vi "MC_8_27_12a_JW.vi"() -> ()   [LabVIEW 2011]
uses:
  <vilib>/Utility/file.llb/Read From Spreadsheet File (string).vi
  <vilib>/Utility/inputDevices.llb/keyboardAcquire.vi
  <vilib>/Utility/file.llb/Write To Spreadsheet File (DBL).vi
  <vilib>/Utility/file.llb/Write To Spreadsheet File (string).vi
  <vilib>/regexp/Match Regular Expression.xnode
panel:
  in  "Treatment Concentration (mM):":dbl=nan
  in  "Surface Treatment:":string="NaN"
  in  "# Drops*:":dbl=inf
  in  "Solution Temp (C):":dbl=nan
  in  "Relative Humidity (%):":dbl=nan
  in  "Room Temp (F):":dbl=nan
  in  "Time (s):":dbl=nan
  in  "RPM:":dbl=nan
  in  "Wait Time (s):":dbl=nan
  in  "Sample #:":dbl=1.0
  in  "Fabricator:":string="NaN"
  in  "Ramp (s):":dbl=3.0
  out "X Axis Display Type":string
  out "Opj X Axis":string
  in  "Room Temp":dbl=294.0
  out "No Image 2":path=path "\\\\acad1\\physics/Jurchescu-group/JW-PD/Image Not Found.png"
  out "Save1 Array":string[][](array[string])
  out "Lin Vd":dbl
  out "Lin-Vg Array-Used":dbl[](array[numeric])
  out "Lin Id-Used":dbl[](array[numeric])
  out "Rec: Comments":string
  out "Folder Index":dbl caption="Length"
  out "Current \nRecord":string[](array[string])
  out "Transformer \nHeaders":string[](array[string])
  out "Current Device ID":string
  out "Column":string
  out "Row":string
  out "Rec: Concentration":dbl
  out "Rec: Solvent":string
  out "Rec: Method":string
  in  "?":T1(tab)
  in  "Transport File":path
  out "Transport Folder":path
  out "Rec: Material":string
  out "Accel (RPM/s):":dbl
  in  "Transfer File":path
  out "Transfer Folder":path
  in  "Image Folder":path
  out "Image File":path=path "D:/UserData/Desktop/Jeremy/WFU/Research/Programs/VI mods/Image Not Found.png"
  in  "Manual Comments":bool
  in  "Comments:":string
  out "Calc: On/Off":dbl caption="On/Off-Sat" format="%#.2e"
  out "Calc: Off I-Sat":dbl caption="Off I-Sat" format="%#.2e"
  in  "Manuel-Dielectric":bool
  in  "Manuel-Length":bool
  out "Calc: VT-Lin":dbl
  out "New: VT-Lin":dbl
  out "Rec: VT-Lin":dbl caption="VT-Lin" format="%#_3g"
  out "Calc: Trap Density-STS":dbl format="%#.2e"
  out "New: Trap Density-STS":dbl format="%#.2e"
  out "Rec: Trap Density-STS":dbl caption="N-Sat (STS)" format="%#.2e"
  out "Calc: Trap Density-VT":dbl format="%#.2e"
  out "New: Trap Density-VT":dbl format="%#.2e"
  out "Rec: Trap Density-VT":dbl caption="N-Sat (VT)" format="%#.2e"
  out "Calc: Mobility-Lin":dbl format="%#.2e"
  out "New: Mobility-Lin":dbl format="%#_4e"
  out "Rec: Mobility-Lin":dbl caption="Mobility-Lin" format="%#_3e"
  out "Calc: Mobility-Sat":dbl format="%#.2e"
  out "Rec: Length":dbl caption="Length" format="%#_3g"
  out "Rec: Width":dbl caption="Width" format="%#_4g"
  out "Rec: Dielectric (d)":dbl caption="Dielectric (d)" format="%#_3g"
  in  "Cancel Button":bool
  in  "Up Button":bool
  in  "Down Button":bool
  out "Data Name:":string
  in  "Save Changes?":bool
  in  "New: Dielectric":dbl
  in  "New: Length":dbl
  in  "New: Width":dbl
  out "New: Mobility-Sat":dbl format="%#.2e"
  in  "Blank Button":bool
  in  "Zoom":i16(slide)=-3 scale=-5.0..5.0
  out "Image Out 2":T2(plugin-control)
  out "Image Out":T2(plugin-control)
  in  "Magnification":u16(ring) items=["5x", "10x", "20x", "50x", "80x"]
  out "Total Width":dbl
  out "Distances":dbl[](array[numeric])
  in  "Undo Button":bool
  in  "Remove Button":bool
  out "Rec: Mobility-Sat":dbl caption="Mobility-Sat" format="%#.2e"
  in  "Export":bool
  out "Calc: VT-Sat":dbl format="%#.2g"
  out "New: VT-Sat":dbl format="%#.2g"
  in  "Manual-Width":bool caption="Manual"
  out "Calc: STS":dbl format="%#.2g"
  out "New: STS":dbl format="%#.2g"
  out "Rec: VT-Sat":dbl caption="VT-Sat" format="%#.2g"
  out "Rec: STS":dbl caption="STS-Sat" format="%#.2g"
  out "Rec: On/Off":dbl caption="On/Off-Sat" format="%#.2e"
  in  "Save Changes? 2":bool
  in  "Save Changes? 3":bool
  out "Rec: Temp":dbl caption="Sample Temp" format="%.1f"
  in  "New: Temp":dbl format="%.1f"
  out "Rec: Off I-Sat":dbl caption="Off I-Sat" format="%#.2e"
  in  "Independant Variable":string(combo)="Length (um):"
  in  "Transfer Plots":enum32{"Linear", "Saturation", "Raw"}(tab)=enum."Saturation"
  in  "Lin-Trans Slider":dbl(slide) step=1.0 scale=-22.0..89.0 scale format="%#_1p"
  out "Sqrt-Lin":cluster{dbl[], dbl[]}[](graph)
  in  "Next Sqrt Lin":bool
  in  "Previous Sqrt Lin":bool
  in  "Sat-Trans Slider":dbl(slide) step=1.0 scale=-22.0..89.0 scale format="%#_1p"
  out "Sqrt-Sat":cluster{dbl[], dbl[]}[](graph)
  in  "Previous Sqrt Sat":bool
  in  "Next Sqrt Sat":bool
  out "Sqrt-Raw":cluster{dbl[], dbl[]}[](graph)
  in  "Log Plots":enum32{"Linear", "Saturation", "Raw"}(tab)=enum."Saturation"
  in  "Lin-Log Slider":dbl(slide) step=1.0 scale=-1.0..82.0 scale format="%#_1p"
  in  "Previous Log Lin":bool
  in  "Next Log Lin":bool
  out "Log-Lin":cluster{dbl[], dbl[]}[](graph)
  in  "Sat-Log Slider":dbl(slide) step=1.0 scale=-1.0..82.0 scale format="%#_1p"
  out "Log-Sat":cluster{dbl[], dbl[]}[](graph)
  in  "Previous Log Sat":bool
  in  "Next Log Sat":bool
  out "Raw-Log":cluster{dbl[], dbl[]}[](graph)
  in  "Manual-Temp":bool caption="Manual"
  out "Date Created":string caption="Fabricated"
  out "Date Recorded":string="Date Recorded" caption="Measured"
  out "Image Name":string
  out "Index":string
  in  "Num Pts":dbl=5.0
  in  "NumPoints Log":dbl=5.0 caption="Num Pts"
  in  "Origin Project File":path=path "\\\\acad1\\physics/Jurchescu-group/JW-PD/Group Library/Origin Project Files/DeviceData_8_10_12a_JW.opj"
  in  "No Image File":path=path "\\\\acad1\\physics/Jurchescu-group/JW-PD/Mega Awesome/Image Not Found.png"
  out "String":string
  out "Index 2":dbl
  out "Sat Id-Log-Used":dbl[](array[numeric])
  out "Vg Array-Log-Used":dbl[](array[numeric])
  out "ROI Descriptor out":T3 {"Contours"."Type" items=["No Selection", "Point", "Line", "Rectangle", "Oval", "Polygon", "Freehand Region", "Annulus", "Unused2", "Unused3", "Broken Line", "Freehand Line", "Rotated Rectangle"]}
  out "ROI Descriptor":T3 {"Contours"."Type" items=["No Selection", "Point", "Line", "Rectangle", "Oval", "Polygon", "Freehand Region", "Annulus", "Unused2", "Unused3", "Broken Line", "Freehand Line", "Rotated Rectangle"]}
  out "Numeric 3":dbl
  out "Array 6":dbl[][](array[numeric])
  out "Cluster":T4
  out "Array 5":dbl[](array[numeric])
  out "Array 4":dbl[](array[numeric])
  out "Array 3":dbl[](array[numeric])
  out "Numeric 2":dbl
  out "Numeric":dbl
  out "Sat Id-Used":dbl[](array[numeric])
  out "Sat Vg Array-Used":dbl[](array[numeric])
  out "MobVi Index":dbl
  in  "Row Start":dbl=20.0
  # "Sample Properties"
  # "*     Inf = Full coverage\n   NaN = Unknown or Not Applicable"
  # "Data Locations"
  # "Transport Location"
  # "Transfer Location"
  # "Image Location"
  # "Recorded"
  # "Calculated"
  # "Re-Calculated"
  # "Manual"
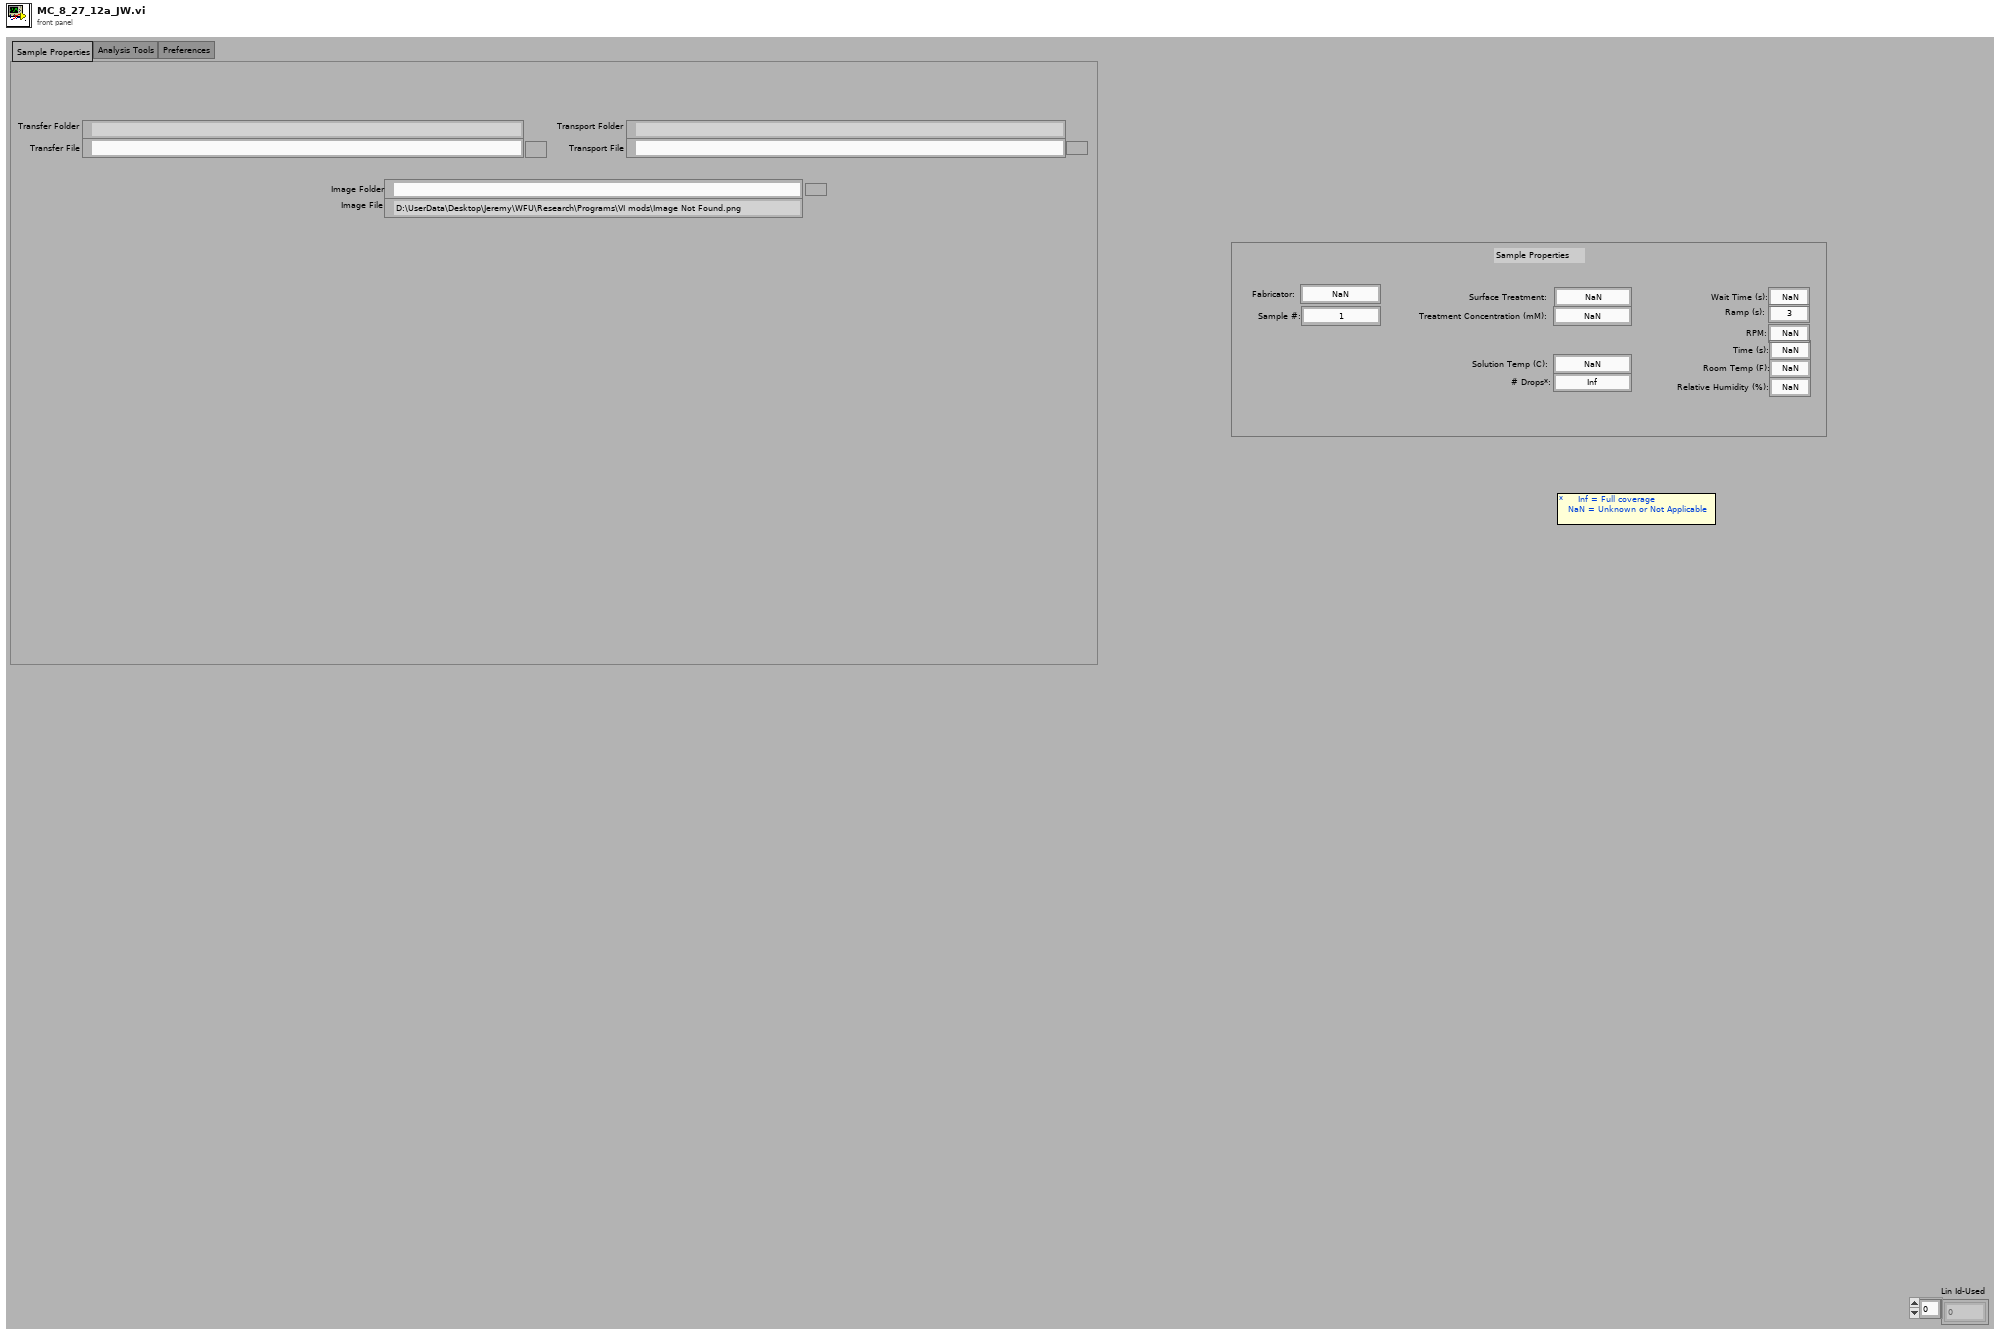
[diagram p1: front panel]
types:
  T1 = enum32{"Sample Properties", "Analysis Tools", "Preferences", "Current Database"}
  T2 = typedef "IMAQ Image.ctl" = refnum<image>
  T3 = typedef "ROI Descriptor" = cluster{"Global Rectangle":i32[], "Contours":cluster{"ID":enum32{"External", "Internal"}, "Type":u32, "Coordinates":i32[]}[]}
  T4 = cluster{"Numeric":dbl, "Numeric 2":dbl, "Numeric 3":dbl, "Numeric 4":dbl}
  T5 = cluster{"Mobility-Sat":dbl, "Moblitity-Lin":dbl, "On/Off":dbl, "Off Current":dbl, "Vt-Sat":dbl, "STS":dbl, "Trap Density-VT":dbl, "Trap Density-STS":dbl}
  T6 = cluster{"Date Recorded":string, "Index":string, "Length":dbl, "Width":dbl, "Sample Temp":dbl}
  T7 = cluster{"Date Created":string, "Material":string, "Solvent":string, "Concentration":dbl, "Method":string, "Dielectric (nm)":dbl, "Treatment":string, "Comments":string}
  T8 = cluster{"Raw Sat":cluster{dbl[], dbl[]}[], "Sqrt Sat":cluster{dbl[], dbl[]}[], "Log Sat":cluster{dbl[], dbl[]}, "Raw Lin":cluster{dbl[], dbl[]}[], "Sqrt Lin":cluster{dbl[], dbl[]}[], "Log Lin":cluster{dbl[], dbl[]}[]}
  T9 = cluster{"Mobility-Sat":dbl, "Vt-Sat":dbl, "Mobility-Lin":dbl, "Vt-Lin":dbl, "Off I-Sat":dbl, "On/Off I-Sat":dbl}
  T10 = cluster{"[0]":cluster{dbl[], dbl[]}, "[1]":cluster{dbl[], dbl[]}, "[2]":cluster{dbl[], dbl[]}, "[3]":cluster{dbl[], dbl[]}, "[4]":cluster{dbl[], dbl[]}, "[5]":cluster{dbl[], dbl[]}, "[6]":cluster{dbl[], dbl[]}, "[7]":cluster{dbl[], dbl[]}, "[8]":cluster{dbl[], dbl[]}}
  T11 = cluster{"Global Rectangle":i32[], "Contours":cluster{"Contour Type":u32, "ROI Type":u32, "Points":i32[]}[]}
  T12 = typedef "LVBoundsTypeDef.ctl" = cluster{"Width":u32, "Height":u32}
  T13 = enum16{"0", "1", "2", "3", "4", "5", "6", "7", "8", "9", "A", "B", "C", "D", "E", "F", "G", "H", "I", "J", "K", "L", "M", "N", "O", "P", "Q", "R", "S", "T", "U", "V", "W", "X", "Y", "Z", "F1", "F2", "F3", "F4", "F5", "F6", "F7", "F8", "F9", "F10", "F11", "F12", "F13", "F14", "F15", "ADD", "BACK", "BACKSLASH", "CAPITAL", "COMMA", "DECIMAL", "DELETE", "DIVIDE", "DOWN", "END", "EQUALS", "ESCAPE", "GRAVE (`)", "HOME", "INSERT", "LBRACKET", "LCONTROL", "LEFT", "L ALT", "LSHIFT", "LWIN", "MINUS", "MULTIPLY", "NEXT", "NUMLOCK", "NUMPAD_0", "NUMPAD_1", "NUMPAD_2", "NUMPAD_3", "NUMPAD_4", "NUMPAD_5", "NUMPAD_6", "NUMPAD_7", "NUMPAD_8", "NUMPAD_9", "PAUSE", "PERIOD", "PRIOR (PG UP)", "RBRACKET", "RCONTROL", "RETURN", "RIGHT", "R ALT", "RSHIFT", "RWIN", "SCROLL", "SEMICOLON", "SLASH", "SPACE", "SUBTRACT", "TAB", "UP", "ENTER (num pad)", "' (quote)"}[]
  T14 = enum16{"0", "1", "2", "3", "4", "5", "6", "7", "8", "9", "A", "B", "C", "D", "E", "F", "G", "H", "I", "J", "K", "L", "M", "N", "O", "P", "Q", "R", "S", "T", "U", "V", "W", "X", "Y", "Z", "F1", "F2", "F3", "F4", "F5", "F6", "F7", "F8", "F9", "F10", "F11", "F12", "F13", "F14", "F15", "ADD", "BACK", "BACKSLASH", "CAPITAL", "COMMA", "DECIMAL", "DELETE", "DIVIDE", "DOWN", "END", "EQUALS", "ESCAPE", "GRAVE (`)", "HOME", "INSERT", "LBRACKET", "LCONTROL", "LEFT", "L ALT", "LSHIFT", "LWIN", "MINUS", "MULTIPLY", "NEXT", "NUMLOCK", "NUMPAD_0", "NUMPAD_1", "NUMPAD_2", "NUMPAD_3", "NUMPAD_4", "NUMPAD_5", "NUMPAD_6", "NUMPAD_7", "NUMPAD_8", "NUMPAD_9", "PAUSE", "PERIOD", "PRIOR (PG UP)", "RBRACKET", "RCONTROL", "RETURN", "RIGHT", "R ALT", "RSHIFT", "RWIN", "SCROLL", "SEMICOLON", "SLASH", "SPACE", "SUBTRACT", "TAB", "UP", "ENTER (num pad)", "' (quote)"}
  T15 = cluster{"Contour Type":u32, "ROI Type":u32, "Points":i32[]}[]
  T16 = cluster{i32[], cluster{"Contour Type":u32, "ROI Type":u32, "Points":i32[]}[]}
  T17 = cluster{"Independant  Variable Indicator":string, "Parameter String Indicator":string}
  T18 = cluster{string, sgl, bool, bool, bool, bool, bool, bool, i32}
  T19 = cluster{i32, cluster{string, sgl, bool, bool, bool, bool, bool, bool, i32}, i32, i32}
  T20 = cluster{"Contour Type":u32, "ROI Type":u32, "Points":i32[]}
  T21 = cluster{"Points[0]":i32, "Points[1]":i32, "Points[2]":i32, "Points[3]":i32, "Points[4]":i32, "Points[5]":i32, "Points[6]":i32, "Points[7]":i32, "Points[8]":i32}
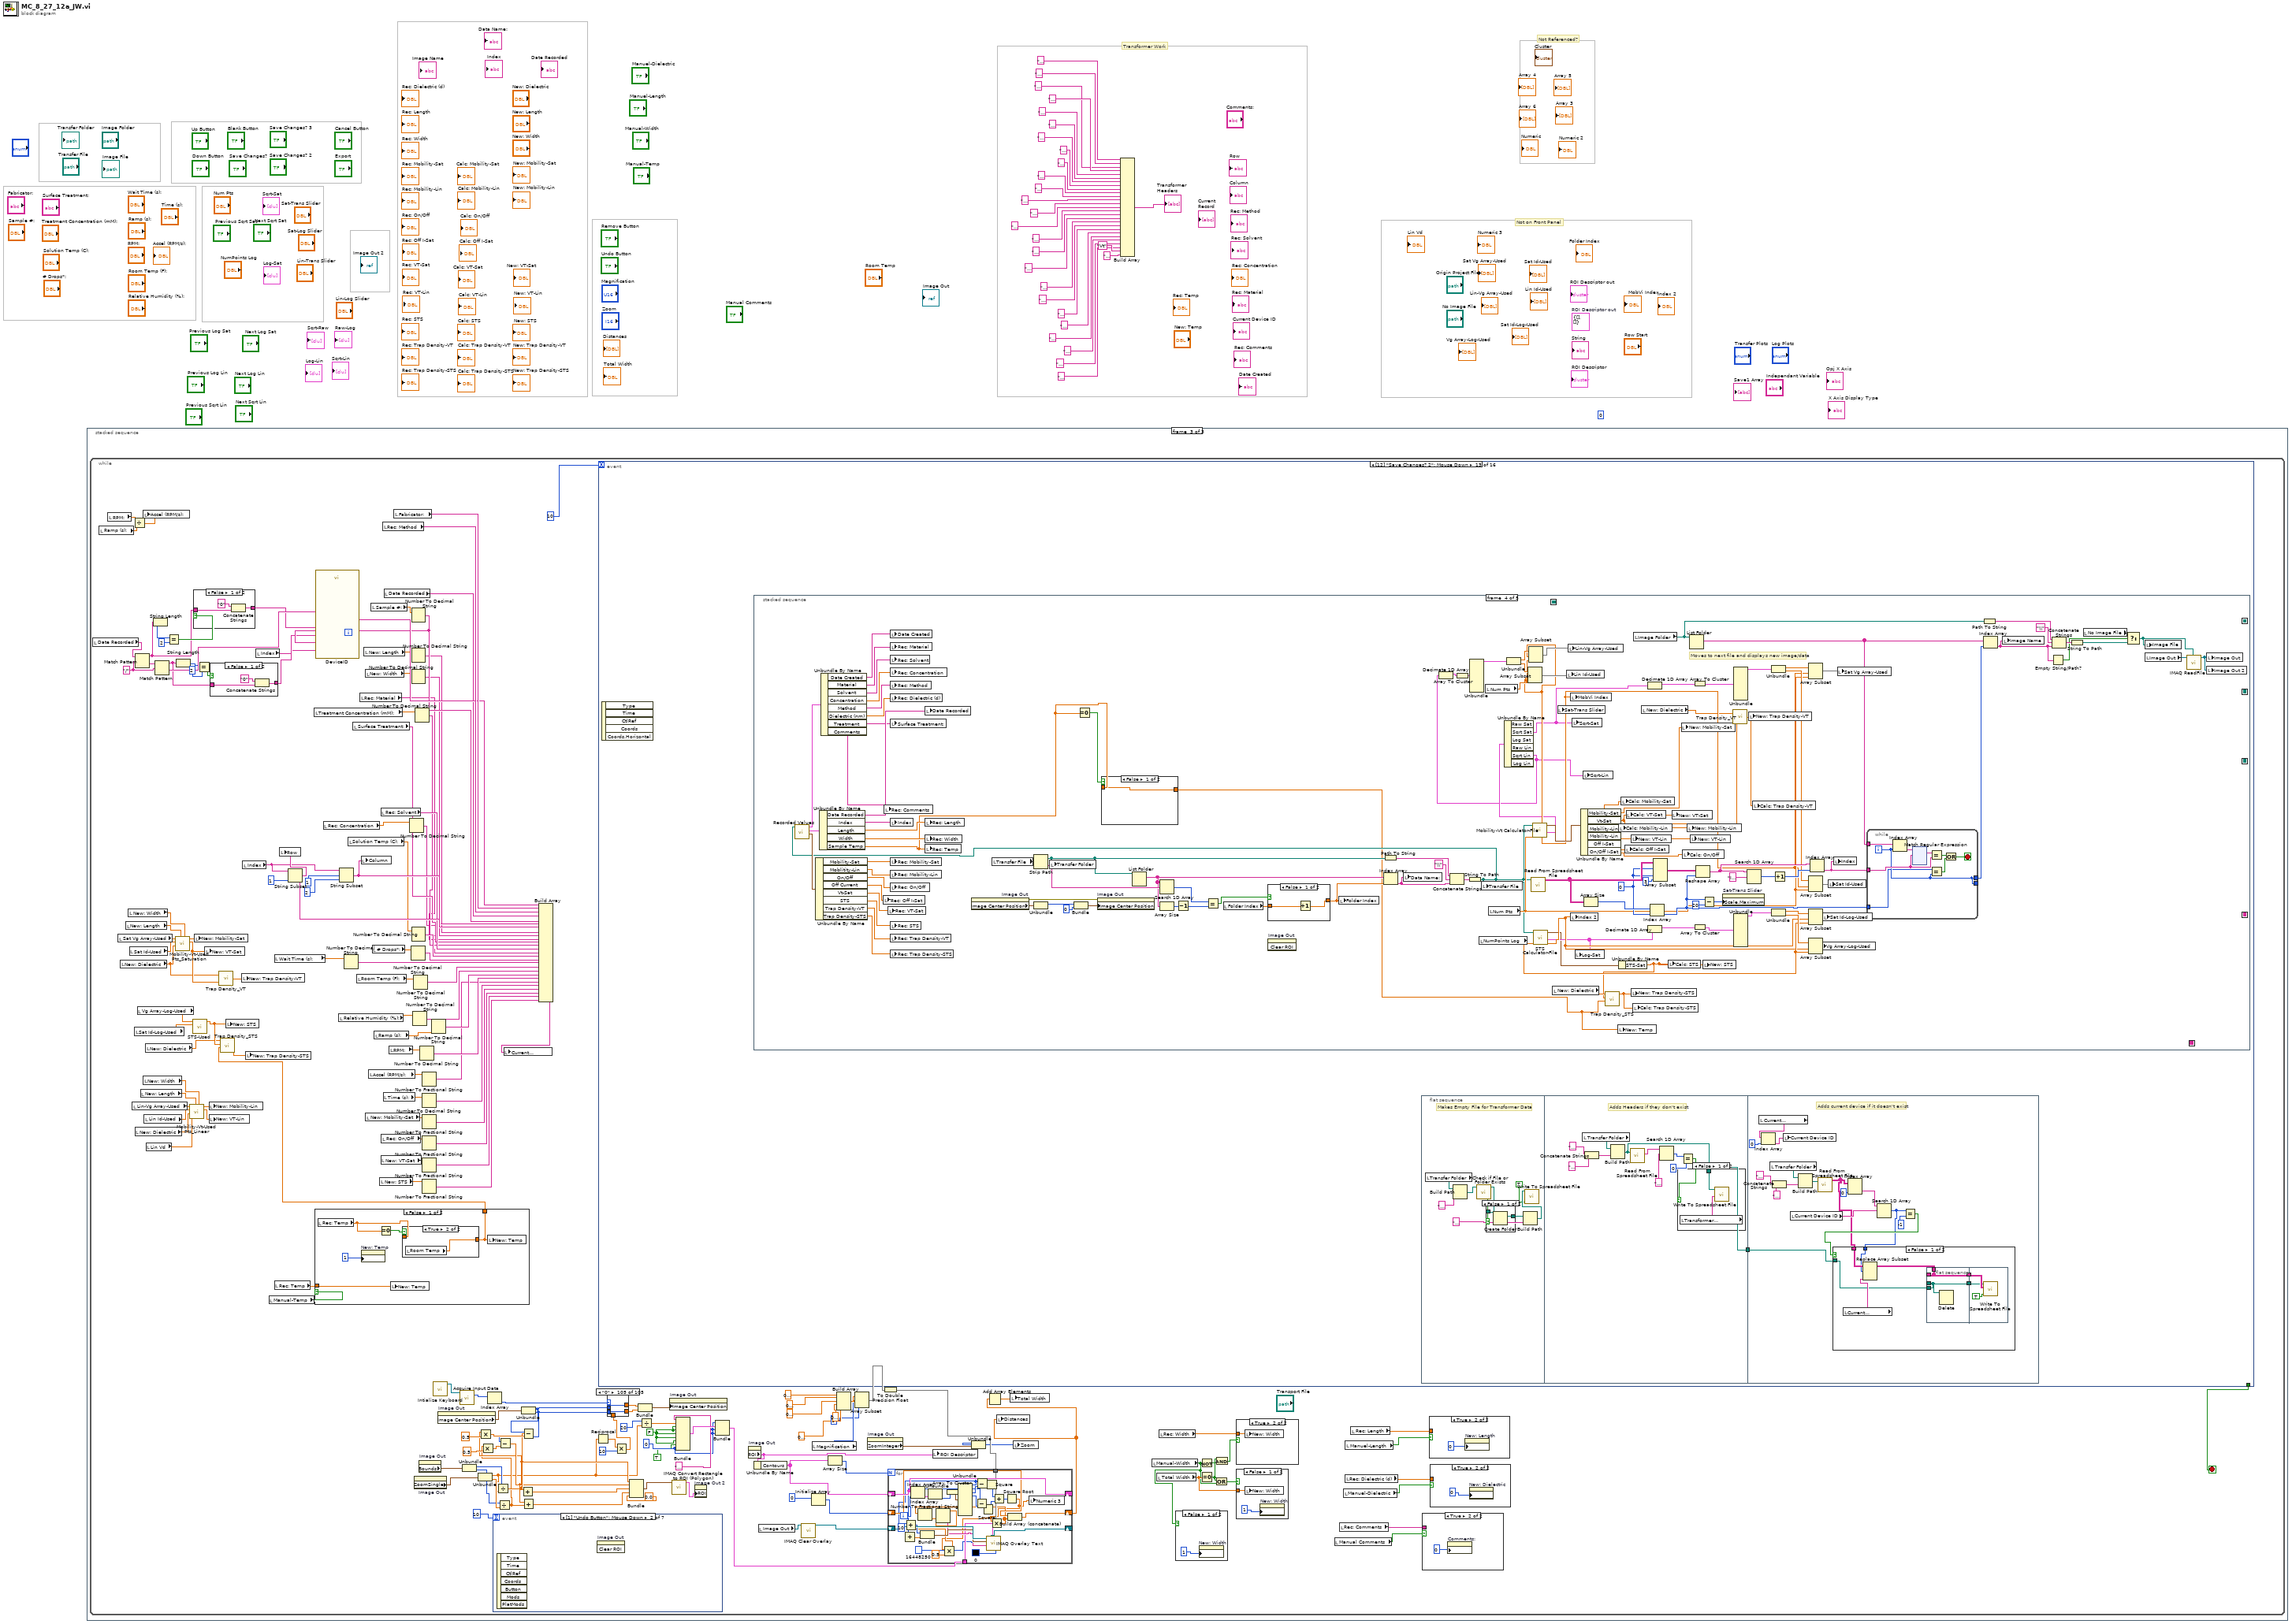
[diagram p0: block diagram]
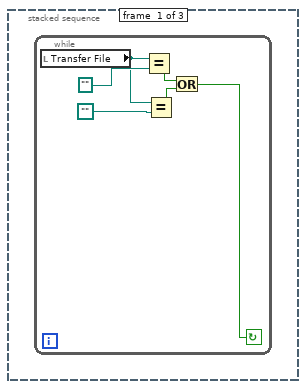
[diagram p2: hidden frame]
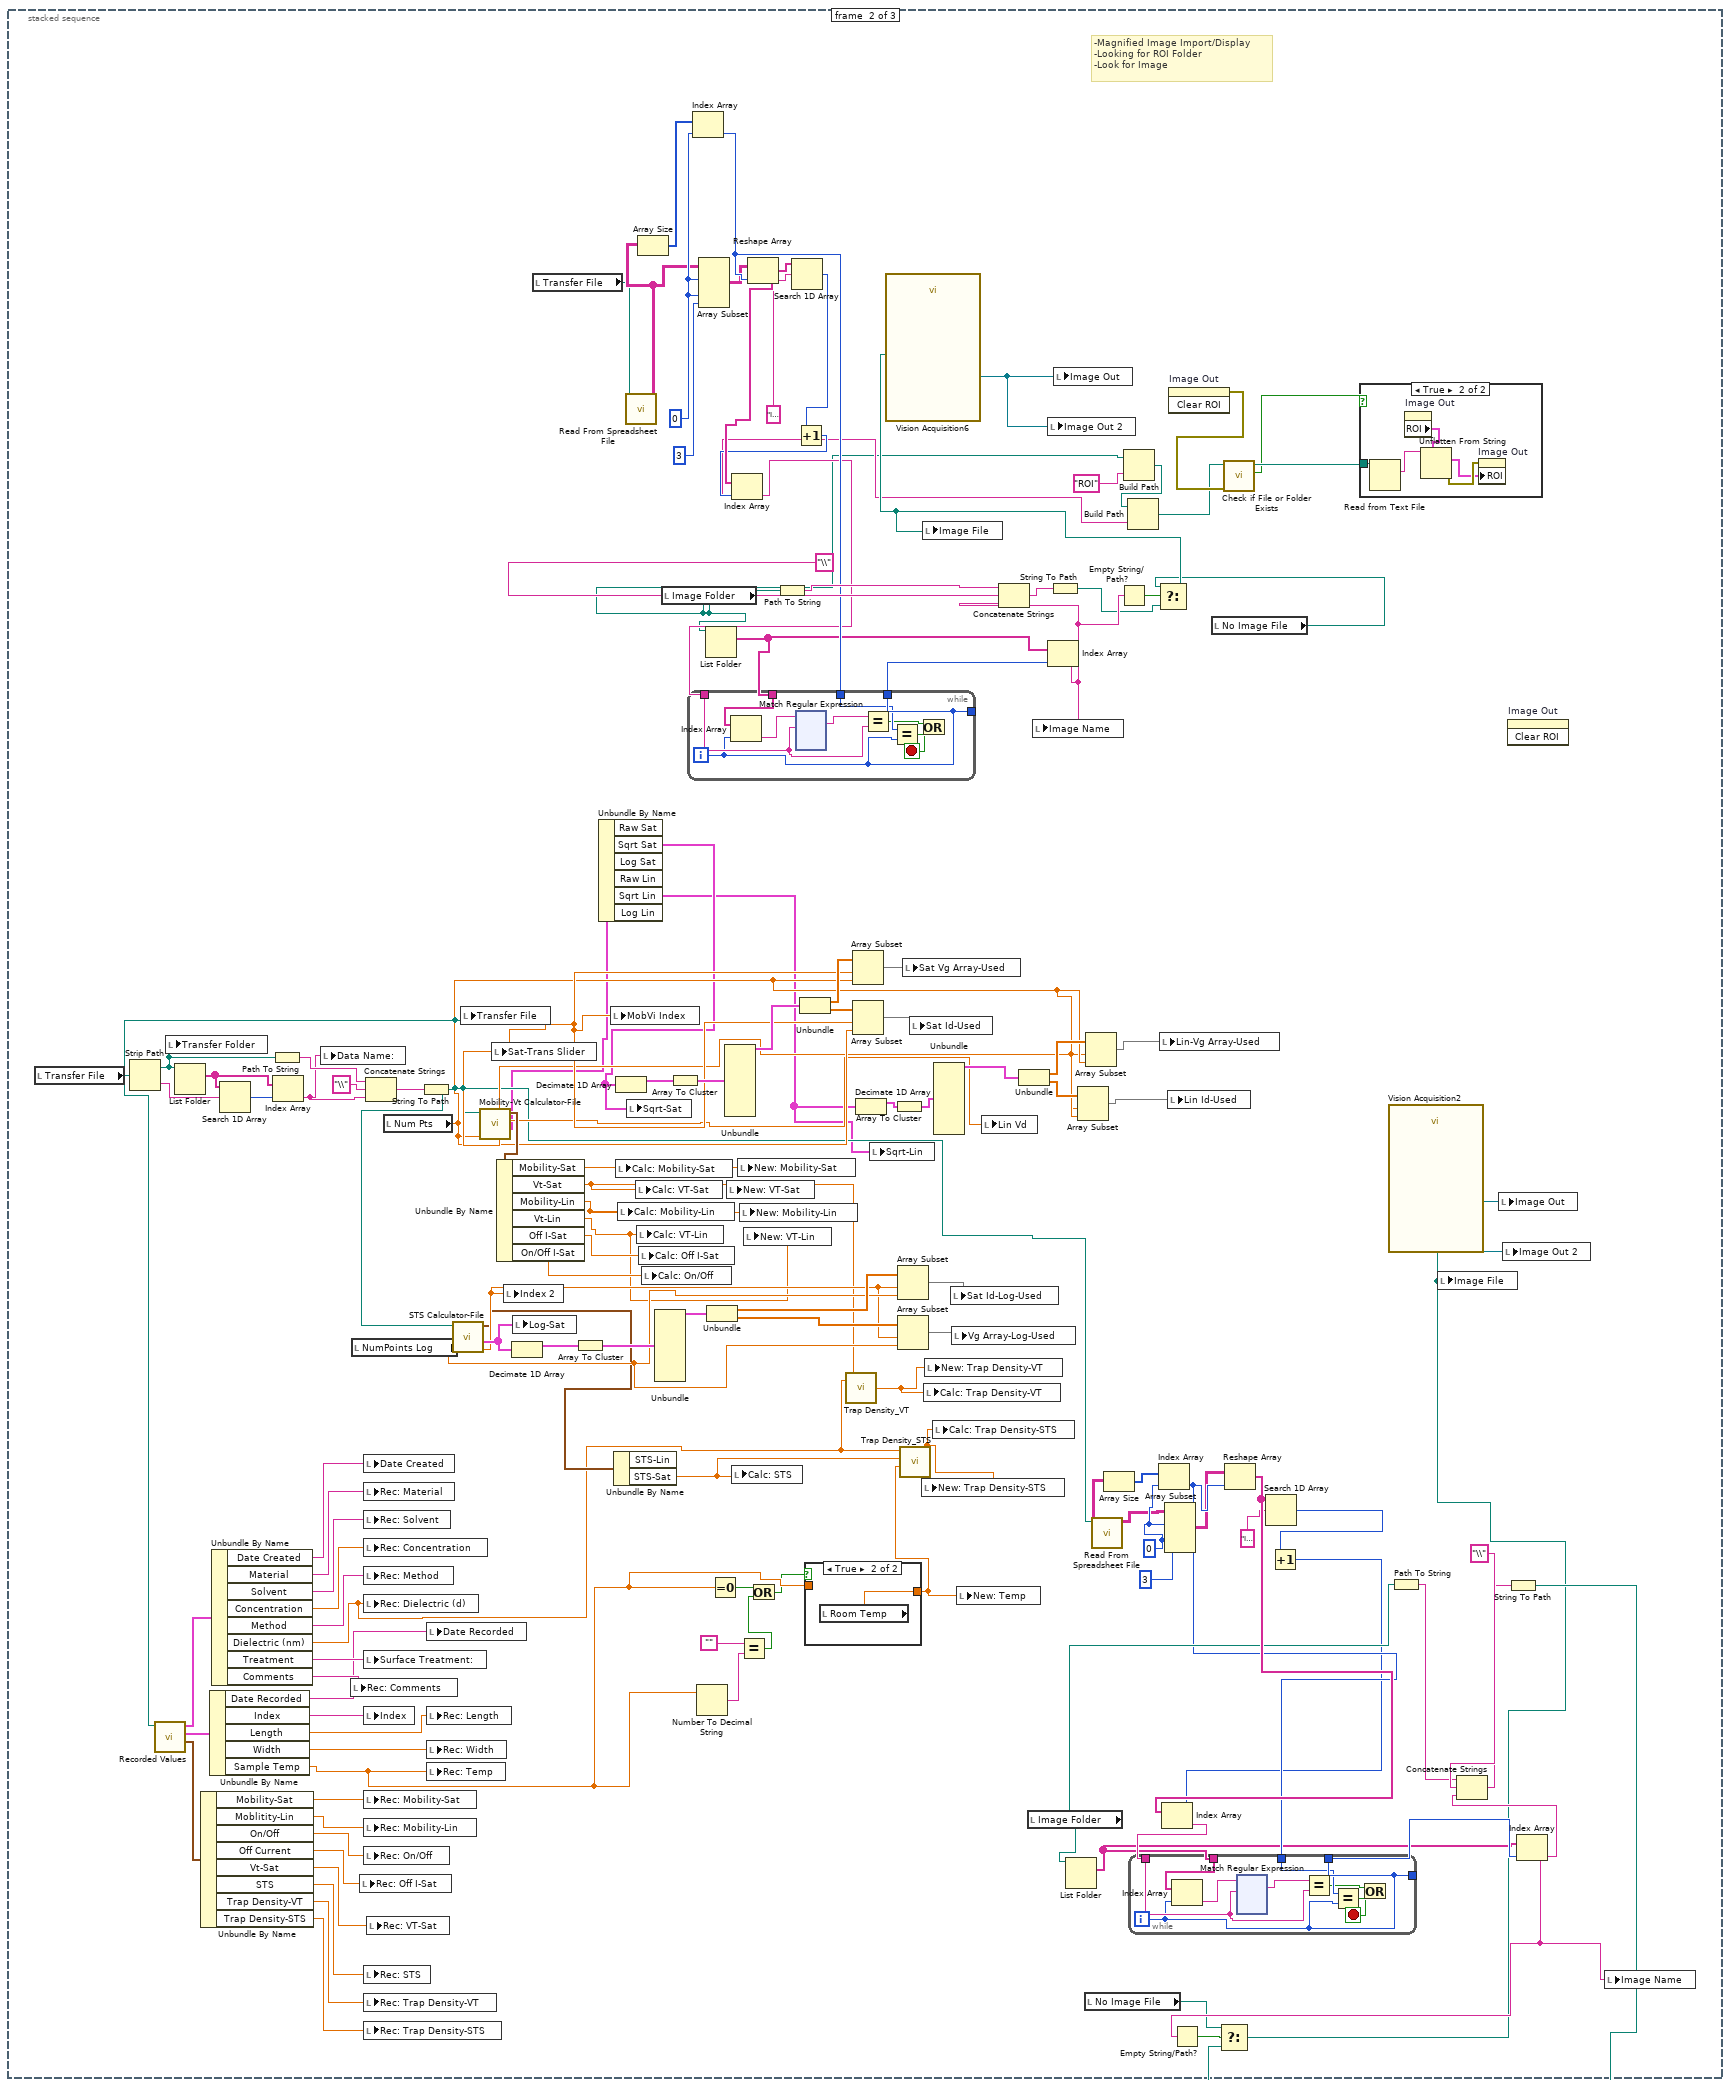
[diagram p3: hidden frame]
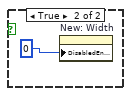
[diagram p6: hidden frame]
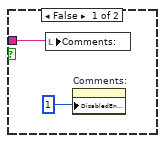
[diagram p7: hidden frame]
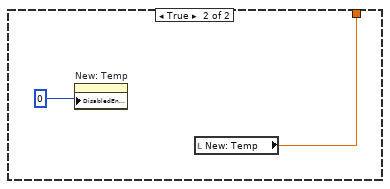
[diagram p9: hidden frame]
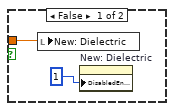
[diagram p10: hidden frame]
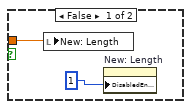
[diagram p11: hidden frame]
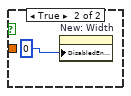
[diagram p15: hidden frame]
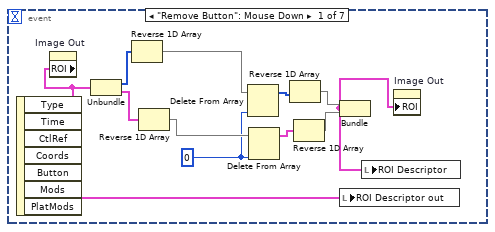
[diagram p16: hidden frame]
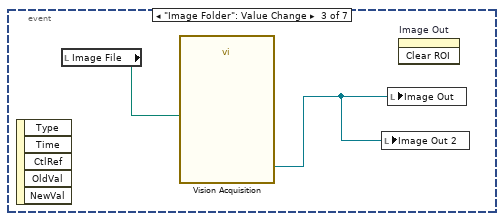
[diagram p17: hidden frame]
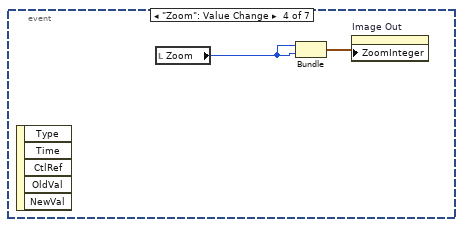
[diagram p18: hidden frame]
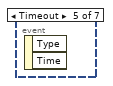
[diagram p19: hidden frame]
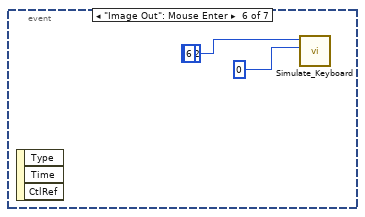
[diagram p20: hidden frame]
diagram:
  (unwired) 0
  (unwired) T3 {"Global Rectangle"=[], "Contours"=[]}  # ROI Descriptor out
  # "Not Referenced?"
  # "Transformer Work"
  # "Not on Front Panel"
  n1 = stacked-sequence {
    frame #0 {
      n2 = while {
        stop <- w29 continue-if-true
        n3 = local read "Transfer File"() -> (w31:path)
        n4 = Equal?(x=w31, y=path "") -> (x = y?=w33:bool)
        n5 = Equal?(x=w31, y=path "") -> (x = y?=w32:bool)
        n6 = Or(x=w33, y=w32) -> (x .or. y?=w29:bool)
      }
    }
    frame #1 {
      w134 = 0
      w158 = 0
      # "-Magnified Image Import/Display\n-Looking for ROI Folder\n-Look for Image"
      n7 = local read "Transfer File"() -> (w138:path)
      n8 = Strip Path(path=w138) -> (stripped path=w139:path, name=w125:string)
      n9 = local write "Transfer Folder"(w139) -> ()
      n10 = List Folder(path=w139) -> (filenames=w129:string[])  [unwired: 3 in, 3 out]
      n11 = Search 1D Array(1D array=w129, element=w125) -> (index of element=w128:i32)  [unwired: 1 in]
      n12 = Path To String(path=w139) -> (string=w124:string)
      n13 = Index Array(array=w129, index=w128) -> (element=w94:string)
      n14 = local write "Data Name:"(w94) -> ()
      n15 = local read "NumPoints Log"() -> (w70:dbl)
      n16 = Concatenate Strings(w124, "\\", w94) -> (w126:string)
      n17 = local read "Num Pts"() -> (w61:dbl)
      n18 = String To Path(string=w126) -> (path=w55:path)
      n19 = call "Recorded Values.vi"("Path"=w55) -> ("Recorded Char"=w92:T5, "Recorded Prop"=w91:T6, "Fabrication Prop"=w93:T7)  [unwired: 8 in]
      n20 = Unbundle By Name(w92) -> ("Mobility-Sat"=w80:dbl, "Moblitity-Lin"=w79:dbl, "On/Off"=w78:dbl, "Off Current"=w77:dbl, "Vt-Sat"=w41:dbl, "STS"=w76:dbl, "Trap Density-VT"=w75:dbl, "Trap Density-STS"=w74:dbl)
      n21 = Unbundle By Name(w91) -> ("Date Recorded"=w84:string, "Index"=w83:string, "Length"=w82:dbl, "Width"=w81:dbl, "Sample Temp"=w47:dbl)
      n22 = Unbundle By Name(w93) -> ("Date Created"=w73:string, "Material"=w90:string, "Solvent"=w89:string, "Concentration"=w88:dbl, "Method"=w87:string, "Dielectric (nm)"=w51:dbl, "Treatment"=w86:string, "Comments"=w85:string)
      n23 = local write "Rec: Comments"(w85) -> ()
      n24 = local write "Rec: Off I-Sat"(w77) -> ()
      n25 = local write "Date Created"(w73) -> ()
      n26 = local write "Rec: Material"(w90) -> ()
      n27 = local write "Rec: Solvent"(w89) -> ()
      n28 = local write "Rec: Concentration"(w88) -> ()
      n29 = local write "Rec: Method"(w87) -> ()
      n30 = local write "Rec: Dielectric (d)"(w51) -> ()
      n31 = local write "Surface Treatment:"(w86) -> ()
      n32 = local write "Index"(w83) -> ()
      n33 = local write "Rec: Mobility-Sat"(w80) -> ()
      n34 = local write "Rec: Mobility-Lin"(w79) -> ()
      n35 = local write "Rec: On/Off"(w78) -> ()
      n36 = local write "Rec: STS"(w76) -> ()
      n37 = local write "Rec: Trap Density-VT"(w75) -> ()
      n38 = local write "Rec: Trap Density-STS"(w74) -> ()
      n39 = local write "Rec: VT-Sat"(w41) -> ()
      n40 = local write "Date Recorded"(w84) -> ()
      n41 = local write "Rec: Length"(w82) -> ()
      n42 = local write "Rec: Width"(w81) -> ()
      n43 = local write "Rec: Temp"(w47) -> ()
      n44 = call "STS Calculator-File.vi"("NumPts"=w70, "Path"=w55) -> ("STS Index-Sat"=w68:dbl, "XY Graph-Sat"=w69:cluster{dbl[], dbl[]}[], "Ouput"=w67:cluster{"STS-Sat":dbl, "STS-Lin":dbl})  [unwired: 5 in, 2 out]
      n45 = local write "Transfer File"(w55) -> ()
      n46 = call "Mobility-Vt Calculator-File.vi"("NumPts"=w61, "Path"=w55) -> ("Graph Cluster"=w37:T8, "Lin Vd"=w57:dbl, "Output"=w72:T9, "Index-Sat"=w71:dbl, "Index-Lin"=w60:dbl)  [unwired: 5 in]
      n47 = local write "Sat-Trans Slider"(w71) -> ()
      n48 = Unbundle By Name(w72) -> ("Mobility-Sat"=w50:dbl, "Vt-Sat"=w49:dbl, "Mobility-Lin"=w40:dbl, "Vt-Lin"=w38:dbl, "Off I-Sat"=w56:dbl, "On/Off I-Sat"=w39:dbl)
      n49 = local write "Index 2"(w68) -> ()
      n50 = Decimate 1D Array(w69) -> (w116:cluster{dbl[], dbl[]}[])  [unwired: 1 out]
      n51 = local write "Log-Sat"(w69) -> ()
      n52 = local read "Transfer File"() -> (w153:path)
      n53 = Array To Cluster(array=w116) -> (cluster=w118:T10)
      n54 = Unbundle By Name(w37) -> ("Sqrt Sat"=w36:cluster{dbl[], dbl[]}[], "Sqrt Lin"=w35:cluster{dbl[], dbl[]}[])  [unwired: 4 out]
      n55 = local write "MobVi Index"(w71) -> ()
      n56 = Unbundle By Name(w67) -> ("STS-Sat"=w54:dbl)  [unwired: 1 out]
      n57 = Decimate 1D Array(w36) -> (w152:cluster{dbl[], dbl[]}[])  [unwired: 1 out]
      n58 = local write "Calc: Mobility-Sat"(w50) -> ()
      n59 = local write "Calc: Mobility-Lin"(w40) -> ()
      n60 = call-poly <vilib>:"Read From Spreadsheet File.vi"("file path (dialog if empty)"=w153) -> ("all rows"=w156:string[][])  [unwired: 6 in, 4 out]
      n61 = local write "Sqrt-Sat"(w36) -> ()
      n62 = local write "Calc: VT-Sat"(w49) -> ()
      n63 = local write "Calc: VT-Lin"(w38) -> ()
      n64 = Array Size(array=w156) -> (size(s)=w157:i32[])
      n65 = local write "Calc: Off I-Sat"(w56) -> ()
      n66 = local write "Calc: On/Off"(w39) -> ()
      n67 = Unbundle(w118) -> ("[0]"=w117:cluster{dbl[], dbl[]})  [unwired: 8 out]
      n68 = local read "Image Folder"() -> (w95:path)
      n69 = Array To Cluster(array=w152) -> (cluster=w150:T10)
      n70 = Index Array(array=w157, index=w158) -> (element=w164:i32)
      n71 = Number To Decimal String(number=w47) -> (decimal integer string=w45:string)  [unwired: 1 in]
      n72 = Array Subset(array=w156, index (row)=w158, index (col)=w158, length (col)=3) -> (w155:string[][])  [unwired: 1 in]
      n73 = List Folder(path=w95) -> (filenames=w162:string[])  [unwired: 3 in, 3 out]
      n74 = Unbundle(w117) -> (w114:dbl[], w113:dbl[])
      n75 = Equal To 0?(x=w47) -> (x = 0?=w46:bool)
      n76 = Unbundle(w150) -> ("[0]"=w151:cluster{dbl[], dbl[]})  [unwired: 8 out]
      n77 = local write "New: VT-Sat"(w49) -> ()
      n78 = local write "Calc: STS"(w54) -> ()
      n79 = local write "New: Mobility-Sat"(w50) -> ()
      n80 = Equal?(x="", y=w45) -> (x = y?=w43:bool)
      n81 = local write "New: Mobility-Lin"(w40) -> ()
      n82 = local write "New: VT-Lin"(w38) -> ()
      n83 = Reshape Array(w155, w164) -> (w169:string[])
      n84 = Or(x=w46, y=w43) -> (x .or. y?=w42:bool)
      n85 = Path To String(path=w95) -> (string=w166:string)
      n86 = Search 1D Array(1D array=w169, element="Index:") -> (index of element=w161:i32)  [unwired: 1 in]
      n87 = Increment(x=w161) -> (x+1=w160:i32)
      n88 = Index Array(array=w169, index=w160) -> (element=w96:string)
      n89 = while {
        tunnel: w162 -> [w304]
        tunnel: w96 -> [w302]
        tunnel: [w301] -> _
        tunnel: [w301] -> w163
        tunnel: w164 -> [w300]
        i -> [w301]
        stop <- w297 stop-if-true
        n90 = Index Array(array=w304, index=w301) -> (element=w305:string)
        n91 = xnode "Match Regular Expression"("input string"=w305, "regular expression"=w302) -> ("whole match"=w303:string)  [unwired: 4 in, 4 out]
        n92 = Equal?(x=w303, y=w302) -> (x = y?=w299:bool)
        n93 = Equal?(x=w300, y=w301) -> (x = y?=w298:bool)
        n94 = Or(x=w299, y=w298) -> (x .or. y?=w297:bool)
      }
      n95 = Unbundle(w151) -> (w115:dbl[], w119:dbl[])
      n96 = case shown="True" w42 {
        tunnel: [w170 w171] -> w53
        tunnel: w47 -> [w170 _]
        frame False {
        }
        frame True {
          n97 = local read "Room Temp"() -> (w171:dbl)
        }
      }
      n98 = call "Trap Density_VT.vi"("VT"=w49, "Dielectric"=w51) -> ("Trap Density-VT"=w48:dbl)
      n99 = Array Subset(array=w115, index=w71, length=w61) -> (w122:dbl[])
      n100 = Array Subset(array=w119, index=w71, length=w61) -> (w123:dbl[])
      n101 = Decimate 1D Array(w35) -> (w66:cluster{dbl[], dbl[]}[])  [unwired: 1 out]
      n102 = local write "Sqrt-Lin"(w35) -> ()
      n103 = Array To Cluster(array=w66) -> (cluster=w65:T10)
      n104 = Array Subset(array=w114, index=w68, length=w70) -> (w121:dbl[])
      n105 = Array Subset(array=w113, index=w68, length=w70) -> (w120:dbl[])
      n106 = call "Trap Density_STS.vi"("Temp (T) [K]"=w53, "S.T.S. (S)"=w54, "Dielectric"=w51) -> ("Trap Density (N)"=w52:dbl)  [unwired: 8 in]
      n107 = local write "Sat Vg Array-Used"(w122) -> ()
      n108 = local write "Sat Id-Used"(w123) -> ()
      n109 = local write "New: Trap Density-STS"(w52) -> ()
      n110 = local write "Calc: Trap Density-VT"(w48) -> ()
      n111 = local write "New: Trap Density-VT"(w48) -> ()
      n112 = local write "Calc: Trap Density-STS"(w52) -> ()
      n113 = Unbundle(w65) -> ("[0]"=w64:cluster{dbl[], dbl[]})  [unwired: 8 out]
      n114 = local write "Sat Id-Log-Used"(w121) -> ()
      n115 = local write "Vg Array-Log-Used"(w120) -> ()
      n116 = local write "New: Temp"(w53) -> ()
      n117 = local write "Lin Vd"(w57) -> ()
      n118 = Unbundle(w64) -> (w63:dbl[], w62:dbl[])
      n119 = local read "Image Folder"() -> (w145:path)
      n120 = Index Array(array=w162, index=w163) -> (element=w112:string)
      n121 = Concatenate Strings(w166, "\\", w112) -> (w167:string)
      n122 = local write "Image Name"(w112) -> ()
      n123 = String To Path(string=w167) -> (path=w110:path)
      n124 = List Folder(path=w145) -> (filenames=w141:string[])  [unwired: 3 in, 3 out]
      n125 = Array Subset(array=w62, index=w60, length=w61) -> (w58:dbl[])
      n126 = local read "No Image File"() -> (w104:path)
      n127 = Array Subset(array=w63, index=w60, length=w61) -> (w59:dbl[])
      n128 = call-poly <vilib>:"Read From Spreadsheet File.vi"("file path (dialog if empty)"=w55) -> ("all rows"=w132:string[][])  [unwired: 6 in, 4 out]
      n129 = Array Size(array=w132) -> (size(s)=w133:i32[])
      n130 = Empty String/Path?(string/path=w112) -> (empty?=w111:bool)
      n131 = Build Path(base path=w95, name or relative path="ROI") -> (appended path=w98:path)
      n132 = Build Path(base path=w98, name or relative path=w96) -> (appended path=w97:path)
      n133 = Index Array(array=w133, index=w134) -> (element=w144:i32)
      n134 = local write "Lin-Vg Array-Used"(w59) -> ()
      n135 = Array Subset(array=w132, index (row)=w134, index (col)=w134, length (col)=3) -> (w131:string[][])  [unwired: 1 in]
      n136 = local write "Lin Id-Used"(w58) -> ()
      n137 = invoke on="Image Out" class="ImageControl" method="Clear ROI"() -> (error out=w102:errorcluster)  [unwired: 3 in, 2 out]
      n138 = local read "No Image File"() -> (w103:path)
      n139 = Select(t=w103, s=w111, f=w110) -> (s? t:f=w109:path)
      n140 = call "Vision Acquisition6"("Image Path"=w109) -> ("Image Out"=w165:T2)  [unwired: 25 in, 1 out]
      n141 = local write "Image File"(w109) -> ()
      n142 = local write "Image Out 2"(w165) -> ()
      n143 = local write "Image Out"(w165) -> ()
      n144 = call <vilib>:"Check if File or Folder Exists.vi"("error in (no error)"=w102, "path"=w97) -> ("file or folder exists?"=w100:bool, "dup path"=w101:path)  [unwired: 7 in, 1 out]
      n145 = Reshape Array(w131, w144) -> (w149:string[])
      n146 = Search 1D Array(1D array=w149, element="Index:") -> (index of element=w137:i32)  [unwired: 1 in]
      n147 = Increment(x=w137) -> (x+1=w136:i32)
      n148 = Index Array(array=w149, index=w136) -> (element=w142:string)
      n149 = while {
        tunnel: w141 -> [w184]
        tunnel: w142 -> [w182]
        tunnel: [w181] -> _
        tunnel: [w181] -> w143
        tunnel: w144 -> [w180]
        i -> [w181]
        stop <- w177 stop-if-true
        n150 = Index Array(array=w184, index=w181) -> (element=w185:string)
        n151 = xnode "Match Regular Expression"("input string"=w185, "regular expression"=w182) -> ("whole match"=w183:string)  [unwired: 4 in, 4 out]
        n152 = Equal?(x=w183, y=w182) -> (x = y?=w179:bool)
        n153 = Equal?(x=w180, y=w181) -> (x = y?=w178:bool)
        n154 = Or(x=w179, y=w178) -> (x .or. y?=w177:bool)
      }
      n155 = case shown="True" w100 {
        tunnel: w101 -> [_ w172]
        frame False {
        }
        frame True {
          n156 = Read from Text File(file (use dialog)=w172) -> (text=w176:string)  [unwired: 3 in, 3 out]
          n157 = property on="Image Out" class="ImageControl"() -> ("ROI"=w173:T11)  [unwired: 2 in, 2 out]
          n158 = Unflatten From String(type=w173, binary string=w176) -> (value=w174:T11, error out=w175:errorcluster)  [unwired: 3 in, 1 out]
          n159 = property on="Image Out" class="ImageControl"(error in=w175, "ROI"=w174) -> ()  [unwired: 1 in, 2 out]
        }
      }
      n160 = Path To String(path=w145) -> (string=w146:string)
      n161 = invoke on="Image Out" class="ImageControl" method="Clear ROI"() -> ()  [unwired: 3 in, 3 out]
      n162 = Index Array(array=w141, index=w143) -> (element=w107:string)
      n163 = Empty String/Path?(string/path=w107) -> (empty?=w108:bool)
      n164 = Concatenate Strings(w146, "\\", w107) -> (w147:string)
      n165 = String To Path(string=w147) -> (path=w106:path)
      n166 = Select(t=w104, s=w108, f=w106) -> (s? t:f=w105:path)
      n167 = call "Vision Acquisition2"("Image Path"=w105) -> ("Image Out"=w140:T2)  [unwired: 25 in, 1 out]
      n168 = local write "Image File"(w105) -> ()
      n169 = local write "Image Out"(w140) -> ()
      n170 = local write "Image Out 2"(w140) -> ()
      n171 = local write "Image Name"(w107) -> ()
    }
    frame #2 {
      n172 = while {
        stop <- w584 stop-if-true
        w481 = "/"
        w534 = FALSE
        w532 = 0
        n173 = local read "Date Recorded"() -> (w484:string)
        n174 = local read "Ramp (s):"() -> (w451:dbl)
        n175 = local read "RPM:"() -> (w452:dbl)
        n176 = local read "Sat Vg Array-Used"() -> (w440:dbl[])
        n177 = local read "New: Dielectric"() -> (w425:dbl)
        n178 = local read "New: Length"() -> (w441:dbl)
        n179 = local read "New: Width"() -> (w443:dbl)
        n180 = local read "Sat Id-Used"() -> (w439:dbl[])
        n181 = local read "Lin-Vg Array-Used"() -> (w434:dbl[])
        n182 = Divide(x=w452, y=w451) -> (x/y=w450:dbl)
        n183 = local read "Sat Id-Log-Used"() -> (w438:dbl[])
        n184 = local read "New: Dielectric"() -> (w431:dbl)
        n185 = Match Pattern(string=w484, regular expression=w481) -> (before substring=w475:string, after substring=w482:string)  [unwired: 1 in, 2 out]
        n186 = local read "Vg Array-Log-Used"() -> (w437:dbl[])
        n187 = local read "New: Length"() -> (w433:dbl)
        n188 = local write "Accel (RPM/s):"(w450) -> ()
        n189 = local read "New: Width"() -> (w430:dbl)
        n190 = local read "Lin Id-Used"() -> (w435:dbl[])
        n191 = local read "New: Dielectric"() -> (w427:dbl)
        n192 = local read "Lin Vd"() -> (w429:dbl)
        n193 = String Length(string=w475) -> (length=w478:i32)
        n194 = Match Pattern(string=w482, regular expression=w481) -> (before substring=w469:string, after substring=w480:string)  [unwired: 1 in, 2 out]
        n195 = Equal?(x=w478, y=2) -> (x = y?=w476:bool)
        n196 = call "Mobility-Vt-Used Pts_Saturation.vi"("Width"=w443, "Length"=w441, "Dielectric (d)"=w425, "Sat Id Used"=w439, "Vg Used"=w440) -> ("Vt"=w426:dbl, "Mobility"=w442:dbl)  [unwired: 4 in, 1 out]
        n197 = String Length(string=w469) -> (length=w471:i32)
        n198 = call "Mobility-Vt-Used Pts_Linear.vi"("Width"=w430, "Length"=w433, "Vd"=w429, "Dielectric (d)"=w431, "Sat Id Used"=w435, "Vg Used"=w434) -> ("Vt"=w436:dbl, "Mobility"=w432:dbl)  [unwired: 3 in, 1 out]
        n199 = call "STS-Used.vi"("Id Used"=w438, "Vg-Used"=w437) -> ("STS"=w428:dbl)  [unwired: 9 in]
        n200 = case shown="False" w476 {
          tunnel: w475 -> [w610 w612]
          tunnel: [w609 w612] -> w474
          frame False {
            n201 = Concatenate Strings("0", w610) -> (w609:string)
          }
          frame True {
          }
        }
        n202 = local write "New: Mobility-Sat"(w442) -> ()
        n203 = Equal?(x=w471, y=2) -> (x = y?=w473:bool)
        n204 = local write "New: VT-Sat"(w426) -> ()
        n205 = local write "New: Mobility-Lin"(w432) -> ()
        n206 = local write "New: VT-Lin"(w436) -> ()
        n207 = case shown="False" w473 {
          tunnel: w469 -> [w606 w608]
          tunnel: [w605 w608] -> w470
          frame False {
            n208 = Concatenate Strings("0", w606) -> (w605:string)
          }
          frame True {
          }
        }
        n209 = call "Trap Density_VT.vi"("VT"=w426, "Dielectric"=w425) -> ("Trap Density-VT"=w424:dbl)
        n210 = local write "New: STS"(w428) -> ()
        n211 = local write "New: Trap Density-VT"(w424) -> ()
        n212 = local read "Index"() -> (w454:string)
        n213 = local read "Index"() -> (w468:string)
        n214 = local read "Manual-Temp"() -> (w421:bool)
        n215 = local read "Wait Time (s):"() -> (w514:dbl)
        n216 = local read "Rec: Temp"() -> (w422:dbl)
        n217 = String Subset(string=w454, length (rest)=1) -> (substring=w509:string)  [unwired: 1 in]
        n218 = local write "Row"(w509) -> ()
        n219 = local read "Treatment Concentration (mM):"() -> (w462:dbl)
        n220 = case shown="False" w421 {
          tunnel: w422 -> [w594 _]
          tunnel: [w591 w598] -> w420
          frame False {
            n221 = local read "Rec: Temp"() -> (w592:dbl)
            n222 = property on="New: Temp" class="DigNum (strict)"("DisabledEnum"=1) -> ()  [unwired: 2 in, 2 out]
            n223 = Equal To 0?(x=w592) -> (x = 0?=w593:bool)
            n224 = local write "New: Temp"(w594) -> ()
            n225 = case shown="True" w593 {
              tunnel: [w595 w596] -> w591
              tunnel: w592 -> [w595 _]
              frame False {
              }
              frame True {
                n226 = local read "Room Temp"() -> (w596:dbl)
              }
            }
            n227 = local write "New: Temp"(w591) -> ()
          }
          frame True {
            n228 = property on="New: Temp" class="DigNum (strict)"("DisabledEnum"=0) -> ()  [unwired: 2 in, 2 out]
            n229 = local read "New: Temp"() -> (w598:dbl)
          }
        }
        n230 = call "Trap Density_STS.vi"("Temp (T) [K]"=w420, "S.T.S. (S)"=w428, "Dielectric"=w427) -> ("Trap Density (N)"=w423:dbl)  [unwired: 8 in]
        n231 = local write "New: Trap Density-STS"(w423) -> ()
        n232 = local read "Rec: Concentration"() -> (w449:dbl)
        n233 = local read "Relative Humidity (%):"() -> (w459:dbl)
        n234 = String Subset(string=w454, offset (0)=1, length (rest)=2) -> (substring=w510:string)
        n235 = Number To Decimal String(number=w514) -> (decimal integer string=w515:string)  [unwired: 1 in]
        n236 = local read "Solution Temp (C):"() -> (w503:dbl)
        n237 = local read "Surface Treatment:"() -> (w461:string)
        n238 = local read "Room Temp (F):"() -> (w507:dbl)
        n239 = local read "Rec: Material"() -> (w457:string)
        n240 = local write "Column"(w510) -> ()
        n241 = local read "New: Length"() -> (w467:dbl)
        n242 = local read "New: Width"() -> (w466:dbl)
        n243 = local read "New: Mobility-Sat"() -> (w496:dbl)
        n244 = local read "Accel (RPM/s):"() -> (w494:dbl)
        n245 = local read "Sample #:"() -> (w486:dbl)
        n246 = local read "# Drops*:"() -> (w504:dbl)
        n247 = local read "Ramp (s):"() -> (w512:dbl)
        n248 = local read "New: STS"() -> (w488:dbl)
        n249 = local read "Rec: Solvent"() -> (w463:string)
        n250 = local read "New: VT-Sat"() -> (w490:dbl)
        n251 = local read "Rec: On/Off"() -> (w492:dbl)
        n252 = local read "Rec: Method"() -> (w487:string)
        n253 = local read "Time (s):"() -> (w499:dbl)
        n254 = local read "Date Recorded"() -> (w483:string)
        n255 = local read "RPM:"() -> (w500:dbl)
        n256 = local read "Fabricator:"() -> (w508:string)
        n257 = Number To Decimal String(number=w449) -> (decimal integer string=w448:string)  [unwired: 1 in]
        n258 = Number To Decimal String(number=w504) -> (decimal integer string=w505:string)  [unwired: 1 in]
        n259 = Number To Decimal String(number=w486) -> (decimal integer string=w479:string)  [unwired: 1 in]
        n260 = call "DeviceID"("Sample"=w479, "Year"=w480, "Month"=w474, "Day"=w470, "Index"=w468) -> ("Result"=w485:string)  [unwired: 9 in, 1 out]
        n261 = Number To Decimal String(number=w467) -> (decimal integer string=w465:string)  [unwired: 1 in]
        n262 = Number To Decimal String(number=w466) -> (decimal integer string=w464:string)  [unwired: 1 in]
        n263 = Number To Decimal String(number=w503) -> (decimal integer string=w502:string)  [unwired: 1 in]
        n264 = Number To Decimal String(number=w459) -> (decimal integer string=w458:string)  [unwired: 1 in]
        n265 = Number To Decimal String(number=w507) -> (decimal integer string=w506:string)  [unwired: 1 in]
        n266 = property on="Image Out" class="ImageControl"() -> ("ZoomSingle"=w552:cluster{"X":sgl, "Y":sgl})  [unwired: 2 in, 2 out]
        n267 = Number To Decimal String(number=w462) -> (decimal integer string=w460:string)  [unwired: 1 in]
        n268 = property on="Image Out" class="ImageControl"() -> ("Bounds"=w553:T12)  [unwired: 2 in, 2 out]
        n269 = Number To Decimal String(number=w500) -> (decimal integer string=w501:string)  [unwired: 1 in]
        n270 = Number To Fractional String(number=w494) -> (F-format string=w495:string)  [unwired: 3 in]
        n271 = Number To Decimal String(number=w499) -> (decimal integer string=w498:string)  [unwired: 1 in]
        n272 = Number To Fractional String(number=w496) -> (F-format string=w497:string)  [unwired: 3 in]
        n273 = Number To Fractional String(number=w492) -> (F-format string=w493:string)  [unwired: 3 in]
        n274 = Number To Fractional String(number=w490) -> (F-format string=w491:string)  [unwired: 3 in]
        n275 = Number To Fractional String(number=w488) -> (F-format string=w489:string)  [unwired: 3 in]
        n276 = Number To Decimal String(number=w512) -> (decimal integer string=w513:string)  [unwired: 1 in]
        n277 = call <vilib>:"Intialize Keyboard.vi"() -> ("device ID"=w564:refnum<k1>)  [unwired: 10 in, 1 out]
        n278 = property on="Image Out" class="ImageControl"() -> ("Image Center Position"=w559:cluster{"X":u32, "Y":u32})  [unwired: 2 in, 2 out]
        n279 = call-poly <vilib>:"Acquire Input Data.vi"("device ID"=w564) -> ("keys pressed"=w563:T13)  [unwired: 16 in, 2 out]
        n280 = Unbundle(w553) -> ("Width"=w550:u32, "Height"=w549:u32)
        n281 = Unbundle(w552) -> ("X"=w527:sgl, "Y"=w551:sgl)
        n282 = Index Array(array=w563) -> (element=w567:T14)  [unwired: 1 in]
        n283 = event shown="[1] \"Undo Button\": Mouse Down" {
          selector: _ -> [_ _ _ _ _ _ _]
          dyn-events: _ -> [_ _ _ _ _ _ _]
          timeout: 10 -> [_ _ _ _ _ _ _]
          event "Remove Button": Mouse Down {
            w619 = 0
            n284 = event-data() -> ()  [unwired: 1 in, 7 out]
            n285 = property on="Image Out" class="ImageControl"() -> ("ROI"=w617:T11)  [unwired: 2 in, 2 out]
            n286 = Unbundle(w617) -> ("Global Rectangle"=w620:i32[], "Contours"=w622:T15)
            n287 = Reverse 1D Array(array=w620) -> (reversed array=w621:i32[])
            n288 = Reverse 1D Array(array=w622) -> (reversed array=w623:T15)
            n289 = Delete From Array(array=w621, index=w619) -> (array with subset deleted=w624:i32[])  [unwired: 1 in, 1 out]
            n290 = Delete From Array(array=w623, index=w619) -> (array with subset deleted=w625:T15)  [unwired: 1 in, 1 out]
            n291 = Reverse 1D Array(array=w624) -> (reversed array=w626:i32[])
            n292 = Reverse 1D Array(array=w625) -> (reversed array=w627:T15)
            n293 = Bundle(w626, w627) -> (w618:T16)  [unwired: 1 in]
            n294 = local write "ROI Descriptor out"(w617) -> ()
            n295 = local write "ROI Descriptor"(w618) -> ()
            n296 = property on="Image Out" class="ImageControl"("ROI"=w618) -> ()  [unwired: 2 in, 2 out]
          }
          event "Undo Button": Mouse Down {
            n297 = event-data() -> ()  [unwired: 1 in, 7 out]
            n298 = invoke on="Image Out" class="ImageControl" method="Clear ROI"() -> ()  [unwired: 3 in, 3 out]
          }
          event "Image Folder": Value Change {
            n299 = event-data() -> ()  [unwired: 1 in, 5 out]
            n300 = local read "Image File"() -> (w629:path)
            n301 = call "Vision Acquisition"("Image Path"=w629) -> ("Image Out"=w628:T2)  [unwired: 25 in, 1 out]
            n302 = local write "Image Out 2"(w628) -> ()
            n303 = local write "Image Out"(w628) -> ()
            n304 = invoke on="Image Out" class="ImageControl" method="Clear ROI"() -> ()  [unwired: 3 in, 3 out]
          }
          event "Zoom": Value Change {
            n305 = event-data() -> ()  [unwired: 1 in, 5 out]
            n306 = local read "Zoom"() -> (w630:i16)
            n307 = Bundle("Zoom"=w630, "Zoom"=w630) -> (w631:cluster{"Zoom":i16, "Zoom":i16})  [unwired: 1 in]
            n308 = property on="Image Out" class="ImageControl"("ZoomInteger"=w631) -> ()  [unwired: 2 in, 2 out]
          }
          event Timeout {
            n309 = event-data() -> ()  [unwired: 1 in, 2 out]
          }
          event "Image Out": Mouse Enter {
            (unwired) 6
            n310 = event-data() -> ()  [unwired: 1 in, 3 out]
            n311 = call "Simulate_Keyboard.vi"("Action"=0, "Virtual Key"=162) -> ()  [unwired: 7 in, 1 out]
          }
          event "Image Out": Mouse Leave {
            n312 = event-data() -> ()  [unwired: 1 in, 3 out]
            n313 = flat-sequence {
              frame #0 {
                n314 = Wait (ms)(milliseconds to wait=10) -> ()  [unwired: 1 out]
              }
              frame #1 {
                (unwired) 6
                n315 = call "Simulate_Keyboard.vi"("Action"=2, "Virtual Key"=162) -> ()  [unwired: 7 in, 1 out]
              }
            }
          }
        }
        n316 = Divide(x=w550, y=w527) -> (x/y=w540:sgl)
        n317 = Multiply(x=w540, y=0.5) -> (x*y=w546:dbl)
        n318 = Divide(x=w549, y=w551) -> (x/y=w539:sgl)
        n319 = Multiply(x=w539, y=0.5) -> (x*y=w545:dbl)
        n320 = Unbundle(w559) -> ("X"=w541:u32, "Y"=w542:u32)
        n321 = Subtract(x=w542, y=w545) -> (x-y=w543:dbl)
        n322 = Subtract(x=w541, y=w546) -> (x-y=w544:dbl)
        n323 = Add(x=w544, y=w540) -> (x+y=w558:dbl)
        n324 = Add(x=w543, y=w539) -> (x+y=w557:dbl)
        n325 = Build Array(w485, w508, w487, w483, w479, w509, w510, w465, w464, w457, w461, w460, w463, w448, w502, w505, w515, w506, w458, w513, w501, w495, w498, w497, w493, w491, w489) -> (w511:string[])
        n326 = local write "Current \nRecord"(w511) -> ()
        n327 = Reciprocal(x=w527) -> (1/x=w526:sgl)
        n328 = event shown="[12] \"Save Changes? 2\": Mouse Down" {
          selector: _ -> [_ _ _ _ _ _ _ _ _ _ _ _ _ _ _ _]
          dyn-events: _ -> [_ _ _ _ _ _ _ _ _ _ _ _ _ _ _ _]
          timeout: 10 -> [_ _ _ _ _ _ _ _ _ _ _ _ _ _ _ _]
          tunnel: [_ _ _ _ _ _ _ _ _ _ _ _ _ TRUE _ TRUE] -> w584
          event Timeout {
            n329 = event-data() -> ()  [unwired: 1 in, 2 out]
          }
          event "Down Button": Mouse Down {
            w972 = 0
            n330 = event-data() -> ()  [unwired: 1 in, 7 out]
            n331 = local read "Transfer File"() -> (w977:path)
            n332 = Strip Path(path=w977) -> (stripped path=w968:path, name=w986:string)
            n333 = local write "Transfer Folder"(w968) -> ()
            n334 = List Folder(path=w968) -> (filenames=w982:string[], error out=w922:errorcluster)  [unwired: 3 in, 2 out]
            n335 = local read "Folder Index"() -> (w924:dbl)
            n336 = Array Size(array=w982) -> (size(s)=w978:i32)
            n337 = Search 1D Array(1D array=w982, element=w986) -> (index of element=w979:i32)  [unwired: 1 in]
            n338 = property on="Image Out" class="ImageControl"() -> (error out=w925:errorcluster, "Image Center Position"=w929:cluster{"X":u32, "Y":u32})  [unwired: 2 in, 1 out]
            n339 = Decrement(x=w978) -> (x-1=w980:i32)
            n340 = Equal?(x=w979, y=w980) -> (x = y?=w981:bool)
            n341 = invoke on="Image Out" class="ImageControl" method="Clear ROI"() -> ()  [unwired: 3 in, 3 out]
            n342 = case shown="False" w981 {
              tunnel: w924 -> [w1139 _]
              tunnel: [w1138 0] -> w923
              tunnel: w922 -> [w1137 w1140]
              tunnel: [w1137 w1140] -> w921
              frame False {
                n343 = Increment(x=w1139) -> (x+1=w1138:dbl)
              }
              frame True {
              }
            }
            n344 = Unbundle(w929) -> ("X"=w927:u32)  [unwired: 1 out]
            n345 = local write "Folder Index"(w923) -> ()
            n346 = Bundle("X"=w927, 0) -> (w928:cluster{"X":u32, i32})  [unwired: 1 in]
            n347 = property on="Image Out" class="ImageControl"(error in=w925, "Image Center Position"=w928) -> ()  [unwired: 1 in, 2 out]
            n348 = Path To String(path=w968) -> (string=w987:string)
            n349 = Index Array(array=w982, index=w923) -> (element=w983:string)
            n350 = local write "Data Name:"(w983) -> ()
            n351 = Concatenate Strings(w987, "\\", w983) -> (w985:string)
            n352 = String To Path(string=w985) -> (path=w896:path)
            n353 = call "Recorded Values.vi"("Path"=w896) -> ("Recorded Char"=w989:T5, "Recorded Prop"=w990:T6, "Fabrication Prop"=w988:T7)  [unwired: 8 in]
            n354 = Unbundle By Name(w989) -> ("Mobility-Sat"=w1002:dbl, "Moblitity-Lin"=w1003:dbl, "On/Off"=w1004:dbl, "Off Current"=w1005:dbl, "Vt-Sat"=w891:dbl, "STS"=w1006:dbl, "Trap Density-VT"=w1007:dbl, "Trap Density-STS"=w1008:dbl)
            n355 = Unbundle By Name(w988) -> ("Date Created"=w1009:string, "Material"=w991:string, "Solvent"=w992:string, "Concentration"=w993:dbl, "Method"=w994:string, "Dielectric (nm)"=w995:dbl, "Treatment"=w996:string, "Comments"=w997:string)
            n356 = Unbundle By Name(w990) -> ("Date Recorded"=w998:string, "Index"=w999:string, "Length"=w1000:dbl, "Width"=w1001:dbl, "Sample Temp"=w893:dbl)
            n357 = local write "Date Created"(w1009) -> ()
            n358 = local write "Rec: Off I-Sat"(w1005) -> ()
            n359 = local write "Rec: Comments"(w997) -> ()
            n360 = local write "Rec: Material"(w991) -> ()
            n361 = local write "Rec: VT-Sat"(w891) -> ()
            n362 = local write "Rec: Concentration"(w993) -> ()
            n363 = local write "Rec: Method"(w994) -> ()
            n364 = local write "Rec: Dielectric (d)"(w995) -> ()
            n365 = local write "Surface Treatment:"(w996) -> ()
            n366 = local write "Index"(w999) -> ()
            n367 = local write "Rec: Mobility-Sat"(w1002) -> ()
            n368 = local write "Rec: Mobility-Lin"(w1003) -> ()
            n369 = local write "Rec: On/Off"(w1004) -> ()
            n370 = local write "Rec: STS"(w1006) -> ()
            n371 = local write "Rec: Trap Density-VT"(w1007) -> ()
            n372 = local write "Rec: Trap Density-STS"(w1008) -> ()
            n373 = local write "Rec: Solvent"(w992) -> ()
            n374 = local write "Date Recorded"(w998) -> ()
            n375 = local write "Rec: Length"(w1000) -> ()
            n376 = local write "Rec: Width"(w1001) -> ()
            n377 = local write "Rec: Temp"(w893) -> ()
            n378 = Equal To 0?(x=w893) -> (x = 0?=w894:bool)
            n379 = case shown="True" w894 {
              tunnel: [w1010 w1011] -> w892
              tunnel: w893 -> [w1010 _]
              frame False {
              }
              frame True {
                n380 = local read "Room Temp"() -> (w1011:dbl)
              }
            }
            n381 = local read "NumPoints Log"() -> (w917:dbl)
            n382 = local write "Transfer File"(w896) -> ()
            n383 = local read "Num Pts"() -> (w920:dbl)
            n384 = call-poly <vilib>:"Read From Spreadsheet File.vi"("file path (dialog if empty)"=w896) -> ("all rows"=w974:string[][])  [unwired: 6 in, 4 out]
            n385 = call "Mobility-Vt Calculator-File.vi"("NumPts"=w920, "Path"=w896) -> ("Graph Cluster"=w889:T8, "Output"=w919:T9, "Index-Sat"=w918:dbl, "Index-Lin"=w904:dbl)  [unwired: 5 in, 1 out]
            n386 = local read "New: Dielectric"() -> (w901:dbl)
            n387 = call "STS Calculator-File.vi"("NumPts"=w917, "Path"=w896) -> ("STS Index-Sat"=w916:dbl, "XY Graph-Sat"=w915:cluster{dbl[], dbl[]}[], "Ouput"=w914:cluster{"STS-Sat":dbl, "STS-Lin":dbl})  [unwired: 5 in, 2 out]
            n388 = local write "Sat-Trans Slider"(w918) -> ()
            n389 = Unbundle By Name(w919) -> ("Mobility-Sat"=w913:dbl, "Vt-Sat"=w900:dbl, "Mobility-Lin"=w912:dbl, "Vt-Lin"=w911:dbl, "Off I-Sat"=w897:dbl, "On/Off I-Sat"=w890:dbl)
            n390 = Unbundle By Name(w914) -> ("STS-Sat"=w895:dbl)  [unwired: 1 out]
            n391 = local write "Index 2"(w916) -> ()
            n392 = local write "MobVi Index"(w918) -> ()
            n393 = local write "Log-Sat"(w915) -> ()
            n394 = Array Size(array=w974) -> (size(s)=w973:i32[])
            n395 = Unbundle By Name(w889) -> ("Sqrt Sat"=w888:cluster{dbl[], dbl[]}[], "Sqrt Lin"=w887:cluster{dbl[], dbl[]}[])  [unwired: 4 out]
            n396 = local write "Sqrt-Sat"(w888) -> ()
            n397 = call "Trap Density_VT.vi"("VT"=w900, "Dielectric"=w901) -> ("Trap Density-VT"=w899:dbl)
            n398 = call "Trap Density_STS.vi"("Temp (T) [K]"=w892, "S.T.S. (S)"=w895, "Dielectric"=w901) -> ("Trap Density (N)"=w898:dbl)  [unwired: 8 in]
            n399 = local write "New: STS"(w895) -> ()
            n400 = local write "Calc: STS"(w895) -> ()
            n401 = local write "Calc: Mobility-Sat"(w913) -> ()
            n402 = local write "Calc: Off I-Sat"(w911) -> ()
            n403 = local write "Calc: Mobility-Lin"(w912) -> ()
            n404 = Index Array(array=w973, index=w972) -> (element=w954:i32)
            n405 = Decimate 1D Array(w915) -> (w948:cluster{dbl[], dbl[]}[])  [unwired: 1 out]
            n406 = Decimate 1D Array(w888) -> (w958:cluster{dbl[], dbl[]}[])  [unwired: 1 out]
            n407 = local write "Calc: Off I-Sat"(w897) -> ()
            n408 = local write "Calc: On/Off"(w890) -> ()
            n409 = Decimate 1D Array(w887) -> (w910:cluster{dbl[], dbl[]}[])  [unwired: 1 out]
            n410 = local write "Calc: VT-Sat"(w900) -> ()
            n411 = Array Subset(array=w974, index (row)=w972, index (col)=w972, length (col)=3) -> (w975:string[][])  [unwired: 1 in]
            n412 = local write "Calc: Trap Density-VT"(w899) -> ()
            n413 = local write "Calc: Trap Density-STS"(w898) -> ()
            n414 = local write "New: Trap Density-STS"(w898) -> ()
            n415 = local write "New: Trap Density-VT"(w899) -> ()
            n416 = Array To Cluster(array=w948) -> (cluster=w946:T10)
            n417 = Array To Cluster(array=w958) -> (cluster=w960:T10)
            n418 = local write "Sqrt-Lin"(w887) -> ()
            n419 = local write "New: VT-Lin"(w911) -> ()
            n420 = local write "New: VT-Sat"(w900) -> ()
            n421 = local write "New: Mobility-Sat"(w913) -> ()
            n422 = local write "New: Mobility-Lin"(w912) -> ()
            n423 = Reshape Array(w975, w954) -> (w961:string[])
            n424 = Array To Cluster(array=w910) -> (cluster=w909:T10)
            n425 = Subtract(x=w954, y=20) -> (x-y=w953:i32)
            n426 = property on="Sat-Trans Slider" class="Slide (strict)"("Scale.Maximum"=w953) -> ()  [unwired: 2 in, 2 out]
            n427 = Unbundle(w946) -> ("[0]"=w947:cluster{dbl[], dbl[]})  [unwired: 8 out]
            n428 = Unbundle(w960) -> ("[0]"=w959:cluster{dbl[], dbl[]})  [unwired: 8 out]
            n429 = Unbundle(w909) -> ("[0]"=w906:cluster{dbl[], dbl[]})  [unwired: 8 out]
            n430 = Search 1D Array(1D array=w961, element="Index:") -> (index of element=w969:i32)  [unwired: 1 in]
            n431 = local read "Num Pts"() -> (w905:dbl)
            n432 = Unbundle(w906) -> (w908:dbl[], w907:dbl[])
            n433 = Increment(x=w969) -> (x+1=w970:i32)
            n434 = Unbundle(w947) -> (w945:dbl[], w944:dbl[])
            n435 = Unbundle(w959) -> (w950:dbl[], w949:dbl[])
            n436 = Array Subset(array=w908, index=w904, length=w905) -> (w903:dbl[])
            n437 = Array Subset(array=w907, index=w904, length=w905) -> (w902:dbl[])
            n438 = Array Subset(array=w945, index=w916, length=w917) -> (w952:dbl[])
            n439 = Array Subset(array=w944, index=w916, length=w917) -> (w951:dbl[])
            n440 = Array Subset(array=w950, index=w918, length=w920) -> (w957:dbl[])
            n441 = Array Subset(array=w949, index=w918, length=w920) -> (w956:dbl[])
            n442 = Index Array(array=w961, index=w970) -> (element=w933:string)
            n443 = local write "Lin-Vg Array-Used"(w903) -> ()
            n444 = local write "Sat Vg Array-Used"(w957) -> ()
            n445 = local write "Vg Array-Log-Used"(w951) -> ()
            n446 = local write "Lin Id-Used"(w902) -> ()
            n447 = local read "Image Folder"() -> (w931:path)
            n448 = local write "Sat Id-Used"(w956) -> ()
            n449 = local write "Sat Id-Log-Used"(w952) -> ()
            n450 = List Folder(path=w931, error in=w921) -> (filenames=w967:string[], error out=w934:errorcluster)  [unwired: 2 in, 2 out]
            n451 = while {
              tunnel: w967 -> [w1024]
              tunnel: w933 -> [w1022]
              tunnel: [w1021] -> _
              tunnel: [w1021] -> w966
              tunnel: w954 -> [w1020]
              i -> [w1021]
              stop <- w1017 stop-if-true
              n452 = Index Array(array=w1024, index=w1021) -> (element=w1025:string)
              n453 = xnode "Match Regular Expression"("input string"=w1025, "regular expression"=w1022) -> ("whole match"=w1023:string)  [unwired: 4 in, 4 out]
              n454 = Equal?(x=w1023, y=w1022) -> (x = y?=w1019:bool)
              n455 = Equal?(x=w1020, y=w1021) -> (x = y?=w1018:bool)
              n456 = Or(x=w1019, y=w1018) -> (x .or. y?=w1017:bool)
            }
            n457 = Build Path(base path=w931, name or relative path="ROI") -> (appended path=w930:path)
            n458 = Path To String(path=w931) -> (string=w964:string)
            n459 = Index Array(array=w967, index=w966) -> (element=w942:string)
            n460 = invoke on="Image Out" class="ImageControl" method="Clear ROI"(error in=w934) -> (error out=w937:errorcluster)  [unwired: 2 in, 2 out]
            n461 = local write "Image Name"(w942) -> ()
            n462 = Build Path(base path=w930, name or relative path=w933) -> (appended path=w938:path)
            n463 = call <vilib>:"Check if File or Folder Exists.vi"("error in (no error)"=w937, "path"=w938) -> ("file or folder exists?"=w935:bool, "dup path"=w936:path)  [unwired: 7 in, 1 out]
            n464 = Concatenate Strings(w964, "\\", w942) -> (w963:string)
            n465 = case shown="False" w935 {
              tunnel: w936 -> [_ w1012]
              frame False {
              }
              frame True {
                n466 = Read from Text File(file (use dialog)=w1012) -> (text=w1016:string)  [unwired: 3 in, 3 out]
                n467 = property on="Image Out" class="ImageControl"() -> ("ROI"=w1013:T11)  [unwired: 2 in, 2 out]
                n468 = Unflatten From String(type=w1013, binary string=w1016) -> (value=w1014:T11, error out=w1015:errorcluster)  [unwired: 3 in, 1 out]
                n469 = property on="Image Out" class="ImageControl"(error in=w1015, "ROI"=w1014) -> ()  [unwired: 1 in, 2 out]
              }
            }
            n470 = String To Path(string=w963) -> (path=w941:path)
            n471 = Empty String/Path?(string/path=w942) -> (empty?=w943:bool)
            n472 = local read "No Image File"() -> (w939:path)
            n473 = Select(t=w939, s=w943, f=w941) -> (s? t:f=w940:path)
            n474 = local write "Image File"(w940) -> ()
            n475 = call "Vision Acquisition4"("Image Path"=w940) -> ("Image Out"=w965:T2)  [unwired: 25 in, 1 out]
            n476 = local write "Image Out"(w965) -> ()
            n477 = local write "Image Out 2"(w965) -> ()
          }
          event "Transfer File": Value Change {
            w1249 = 0
            n478 = event-data() -> ()  [unwired: 1 in, 5 out]
            n479 = local read "Transfer File"() -> (w1245:path)
            n480 = Strip Path(path=w1245) -> (stripped path=w1244:path, name=w1258:string)
            n481 = local write "Transfer Folder"(w1244) -> ()
            n482 = property on="Image Out" class="ImageControl"() -> (error out=w1200:errorcluster, "Image Center Position"=w1204:cluster{"X":u32, "Y":u32})  [unwired: 2 in, 1 out]
            n483 = List Folder(path=w1244) -> (filenames=w1254:string[], error out=w1210:errorcluster)  [unwired: 3 in, 2 out]
            n484 = Search 1D Array(1D array=w1254, element=w1258) -> (index of element=w1199:i32)  [unwired: 1 in]
            n485 = local write "Folder Index"(w1199) -> ()
            n486 = Unbundle(w1204) -> ("X"=w1202:u32)  [unwired: 1 out]
            n487 = Path To String(path=w1244) -> (string=w1259:string)
            n488 = Index Array(array=w1254, index=w1199) -> (element=w1255:string)
            n489 = Bundle("X"=w1202, 0) -> (w1203:cluster{"X":u32, i32})  [unwired: 1 in]
            n490 = local write "Data Name:"(w1255) -> ()
            n491 = property on="Image Out" class="ImageControl"(error in=w1200, "Image Center Position"=w1203) -> ()  [unwired: 1 in, 2 out]
            n492 = Concatenate Strings(w1259, "\\", w1255) -> (w1257:string)
            n493 = String To Path(string=w1257) -> (path=w1151:path)
            n494 = call "Recorded Values.vi"("Path"=w1151) -> ("Recorded Char"=w1197:T5, "Recorded Prop"=w1196:T6, "Fabrication Prop"=w1198:T7)  [unwired: 8 in]
            n495 = Unbundle By Name(w1197) -> ("Mobility-Sat"=w1184:dbl, "Moblitity-Lin"=w1183:dbl, "On/Off"=w1182:dbl, "Off Current"=w1181:dbl, "Vt-Sat"=w1147:dbl, "STS"=w1180:dbl, "Trap Density-VT"=w1179:dbl, "Trap Density-STS"=w1178:dbl)
            n496 = Unbundle By Name(w1198) -> ("Date Created"=w1177:string, "Material"=w1195:string, "Solvent"=w1194:string, "Concentration"=w1193:dbl, "Method"=w1192:string, "Dielectric (nm)"=w1191:dbl, "Treatment"=w1190:string, "Comments"=w1189:string)
            n497 = Unbundle By Name(w1196) -> ("Date Recorded"=w1188:string, "Index"=w1187:string, "Length"=w1186:dbl, "Width"=w1185:dbl, "Sample Temp"=w1149:dbl)
            n498 = local write "Date Created"(w1177) -> ()
            n499 = local write "Rec: Material"(w1195) -> ()
            n500 = local write "Rec: Off I-Sat"(w1181) -> ()
            n501 = local write "Rec: Comments"(w1189) -> ()
            n502 = local write "Rec: VT-Sat"(w1147) -> ()
            n503 = local write "Rec: Concentration"(w1193) -> ()
            n504 = local write "Rec: Method"(w1192) -> ()
            n505 = local write "Rec: Dielectric (d)"(w1191) -> ()
            n506 = local write "Surface Treatment:"(w1190) -> ()
            n507 = local write "Index"(w1187) -> ()
            n508 = local write "Rec: Mobility-Sat"(w1184) -> ()
            n509 = local write "Rec: Mobility-Lin"(w1183) -> ()
            n510 = local write "Rec: On/Off"(w1182) -> ()
            n511 = local write "Rec: STS"(w1180) -> ()
            n512 = local write "Rec: Trap Density-VT"(w1179) -> ()
            n513 = local write "Rec: Trap Density-STS"(w1178) -> ()
            n514 = local write "Rec: Solvent"(w1194) -> ()
            n515 = local write "Date Recorded"(w1188) -> ()
            n516 = local write "Rec: Length"(w1186) -> ()
            n517 = local write "Rec: Width"(w1185) -> ()
            n518 = local write "Rec: Temp"(w1149) -> ()
            n519 = Equal To 0?(x=w1149) -> (x = 0?=w1150:bool)
            n520 = case shown="False" w1150 {
              tunnel: [w1260 w1261] -> w1148
              tunnel: w1149 -> [w1260 _]
              frame False {
              }
              frame True {
                n521 = local read "Room Temp"() -> (w1261:dbl)
              }
            }
            n522 = local read "NumPoints Log"() -> (w1173:dbl)
            n523 = local write "Transfer File"(w1151) -> ()
            n524 = local read "Num Pts"() -> (w1174:dbl)
            n525 = call-poly <vilib>:"Read From Spreadsheet File.vi"("file path (dialog if empty)"=w1151) -> ("all rows"=w1251:string[][])  [unwired: 6 in, 4 out]
            n526 = local read "New: Dielectric"() -> (w1157:dbl)
            n527 = call "STS Calculator-File.vi"("NumPts"=w1173, "Path"=w1151) -> ("STS Index-Sat"=w1171:dbl, "XY Graph-Sat"=w1172:cluster{dbl[], dbl[]}[], "Ouput"=w1170:cluster{"STS-Sat":dbl, "STS-Lin":dbl})  [unwired: 5 in, 2 out]
            n528 = call "Mobility-Vt Calculator-File.vi"("NumPts"=w1174, "Path"=w1151) -> ("Graph Cluster"=w1144:T8, "Output"=w1175:T9, "Index-Sat"=w1176:dbl, "Index-Lin"=w1163:dbl)  [unwired: 5 in, 1 out]
            n529 = Unbundle By Name(w1175) -> ("Mobility-Sat"=w1159:dbl, "Vt-Sat"=w1153:dbl, "Mobility-Lin"=w1158:dbl, "Vt-Lin"=w1145:dbl, "Off I-Sat"=w1152:dbl, "On/Off I-Sat"=w1146:dbl)
            n530 = local write "Index 2"(w1171) -> ()
            n531 = Unbundle By Name(w1170) -> ("STS-Sat"=w1154:dbl)  [unwired: 1 out]
            n532 = local write "MobVi Index"(w1176) -> ()
            n533 = local write "Log-Sat"(w1172) -> ()
            n534 = local write "Sat-Trans Slider"(w1176) -> ()
            n535 = Array Size(array=w1251) -> (size(s)=w1250:i32[])
            n536 = call "Trap Density_VT.vi"("VT"=w1153, "Dielectric"=w1157) -> ("Trap Density-VT"=w1156:dbl)
            n537 = call "Trap Density_STS.vi"("Temp (T) [K]"=w1148, "S.T.S. (S)"=w1154, "Dielectric"=w1157) -> ("Trap Density (N)"=w1155:dbl)  [unwired: 8 in]
            n538 = local write "Calc: Mobility-Lin"(w1158) -> ()
            n539 = local write "Calc: Mobility-Sat"(w1159) -> ()
            n540 = local write "Calc: VT-Sat"(w1153) -> ()
            n541 = local write "Calc: Off I-Sat"(w1152) -> ()
            n542 = local write "Calc: VT-Lin"(w1145) -> ()
            n543 = local write "Calc: On/Off"(w1146) -> ()
            n544 = local write "Calc: STS"(w1154) -> ()
            n545 = Unbundle By Name(w1144) -> ("Sqrt Sat"=w1142:cluster{dbl[], dbl[]}[], "Sqrt Lin"=w1143:cluster{dbl[], dbl[]}[])  [unwired: 4 out]
            n546 = Decimate 1D Array(w1143) -> (w1169:cluster{dbl[], dbl[]}[])  [unwired: 1 out]
            n547 = local write "Calc: Trap Density-VT"(w1156) -> ()
            n548 = local write "Calc: Trap Density-STS"(w1155) -> ()
            n549 = local write "New: Trap Density-STS"(w1155) -> ()
            n550 = local write "New: Trap Density-VT"(w1156) -> ()
            n551 = local write "Sqrt-Lin"(w1143) -> ()
            n552 = local write "New: VT-Sat"(w1153) -> ()
            n553 = Decimate 1D Array(w1172) -> (w1225:cluster{dbl[], dbl[]}[])  [unwired: 1 out]
            n554 = Index Array(array=w1250, index=w1249) -> (element=w1231:i32)
            n555 = Decimate 1D Array(w1142) -> (w1234:cluster{dbl[], dbl[]}[])  [unwired: 1 out]
            n556 = local write "Sqrt-Sat"(w1142) -> ()
            n557 = local write "New: Mobility-Lin"(w1158) -> ()
            n558 = Array Subset(array=w1251, index (row)=w1249, index (col)=w1249, length (col)=3) -> (w1252:string[][])  [unwired: 1 in]
            n559 = local write "New: VT-Lin"(w1145) -> ()
            n560 = Array To Cluster(array=w1169) -> (cluster=w1168:T10)
            n561 = local write "New: STS"(w1154) -> ()
            n562 = local write "New: Mobility-Sat"(w1159) -> ()
            n563 = Array To Cluster(array=w1225) -> (cluster=w1223:T10)
            n564 = Array To Cluster(array=w1234) -> (cluster=w1236:T10)
            n565 = Reshape Array(w1252, w1231) -> (w1237:string[])
            n566 = Subtract(x=w1231, y=20) -> (x-y=w1229:i32)
            n567 = Unbundle(w1168) -> ("[0]"=w1167:cluster{dbl[], dbl[]})  [unwired: 8 out]
            n568 = local read "Num Pts"() -> (w1164:dbl)
            n569 = property on="Sat-Trans Slider" class="Slide (strict)"("Scale.Maximum"=w1229) -> ()  [unwired: 2 in, 2 out]
            n570 = Unbundle(w1167) -> (w1166:dbl[], w1165:dbl[])
            n571 = Unbundle(w1223) -> ("[0]"=w1224:cluster{dbl[], dbl[]})  [unwired: 8 out]
            n572 = Unbundle(w1236) -> ("[0]"=w1235:cluster{dbl[], dbl[]})  [unwired: 8 out]
            n573 = Search 1D Array(1D array=w1237, element="Index:") -> (index of element=w1246:i32)  [unwired: 1 in]
            n574 = local read "Num Pts"() -> (w1160:dbl)
            n575 = Array Subset(array=w1166, index=w1163, length=w1164) -> (w1162:dbl[])
            n576 = Array Subset(array=w1165, index=w1163, length=w1164) -> (w1161:dbl[])
            n577 = Increment(x=w1246) -> (x+1=w1247:i32)
            n578 = Unbundle(w1224) -> (w1221:dbl[], w1220:dbl[])
            n579 = Unbundle(w1235) -> (w1222:dbl[], w1226:dbl[])
            n580 = local read "Image Folder"() -> (w1206:path)
            n581 = local write "Lin-Vg Array-Used"(w1162) -> ()
            n582 = Array Subset(array=w1221, index=w1171, length=w1173) -> (w1228:dbl[])
            n583 = Array Subset(array=w1220, index=w1171, length=w1173) -> (w1227:dbl[])
            n584 = Array Subset(array=w1222, index=w1176, length=w1160) -> (w1233:dbl[])
            n585 = Array Subset(array=w1226, index=w1176, length=w1160) -> (w1232:dbl[])
            n586 = Index Array(array=w1237, index=w1247) -> (element=w1208:string)
            n587 = local write "Lin Id-Used"(w1161) -> ()
            n588 = local write "Sat Vg Array-Used"(w1233) -> ()
            n589 = local write "Vg Array-Log-Used"(w1227) -> ()
            n590 = local write "Sat Id-Log-Used"(w1228) -> ()
            n591 = local write "Sat Id-Used"(w1232) -> ()
            n592 = local write "Index"(w1208) -> ()
            n593 = List Folder(path=w1206, error in=w1210) -> (filenames=w1242:string[], error out=w1209:errorcluster)  [unwired: 2 in, 2 out]
            n594 = Build Path(base path=w1206, name or relative path="ROI") -> (appended path=w1205:path)
            n595 = invoke on="Image Out" class="ImageControl" method="Clear ROI"(error in=w1209) -> (error out=w1213:errorcluster)  [unwired: 2 in, 2 out]
            n596 = Build Path(base path=w1205, name or relative path=w1208) -> (appended path=w1214:path)
            n597 = while {
              tunnel: w1242 -> [w1274]
              tunnel: w1208 -> [w1272]
              tunnel: [w1271] -> _
              tunnel: [w1271] -> w1241
              tunnel: w1231 -> [w1270]
              i -> [w1271]
              stop <- w1267 stop-if-true
              n598 = Index Array(array=w1274, index=w1271) -> (element=w1275:string)
              n599 = xnode "Match Regular Expression"("input string"=w1275, "regular expression"=w1272) -> ("whole match"=w1273:string)  [unwired: 4 in, 4 out]
              n600 = Equal?(x=w1273, y=w1272) -> (x = y?=w1269:bool)
              n601 = Equal?(x=w1270, y=w1271) -> (x = y?=w1268:bool)
              n602 = Or(x=w1269, y=w1268) -> (x .or. y?=w1267:bool)
            }
            n603 = call <vilib>:"Check if File or Folder Exists.vi"("error in (no error)"=w1213, "path"=w1214) -> ("file or folder exists?"=w1211:bool, "dup path"=w1212:path)  [unwired: 7 in, 1 out]
            n604 = case shown="True" w1211 {
              tunnel: w1212 -> [_ w1262]
              frame False {
              }
              frame True {
                n605 = Read from Text File(file (use dialog)=w1262) -> (text=w1266:string)  [unwired: 3 in, 3 out]
                n606 = property on="Image Out" class="ImageControl"() -> ("ROI"=w1263:T11)  [unwired: 2 in, 2 out]
                n607 = Unflatten From String(type=w1263, binary string=w1266) -> (value=w1264:T11, error out=w1265:errorcluster)  [unwired: 3 in, 1 out]
                n608 = property on="Image Out" class="ImageControl"(error in=w1265, "ROI"=w1264) -> ()  [unwired: 1 in, 2 out]
              }
            }
            n609 = invoke on="Image Out" class="ImageControl" method="Clear ROI"() -> ()  [unwired: 3 in, 3 out]
            n610 = Path To String(path=w1206) -> (string=w1240:string)
            n611 = Index Array(array=w1242, index=w1241) -> (element=w1218:string)
            n612 = Concatenate Strings(w1240, "\\", w1218) -> (w1239:string)
            n613 = local write "Image Name"(w1218) -> ()
            n614 = String To Path(string=w1239) -> (path=w1217:path)
            n615 = Empty String/Path?(string/path=w1218) -> (empty?=w1219:bool)
            n616 = local read "No Image File"() -> (w1215:path)
            n617 = Select(t=w1215, s=w1219, f=w1217) -> (s? t:f=w1216:path)
            n618 = local write "Image File"(w1216) -> ()
            n619 = call "Vision Acquisition3"("Image Path"=w1216) -> ("Image Out"=w1243:T2)  [unwired: 25 in, 1 out]
            n620 = local write "Image Out"(w1243) -> ()
            n621 = local write "Image Out 2"(w1243) -> ()
          }
          event "Up Button": Mouse Down {
            w1495 = 0
            n622 = event-data() -> ()  [unwired: 1 in, 5 out]
            n623 = local read "Transfer File"() -> (w1491:path)
            n624 = Strip Path(path=w1491) -> (stripped path=w1490:path, name=w1506:string)
            n625 = local write "Transfer Folder"(w1490) -> ()
            n626 = List Folder(path=w1490) -> (filenames=w1500:string[], error out=w1457:errorcluster)  [unwired: 3 in, 2 out]
            n627 = Array Size(array=w1500) -> (size(s)=w1445:i32)
            n628 = Search 1D Array(1D array=w1500, element=w1506) -> (index of element=w1501:i32)  [unwired: 1 in]
            n629 = Equal To 0?(x=w1501) -> (x = 0?=w1502:bool)
            n630 = local read "Folder Index"() -> (w1444:dbl)
            n631 = property on="Image Out" class="ImageControl"() -> (error out=w1447:errorcluster, "Image Center Position"=w1451:cluster{"X":u32, "Y":u32})  [unwired: 2 in, 1 out]
            n632 = case shown="True" w1502 {
              tunnel: w1444 -> [w1636 _]
              tunnel: [w1635 w1637] -> w1443
              tunnel: w1445 -> [_ w1638]
              frame False {
                n633 = Decrement(x=w1636) -> (x-1=w1635:dbl)
              }
              frame True {
                n634 = Decrement(x=w1638) -> (x-1=w1637:i32)
              }
            }
            n635 = Unbundle(w1451) -> ("X"=w1449:u32)  [unwired: 1 out]
            n636 = local write "Folder Index"(w1443) -> ()
            n637 = Bundle("X"=w1449, 0) -> (w1450:cluster{"X":u32, i32})  [unwired: 1 in]
            n638 = Path To String(path=w1490) -> (string=w1507:string)
            n639 = Index Array(array=w1500, index=w1443) -> (element=w1503:string)
            n640 = local write "Data Name:"(w1503) -> ()
            n641 = property on="Image Out" class="ImageControl"(error in=w1447, "Image Center Position"=w1450) -> ()  [unwired: 1 in, 2 out]
            n642 = Concatenate Strings(w1507, "\\", w1503) -> (w1505:string)
            n643 = String To Path(string=w1505) -> (path=w1395:path)
            n644 = call "Recorded Values.vi"("Path"=w1395) -> ("Recorded Char"=w1441:T5, "Recorded Prop"=w1440:T6, "Fabrication Prop"=w1442:T7)  [unwired: 8 in]
            n645 = Unbundle By Name(w1441) -> ("Mobility-Sat"=w1428:dbl, "Moblitity-Lin"=w1427:dbl, "On/Off"=w1426:dbl, "Off Current"=w1425:dbl, "Vt-Sat"=w1391:dbl, "STS"=w1424:dbl, "Trap Density-VT"=w1423:dbl, "Trap Density-STS"=w1422:dbl)
            n646 = Unbundle By Name(w1442) -> ("Date Created"=w1421:string, "Material"=w1439:string, "Solvent"=w1438:string, "Concentration"=w1437:dbl, "Method"=w1436:string, "Dielectric (nm)"=w1435:dbl, "Treatment"=w1434:string, "Comments"=w1433:string)
            n647 = Unbundle By Name(w1440) -> ("Date Recorded"=w1432:string, "Index"=w1431:string, "Length"=w1430:dbl, "Width"=w1429:dbl, "Sample Temp"=w1392:dbl)
            n648 = local write "Date Created"(w1421) -> ()
            n649 = local write "Rec: Material"(w1439) -> ()
            n650 = local write "Rec: Off I-Sat"(w1425) -> ()
            n651 = local write "Rec: Comments"(w1433) -> ()
            n652 = local write "Rec: VT-Sat"(w1391) -> ()
            n653 = local write "Rec: Solvent"(w1438) -> ()
            n654 = local write "Rec: Concentration"(w1437) -> ()
            n655 = local write "Rec: Method"(w1436) -> ()
            n656 = local write "Rec: Dielectric (d)"(w1435) -> ()
            n657 = local write "Surface Treatment:"(w1434) -> ()
            n658 = local write "Index"(w1431) -> ()
            n659 = local write "Rec: Mobility-Sat"(w1428) -> ()
            n660 = local write "Rec: Mobility-Lin"(w1427) -> ()
            n661 = local write "Rec: On/Off"(w1426) -> ()
            n662 = local write "Rec: STS"(w1424) -> ()
            n663 = local write "Rec: Trap Density-VT"(w1423) -> ()
            n664 = local write "Rec: Trap Density-STS"(w1422) -> ()
            n665 = local write "Date Recorded"(w1432) -> ()
            n666 = local write "Rec: Length"(w1430) -> ()
            n667 = local write "Rec: Width"(w1429) -> ()
            n668 = local write "Rec: Temp"(w1392) -> ()
            n669 = Equal To 0?(x=w1392) -> (x = 0?=w1394:bool)
            n670 = case shown="False" w1394 {
              tunnel: [w1508 w1509] -> w1393
              tunnel: w1392 -> [w1508 _]
              frame False {
              }
              frame True {
                n671 = local read "Room Temp"() -> (w1509:dbl)
              }
            }
            n672 = local read "NumPoints Log"() -> (w1417:dbl)
            n673 = local write "Transfer File"(w1395) -> ()
            n674 = local read "Num Pts"() -> (w1420:dbl)
            n675 = local read "New: Dielectric"() -> (w1401:dbl)
            n676 = call "Mobility-Vt Calculator-File.vi"("NumPts"=w1420, "Path"=w1395) -> ("Graph Cluster"=w1389:T8, "Output"=w1419:T9, "Index-Sat"=w1418:dbl, "Index-Lin"=w1405:dbl)  [unwired: 5 in, 1 out]
            n677 = call "STS Calculator-File.vi"("NumPts"=w1417, "Path"=w1395) -> ("STS Index-Sat"=w1416:dbl, "XY Graph-Sat"=w1415:cluster{dbl[], dbl[]}[], "Ouput"=w1414:cluster{"STS-Sat":dbl, "STS-Lin":dbl})  [unwired: 5 in, 2 out]
            n678 = call-poly <vilib>:"Read From Spreadsheet File.vi"("file path (dialog if empty)"=w1395) -> ("all rows"=w1497:string[][])  [unwired: 6 in, 4 out]
            n679 = Unbundle By Name(w1419) -> ("Mobility-Sat"=w1404:dbl, "Vt-Sat"=w1397:dbl, "Mobility-Lin"=w1403:dbl, "Vt-Lin"=w1402:dbl, "Off I-Sat"=w1396:dbl, "On/Off I-Sat"=w1390:dbl)
            n680 = local write "Sat-Trans Slider"(w1418) -> ()
            n681 = Unbundle By Name(w1414) -> ("STS-Sat"=w1398:dbl)  [unwired: 1 out]
            n682 = local write "Index 2"(w1416) -> ()
            n683 = local write "MobVi Index"(w1418) -> ()
            n684 = local write "Log-Sat"(w1415) -> ()
            n685 = local write "Calc: Mobility-Sat"(w1404) -> ()
            n686 = local write "Calc: VT-Sat"(w1397) -> ()
            n687 = local write "Calc: Mobility-Lin"(w1403) -> ()
            n688 = local write "Calc: Off I-Sat"(w1396) -> ()
            n689 = local write "Calc: On/Off"(w1390) -> ()
            n690 = Array Size(array=w1497) -> (size(s)=w1496:i32[])
            n691 = local write "Calc: VT-Lin"(w1402) -> ()
            n692 = call "Trap Density_VT.vi"("VT"=w1397, "Dielectric"=w1401) -> ("Trap Density-VT"=w1400:dbl)
            n693 = call "Trap Density_STS.vi"("Temp (T) [K]"=w1393, "S.T.S. (S)"=w1398, "Dielectric"=w1401) -> ("Trap Density (N)"=w1399:dbl)  [unwired: 8 in]
            n694 = Unbundle By Name(w1389) -> ("Sqrt Sat"=w1387:cluster{dbl[], dbl[]}[], "Sqrt Lin"=w1388:cluster{dbl[], dbl[]}[])  [unwired: 4 out]
            n695 = local write "Sqrt-Sat"(w1387) -> ()
            n696 = local write "Calc: STS"(w1398) -> ()
            n697 = local write "New: STS"(w1398) -> ()
            n698 = Decimate 1D Array(w1388) -> (w1413:cluster{dbl[], dbl[]}[])  [unwired: 1 out]
            n699 = local write "Calc: Trap Density-VT"(w1400) -> ()
            n700 = local write "New: VT-Sat"(w1397) -> ()
            n701 = local write "Calc: Trap Density-STS"(w1399) -> ()
            n702 = local write "New: Trap Density-STS"(w1399) -> ()
            n703 = local write "New: Trap Density-VT"(w1400) -> ()
            n704 = local write "New: VT-Lin"(w1402) -> ()
            n705 = local write "Sqrt-Lin"(w1388) -> ()
            n706 = local write "New: Mobility-Sat"(w1404) -> ()
            n707 = local write "New: Mobility-Lin"(w1403) -> ()
            n708 = Decimate 1D Array(w1415) -> (w1474:cluster{dbl[], dbl[]}[])  [unwired: 1 out]
            n709 = Index Array(array=w1496, index=w1495) -> (element=w1480:i32)
            n710 = Decimate 1D Array(w1387) -> (w1484:cluster{dbl[], dbl[]}[])  [unwired: 1 out]
            n711 = Array To Cluster(array=w1413) -> (cluster=w1412:T10)
            n712 = Array Subset(array=w1497, index (row)=w1495, index (col)=w1495, length (col)=3) -> (w1498:string[][])  [unwired: 1 in]
            n713 = Array To Cluster(array=w1474) -> (cluster=w1472:T10)
            n714 = Array To Cluster(array=w1484) -> (cluster=w1486:T10)
            n715 = Reshape Array(w1498, w1480) -> (w1487:string[])
            n716 = Subtract(x=w1480, y=20) -> (x-y=w1479:i32)
            n717 = Unbundle(w1412) -> ("[0]"=w1409:cluster{dbl[], dbl[]})  [unwired: 8 out]
            n718 = property on="Sat-Trans Slider" class="Slide (strict)"("Scale.Maximum"=w1479) -> ()  [unwired: 2 in, 2 out]
            n719 = local read "Num Pts"() -> (w1406:dbl)
            n720 = Unbundle(w1472) -> ("[0]"=w1473:cluster{dbl[], dbl[]})  [unwired: 8 out]
            n721 = Unbundle(w1486) -> ("[0]"=w1485:cluster{dbl[], dbl[]})  [unwired: 8 out]
            n722 = Unbundle(w1409) -> (w1408:dbl[], w1407:dbl[])
            n723 = Search 1D Array(1D array=w1487, element="Index:") -> (index of element=w1492:i32)  [unwired: 1 in]
            n724 = Increment(x=w1492) -> (x+1=w1493:i32)
            n725 = Unbundle(w1473) -> (w1471:dbl[], w1470:dbl[])
            n726 = Unbundle(w1485) -> (w1478:dbl[], w1477:dbl[])
            n727 = Array Subset(array=w1408, index=w1405, length=w1406) -> (w1410:dbl[])
            n728 = Array Subset(array=w1407, index=w1405, length=w1406) -> (w1411:dbl[])
            n729 = local read "Image Folder"() -> (w1446:path)
            n730 = local write "Lin-Vg Array-Used"(w1410) -> ()
            n731 = Array Subset(array=w1471, index=w1416, length=w1417) -> (w1476:dbl[])
            n732 = Array Subset(array=w1470, index=w1416, length=w1417) -> (w1475:dbl[])
            n733 = Array Subset(array=w1478, index=w1418, length=w1420) -> (w1483:dbl[])
            n734 = Array Subset(array=w1477, index=w1418, length=w1420) -> (w1482:dbl[])
            n735 = local write "Lin Id-Used"(w1411) -> ()
            n736 = Index Array(array=w1487, index=w1493) -> (element=w1453:string)
            n737 = local write "Sat Vg Array-Used"(w1483) -> ()
            n738 = local write "Vg Array-Log-Used"(w1475) -> ()
            n739 = local write "Sat Id-Log-Used"(w1476) -> ()
            n740 = local write "Sat Id-Used"(w1482) -> ()
            n741 = local write "Index"(w1453) -> ()
            n742 = List Folder(path=w1446, error in=w1457) -> (filenames=w1489:string[], error out=w1456:errorcluster)  [unwired: 2 in, 2 out]
            n743 = Build Path(base path=w1446, name or relative path="ROI") -> (appended path=w1454:path)
            n744 = invoke on="Image Out" class="ImageControl" method="Clear ROI"(error in=w1456) -> (error out=w1460:errorcluster)  [unwired: 2 in, 2 out]
            n745 = while {
              tunnel: w1489 -> [w1522]
              tunnel: w1453 -> [w1520]
              tunnel: [w1519] -> w1488
              tunnel: w1480 -> [w1518]
              i -> [w1519]
              stop <- w1515 stop-if-true
              n746 = Index Array(array=w1522, index=w1519) -> (element=w1523:string)
              n747 = xnode "Match Regular Expression"("input string"=w1523, "regular expression"=w1520) -> ("whole match"=w1521:string)  [unwired: 4 in, 4 out]
              n748 = Equal?(x=w1521, y=w1520) -> (x = y?=w1517:bool)
              n749 = Equal?(x=w1518, y=w1519) -> (x = y?=w1516:bool)
              n750 = Or(x=w1517, y=w1516) -> (x .or. y?=w1515:bool)
            }
            n751 = Build Path(base path=w1454, name or relative path=w1453) -> (appended path=w1452:path)
            n752 = call <vilib>:"Check if File or Folder Exists.vi"("error in (no error)"=w1460, "path"=w1452) -> ("file or folder exists?"=w1458:bool, "dup path"=w1459:path)  [unwired: 7 in, 1 out]
            n753 = case shown="True" w1458 {
              tunnel: w1459 -> [_ w1510]
              frame False {
              }
              frame True {
                n754 = Read from Text File(file (use dialog)=w1510) -> (text=w1514:string)  [unwired: 3 in, 3 out]
                n755 = property on="Image Out" class="ImageControl"() -> ("ROI"=w1511:T11)  [unwired: 2 in, 2 out]
                n756 = Unflatten From String(type=w1511, binary string=w1514) -> (value=w1512:T11, error out=w1513:errorcluster)  [unwired: 3 in, 1 out]
                n757 = property on="Image Out" class="ImageControl"(error in=w1513, "ROI"=w1512) -> ()  [unwired: 1 in, 2 out]
              }
            }
            n758 = Index Array(array=w1489, index=w1488) -> (element=w1462:string)
            n759 = local write "Image Name"(w1462) -> ()
            n760 = Empty String/Path?(string/path=w1462) -> (empty?=w1469:bool)
            n761 = Build Path(base path=w1446, name or relative path=w1462) -> (appended path=w1461:path)
            n762 = local read "No Image File"() -> (w1468:path)
            n763 = Select(t=w1468, s=w1469, f=w1461) -> (s? t:f=w1463:path)
            n764 = call <vilib>:"Get File Extension.vi"("file"=w1463) -> ("lowercase file extension"=w1465:string)  [unwired: 7 in, 3 out]
            n765 = local write "Image File"(w1463) -> ()
            n766 = local write "String"(w1465) -> ()
            n767 = Search 1D Array(1D array=string[] ["bmp", "jpeg", "png", "jpg", "gif"], element=w1465) -> (index of element=w1464:i32)  [unwired: 1 in]
            n768 = call "Vision Acquisition5"("Image Path"=w1463) -> ("Image Out"=w1467:T2)  [unwired: 25 in, 1 out]
            n769 = Less Than 0?(x=w1464) -> ()  [unwired: 1 out]
            n770 = local write "Image Out"(w1467) -> ()
            n771 = local write "Image Out 2"(w1467) -> ()
          }
          event "Save Changes? 3": Mouse Down {
            n772 = event-data() -> ()  [unwired: 1 in, 7 out]
            n773 = local read "Image Folder"() -> (w1639:path)
            n774 = Build Path(base path=w1639, name or relative path="ROI") -> (appended path=w1646:path)
            n775 = call <vilib>:"Check if File or Folder Exists.vi"("path"=w1646) -> ("file or folder exists?"=w1648:bool, "dup path"=w1645:path)  [unwired: 8 in, 1 out]
            n776 = case shown="False" w1648 {
              tunnel: w1645 -> [w1650 w1651]
              tunnel: [w1649 w1651] -> w1640
              frame False {
                n777 = Create Folder(path (use dialog)=w1650) -> (created path=w1649:path)  [unwired: 2 in, 2 out]
              }
              frame True {
              }
            }
            n778 = local read "Index"() -> (w1642:string)
            n779 = property on="Image Out" class="ImageControl"() -> ("ROI"=w1644:T11)  [unwired: 2 in, 2 out]
            n780 = Build Path(base path=w1640, name or relative path=w1642) -> (appended path=w1641:path)
            n781 = Flatten To String(anything=w1644) -> (data string=w1643:string)  [unwired: 3 in, 2 out]
            n782 = Write to Text File(file (use dialog)=w1641, text=w1643) -> ()  [unwired: 2 in, 3 out]
          }
          event "Next Sqrt Sat": Mouse Down {
            n783 = event-data() -> ()  [unwired: 1 in, 5 out]
            n784 = local read "Sqrt-Sat"() -> (w1664:cluster{dbl[], dbl[]}[])
            n785 = Decimate 1D Array(w1664) -> (w1660:cluster{dbl[], dbl[]}[], w1659:cluster{dbl[], dbl[]}[])
            n786 = Array To Cluster(array=w1660) -> (cluster=w1670:T10)
            n787 = local read "MobVi Index"() -> (w1666:dbl)
            n788 = Unbundle(w1670) -> ("[0]"=w1669:cluster{dbl[], dbl[]})  [unwired: 8 out]
            n789 = local read "Num Pts"() -> (w1665:dbl)
            n790 = Unbundle(w1669) -> (w1668:dbl[], w1667:dbl[])
            n791 = Increment(x=w1666) -> (x+1=w1661:dbl)
            n792 = local read "New: Dielectric"() -> (w1655:dbl)
            n793 = local read "New: Length"() -> (w1654:dbl)
            n794 = local read "New: Width"() -> (w1653:dbl)
            n795 = local write "MobVi Index"(w1661) -> ()
            n796 = Array Subset(array=w1668, index=w1661, length=w1665) -> (w1657:dbl[])
            n797 = Array Subset(array=w1667, index=w1661, length=w1665) -> (w1656:dbl[])
            n798 = local write "Sat Vg Array-Used"(w1657) -> ()
            n799 = local write "Sat Id-Used"(w1656) -> ()
            n800 = call "Mobility-Vt-Used Pts_Saturation.vi"("Width"=w1653, "Length"=w1654, "Dielectric (d)"=w1655, "Sat Id Used"=w1656, "Vg Used"=w1657) -> ("Vt"=w1652:dbl, "Mobility"=w1658:dbl)  [unwired: 4 in, 1 out]
            n801 = Bundle(w1657, w1656) -> (w1663:cluster{dbl[], dbl[]})  [unwired: 1 in]
            n802 = Build Array (concatenate)(w1660, w1659, w1663) -> (w1662:cluster{dbl[], dbl[]}[])
            n803 = local write "New: Mobility-Sat"(w1658) -> ()
            n804 = local write "New: VT-Sat"(w1652) -> ()
            n805 = local write "Sqrt-Sat"(w1662) -> ()
          }
          event "Next Log Sat": Mouse Down {
            n806 = event-data() -> ()  [unwired: 1 in, 7 out]
            n807 = local read "Log-Sat"() -> (w1679:cluster{dbl[], dbl[]}[])
            n808 = Decimate 1D Array(w1679) -> (w1675:cluster{dbl[], dbl[]}[], w1674:cluster{dbl[], dbl[]}[])
            n809 = Array To Cluster(array=w1675) -> (cluster=w1685:T10)
            n810 = local read "Index 2"() -> (w1681:dbl)
            n811 = local read "NumPoints Log"() -> (w1680:dbl)
            n812 = Unbundle(w1685) -> ("[0]"=w1684:cluster{dbl[], dbl[]})  [unwired: 8 out]
            n813 = Unbundle(w1684) -> (w1683:dbl[], w1682:dbl[])
            n814 = Increment(x=w1681) -> (x+1=w1676:dbl)
            n815 = local write "Index 2"(w1676) -> ()
            n816 = Array Subset(array=w1682, index=w1676, length=w1680) -> (w1671:dbl[])
            n817 = Array Subset(array=w1683, index=w1676, length=w1680) -> (w1672:dbl[])
            n818 = call "STS-Used.vi"("Id Used"=w1672, "Vg-Used"=w1671) -> ("STS"=w1673:dbl)  [unwired: 9 in]
            n819 = Bundle(w1672, w1671) -> (w1678:cluster{dbl[], dbl[]})  [unwired: 1 in]
            n820 = local write "Vg Array-Log-Used"(w1671) -> ()
            n821 = local write "Sat Id-Log-Used"(w1672) -> ()
            n822 = local write "New: STS"(w1673) -> ()
            n823 = Build Array (concatenate)(w1675, w1674, w1678) -> (w1677:cluster{dbl[], dbl[]}[])
            n824 = local write "Log-Sat"(w1677) -> ()
          }
          event "Previous Log Sat": Mouse Down {
            n825 = event-data() -> ()  [unwired: 1 in, 7 out]
            n826 = local read "Log-Sat"() -> (w1695:cluster{dbl[], dbl[]}[])
            n827 = Decimate 1D Array(w1695) -> (w1692:cluster{dbl[], dbl[]}[], w1691:cluster{dbl[], dbl[]}[])
            n828 = Array To Cluster(array=w1692) -> (cluster=w1700:T10)
            n829 = local read "Index 2"() -> (w1688:dbl)
            n830 = local read "NumPoints Log"() -> (w1696:dbl)
            n831 = Unbundle(w1700) -> ("[0]"=w1699:cluster{dbl[], dbl[]})  [unwired: 8 out]
            n832 = Unbundle(w1699) -> (w1698:dbl[], w1697:dbl[])
            n833 = Decrement(x=w1688) -> (x-1=w1689:dbl)
            n834 = local write "Index 2"(w1689) -> ()
            n835 = Array Subset(array=w1698, index=w1689, length=w1696) -> (w1686:dbl[])
            n836 = Array Subset(array=w1697, index=w1689, length=w1696) -> (w1687:dbl[])
            n837 = local write "Vg Array-Log-Used"(w1687) -> ()
            n838 = local write "Sat Id-Log-Used"(w1686) -> ()
            n839 = Bundle(w1686, w1687) -> (w1694:cluster{dbl[], dbl[]})  [unwired: 1 in]
            n840 = call "STS-Used.vi"("Id Used"=w1686, "Vg-Used"=w1687) -> ("STS"=w1690:dbl)  [unwired: 9 in]
            n841 = Build Array (concatenate)(w1692, w1691, w1694) -> (w1693:cluster{dbl[], dbl[]}[])
            n842 = local write "New: STS"(w1690) -> ()
            n843 = local write "Log-Sat"(w1693) -> ()
          }
          event "Previous Sqrt Sat": Mouse Down {
            n844 = event-data() -> ()  [unwired: 1 in, 5 out]
            n845 = local read "Sqrt-Sat"() -> (w1714:cluster{dbl[], dbl[]}[])
            n846 = Decimate 1D Array(w1714) -> (w1711:cluster{dbl[], dbl[]}[], w1710:cluster{dbl[], dbl[]}[])
            n847 = Array To Cluster(array=w1711) -> (cluster=w1719:T10)
            n848 = local read "MobVi Index"() -> (w1709:dbl)
            n849 = Unbundle(w1719) -> ("[0]"=w1718:cluster{dbl[], dbl[]})  [unwired: 8 out]
            n850 = local read "Num Pts"() -> (w1715:dbl)
            n851 = Unbundle(w1718) -> (w1717:dbl[], w1716:dbl[])
            n852 = Decrement(x=w1709) -> (x-1=w1708:dbl)
            n853 = local read "New: Dielectric"() -> (w1702:dbl)
            n854 = local read "New: Length"() -> (w1703:dbl)
            n855 = local read "New: Width"() -> (w1704:dbl)
            n856 = local write "MobVi Index"(w1708) -> ()
            n857 = Array Subset(array=w1717, index=w1708, length=w1715) -> (w1707:dbl[])
            n858 = Array Subset(array=w1716, index=w1708, length=w1715) -> (w1706:dbl[])
            n859 = local write "Sat Vg Array-Used"(w1707) -> ()
            n860 = local write "Sat Id-Used"(w1706) -> ()
            n861 = call "Mobility-Vt-Used Pts_Linear.vi"("Width"=w1704, "Length"=w1703, "Dielectric (d)"=w1702, "Sat Id Used"=w1706, "Vg Used"=w1707) -> ("Vt"=w1701:dbl, "Mobility"=w1705:dbl)  [unwired: 4 in, 1 out]
            n862 = Bundle(w1707, w1706) -> (w1713:cluster{dbl[], dbl[]})  [unwired: 1 in]
            n863 = local write "New: VT-Sat"(w1701) -> ()
            n864 = Build Array (concatenate)(w1711, w1710, w1713) -> (w1712:cluster{dbl[], dbl[]}[])
            n865 = local write "New: Mobility-Sat"(w1705) -> ()
            n866 = local write "Sqrt-Sat"(w1712) -> ()
          }
          event "Sat-Trans Slider": Value Change {
            n867 = event-data() -> ()  [unwired: 1 in, 5 out]
            n868 = local read "Sqrt-Sat"() -> (w1732:cluster{dbl[], dbl[]}[])
            n869 = Decimate 1D Array(w1732) -> (w1729:cluster{dbl[], dbl[]}[], w1728:cluster{dbl[], dbl[]}[])
            n870 = Array To Cluster(array=w1729) -> (cluster=w1737:T10)
            n871 = Unbundle(w1737) -> ("[0]"=w1736:cluster{dbl[], dbl[]})  [unwired: 8 out]
            n872 = local read "Sat-Trans Slider"() -> (w1721:dbl)
            n873 = local read "Num Pts"() -> (w1733:dbl)
            n874 = Unbundle(w1736) -> (w1735:dbl[], w1734:dbl[])
            n875 = local read "New: Dielectric"() -> (w1722:dbl)
            n876 = local read "New: Length"() -> (w1723:dbl)
            n877 = local read "New: Width"() -> (w1724:dbl)
            n878 = local write "MobVi Index"(w1721) -> ()
            n879 = Array Subset(array=w1735, index=w1721, length=w1733) -> (w1727:dbl[])
            n880 = Array Subset(array=w1734, index=w1721, length=w1733) -> (w1726:dbl[])
            n881 = local write "Sat Vg Array-Used"(w1727) -> ()
            n882 = local write "Sat Id-Used"(w1726) -> ()
            n883 = call "Mobility-Vt-Used Pts_Linear.vi"("Width"=w1724, "Length"=w1723, "Dielectric (d)"=w1722, "Sat Id Used"=w1726, "Vg Used"=w1727) -> ("Vt"=w1720:dbl, "Mobility"=w1725:dbl)  [unwired: 4 in, 1 out]
            n884 = Bundle(w1727, w1726) -> (w1731:cluster{dbl[], dbl[]})  [unwired: 1 in]
            n885 = local write "New: VT-Sat"(w1720) -> ()
            n886 = Build Array (concatenate)(w1729, w1728, w1731) -> (w1730:cluster{dbl[], dbl[]}[])
            n887 = local write "New: Mobility-Sat"(w1725) -> ()
            n888 = local write "Sqrt-Sat"(w1730) -> ()
          }
          event "Sat-Log Slider": Value Change {
            n889 = event-data() -> ()  [unwired: 1 in, 5 out]
            n890 = local read "Log-Sat"() -> (w1746:cluster{dbl[], dbl[]}[])
            n891 = Decimate 1D Array(w1746) -> (w1743:cluster{dbl[], dbl[]}[], w1742:cluster{dbl[], dbl[]}[])
            n892 = Array To Cluster(array=w1743) -> (cluster=w1751:T10)
            n893 = Unbundle(w1751) -> ("[0]"=w1750:cluster{dbl[], dbl[]})  [unwired: 8 out]
            n894 = local read "NumPoints Log"() -> (w1747:dbl)
            n895 = local read "Sat-Log Slider"() -> (w1741:dbl)
            n896 = Unbundle(w1750) -> (w1749:dbl[], w1748:dbl[])
            n897 = local write "Index 2"(w1741) -> ()
            n898 = Array Subset(array=w1749, index=w1741, length=w1747) -> (w1739:dbl[])
            n899 = Array Subset(array=w1748, index=w1741, length=w1747) -> (w1738:dbl[])
            n900 = local write "Vg Array-Log-Used"(w1738) -> ()
            n901 = local write "Sat Id-Log-Used"(w1739) -> ()
            n902 = call "STS-Used.vi"("Id Used"=w1739, "Vg-Used"=w1738) -> ("STS"=w1740:dbl)  [unwired: 9 in]
            n903 = Bundle(w1739, w1738) -> (w1745:cluster{dbl[], dbl[]})  [unwired: 1 in]
            n904 = local write "New: STS"(w1740) -> ()
            n905 = Build Array (concatenate)(w1743, w1742, w1745) -> (w1744:cluster{dbl[], dbl[]}[])
            n906 = local write "Log-Sat"(w1744) -> ()
          }
          event "Save Changes?": Mouse Down {
            n907 = event-data() -> ()  [unwired: 1 in, 5 out]
            n908 = flat-sequence {
              tunnel: [w1758] -> w1756
              tunnel: [w1766] -> w1755
              tunnel: [w1759] -> w1754
              tunnel: w1756 -> [w2298]
              tunnel: w1755 -> [w2295]
              tunnel: [w2296] -> w1753
              tunnel: w1754 -> [w2296]
              tunnel: [w2295] -> w1752
              tunnel: w1753 -> [w2303]
              tunnel: w1752 -> [w2302]
              frame #0 {
                n909 = Wait (ms)(milliseconds to wait=1) -> ()  [unwired: 1 out]
              }
              frame #1 {
                n910 = local read "Transfer File"() -> (w1758:path)
                n911 = local read "New: Temp"() -> (w1760:dbl)
                n912 = local read "New: Length"() -> (w1764:dbl)
                n913 = local read "New: Width"() -> (w1762:dbl)
                n914 = To Single Precision Float(number=w1760) -> (single precision float=w1761:sgl)
                n915 = Number To Decimal String(number=w1761) -> (decimal integer string=w1769:string)  [unwired: 1 in]
                n916 = To Single Precision Float(number=w1762) -> (single precision float=w1763:sgl)
                n917 = To Single Precision Float(number=w1764) -> (single precision float=w1765:sgl)
                n918 = local read "Index"() -> (w1774:string)
                n919 = Strip Path(path=w1758) -> (stripped path=w1779:path)  [unwired: 1 out]
                n920 = Number To Decimal String(number=w1765) -> (decimal integer string=w1772:string)  [unwired: 1 in]
                n921 = Number To Decimal String(number=w1763) -> (decimal integer string=w1773:string)  [unwired: 1 in]
                n922 = Concatenate Strings("_", w1769, "K") -> (w1767:string)
                n923 = call "Build Text"("Temp"=w1767, "Index"=w1774, "Length"=w1772, "Width"=w1773) -> ("Result"=w1775:string)  [unwired: 10 in, 1 out]
                n924 = flat-sequence {
                  tunnel: [w2252] -> w1771
                  tunnel: w1771 -> [w2269]
                  frame #0 {
                    # "Makes Empty File for Transformer Data"
                    n925 = local read "Transfer Folder"() -> (w2241:path)
                    n926 = Build Path(base path=w2241, name or relative path="Stats") -> (appended path=w2243:path)
                    n927 = call <vilib>:"Check if File or Folder Exists.vi"("path"=w2243) -> ("file or folder exists?"=w2244:bool, "dup path"=w2245:path)  [unwired: 8 in, 1 out]
                    n928 = case shown="False" w2244 {
                      tunnel: [w2249 w2251] -> w2246
                      tunnel: w2245 -> [w2250 w2251]
                      frame False {
                        n929 = Create Folder(path (use dialog)=w2250) -> (created path=w2249:path)  [unwired: 2 in, 2 out]
                      }
                      frame True {
                      }
                    }
                    n930 = Build Path(base path=w2246, name or relative path="Tranformer Data.txt") -> (appended path=w2248:path)
                    n931 = call-poly <vilib>:"Write To Spreadsheet File.vi"("append to file? (new file:F)"=TRUE, "file path (dialog if empty)"=w2248) -> ()  [unwired: 6 in, 1 out]
                  }
                  frame #1 {
                    # "Adds Headers if they don't exist"
                    n932 = local read "Transfer Folder"() -> (w2258:path)
                    n933 = Concatenate Strings("Stats\\", "Tranformer Data.txt") -> (w2259:string)
                    n934 = Build Path(base path=w2258, name or relative path=w2259) -> (appended path=w2252:path)
                    n935 = call-poly <vilib>:"Read From Spreadsheet File.vi"("file path (dialog if empty)"=w2252) -> ("first row"=w2257:string[])  [unwired: 6 in, 4 out]
                    n936 = Search 1D Array(1D array=w2257, element="DeviceID") -> (index of element=w2255:i32)  [unwired: 1 in]
                    n937 = Equal?(x=w2255, y=0) -> (x = y?=w2253:bool)
                    n938 = case shown="False" w2253 {
                      tunnel: w2252 -> [w2263 _]
                      frame False {
                        n939 = local read "Transformer \nHeaders"() -> (w2262:string[])
                        n940 = call-poly <vilib>:"Write To Spreadsheet File.vi"("1D data"=w2262, "file path (dialog if empty)"=w2263) -> ()  [unwired: 6 in, 1 out]
                      }
                      frame True {
                      }
                    }
                  }
                  frame #2 {
                    # "Adds current device if it doesn't exist"
                    n941 = local read "Current \nRecord"() -> (w2268:string[])
                    n942 = Index Array(array=w2268, index=0) -> (element=w2267:string)
                    n943 = local read "Transfer Folder"() -> (w2271:path)
                    n944 = Concatenate Strings("Stats\\", "Tranformer Data.txt") -> (w2272:string)
                    n945 = local write "Current Device ID"(w2267) -> ()
                    n946 = local read "Current Device ID"() -> (w2277:string)
                    n947 = Build Path(base path=w2271, name or relative path=w2272) -> (appended path=w2270:path)
                    n948 = call-poly <vilib>:"Read From Spreadsheet File.vi"("file path (dialog if empty)"=w2270) -> ("all rows"=w2264:string[][])  [unwired: 6 in, 4 out]
                    n949 = Index Array(array=w2264, index (col)=0) -> (element=w2265:string[])  [unwired: 1 in]
                    n950 = Search 1D Array(1D array=w2265, element=w2277) -> (index of element=w2266:i32)  [unwired: 1 in]
                    n951 = Equal?(x=w2266, y=-1) -> (x = y?=w2279:bool)
                    n952 = case shown="False" w2279 {
                      tunnel: w2269 -> [w2282 w2293]
                      tunnel: w2266 -> [w2285 _]
                      tunnel: w2264 -> [w2286 _]
                      frame False {
                        n953 = local read "Current \nRecord"() -> (w2284:string[])
                        n954 = Replace Array Subset(array=w2286, new element=w2284, index (row)=w2285) -> (w2283:string[][])  [unwired: 1 in]
                        n955 = flat-sequence {
                          tunnel: w2282 -> [w2287]
                          tunnel: w2283 -> [w2288]
                          tunnel: [w2288] -> w2281
                          tunnel: [w2287] -> w2280
                          tunnel: w2281 -> [w2290]
                          tunnel: w2280 -> [w2289]
                          frame #0 {
                            n956 = Delete(path (use dialog)=w2287) -> ()  [unwired: 4 in, 3 out]
                          }
                          frame #1 {
                            n957 = call-poly <vilib>:"Write To Spreadsheet File.vi"("append to file? (new file:F)"=TRUE, "2D data"=w2290, "file path (dialog if empty)"=w2289) -> ()  [unwired: 5 in, 1 out]
                          }
                        }
                      }
                      frame True {
                        n958 = local read "Current \nRecord"() -> (w2292:string[])
                        n959 = call-poly <vilib>:"Write To Spreadsheet File.vi"("append to file? (new file:F)"=TRUE, "1D data"=w2292, "file path (dialog if empty)"=w2293) -> ()  [unwired: 5 in, 1 out]
                      }
                    }
                  }
                }
                n960 = Path To String(path=w1779) -> (string=w1777:string)
                n961 = stacked-sequence {
                  tunnel: [_ _ _ _ _ _ _ _ _ _ _ _ _ w2212] -> w1759
                  tunnel: w1758 -> [w1781 _ _ _ _ _ _ _ _ _ _ _ _ _]
                  frame #0 {
                    n962 = call-poly <vilib>:"Read From Spreadsheet File.vi"("file path (dialog if empty)"=w1781) -> ("all rows"=w1780:string[][])  [unwired: 6 in, 4 out]
                    n963 = Array Size(array=w1780) -> (size(s)=w1785:i32[])
                    n964 = Array Subset(array=w1780, index (row)=0, index (col)=0, length (col)=3) -> (w1789:string[][])  [unwired: 1 in]
                    n965 = Index Array(array=w1785, index=0) -> (element=w1783:i32)
                    n966 = Reshape Array(w1789, w1783) -> (w1782:string[])
                    n967 = Search 1D Array(1D array=w1782, element="Dielectric (nm):") -> (index of element=w1792:i32)  [unwired: 1 in]
                    n968 = Equal?(x=w1792, y=-1) -> (x = y?=w1791:bool)
                    n969 = case shown="False" w1791 {
                      tunnel: w1780 -> [w1800 w1804]
                      tunnel: w1792 -> [w1796 _]
                      tunnel: [w1795 w1804] -> w1790
                      frame False {
                        n970 = local read "New: Dielectric"() -> (w1802:dbl)
                        n971 = Number To Fractional String(number=w1802) -> (F-format string=w1797:string)  [unwired: 3 in]
                        n972 = Divide(x=w1796, y=3) -> (x/y=w1799:dbl)
                        n973 = To Word Integer(number=w1799) -> (16bit integer=w1798:i16)
                        n974 = Replace Array Subset(array=w1800, new element=w1797, index (row)=w1798, index (col)=1) -> (w1795:string[][])
                      }
                      frame True {
                      }
                    }
                    n975 = local write "Save1 Array"(w1790) -> ()
                  }
                  frame #1 {
                    n976 = local read "Save1 Array"() -> (w1806:string[][])
                    n977 = Array Size(array=w1806) -> (size(s)=w1809:i32[])
                    n978 = Array Subset(array=w1806, index (row)=0, index (col)=0, length (col)=3) -> (w1813:string[][])  [unwired: 1 in]
                    n979 = Index Array(array=w1809, index=0) -> (element=w1807:i32)
                    n980 = Reshape Array(w1813, w1807) -> (w1805:string[])
                    n981 = Search 1D Array(1D array=w1805, element="Comments:") -> (index of element=w1816:i32)  [unwired: 1 in]
                    n982 = Equal?(x=w1816, y=-1) -> (x = y?=w1815:bool)
                    n983 = case shown="False" w1815 {
                      tunnel: w1806 -> [w1824 w1827]
                      tunnel: w1816 -> [w1821 _]
                      tunnel: [w1820 w1827] -> w1814
                      frame False {
                        n984 = local read "Comments:"() -> (w1819:string)
                        n985 = Divide(x=w1821, y=3) -> (x/y=w1823:dbl)
                        n986 = To Word Integer(number=w1823) -> (16bit integer=w1822:i16)
                        n987 = Replace Array Subset(array=w1824, new element=w1819, index (row)=w1822, index (col)=1) -> (w1820:string[][])
                      }
                      frame True {
                      }
                    }
                    n988 = local write "Save1 Array"(w1814) -> ()
                  }
                  frame #2 {
                    n989 = local read "Save1 Array"() -> (w1829:string[][])
                    n990 = Array Size(array=w1829) -> (size(s)=w1832:i32[])
                    n991 = Array Subset(array=w1829, index (row)=0, index (col)=0, length (col)=3) -> (w1836:string[][])  [unwired: 1 in]
                    n992 = Index Array(array=w1832, index=0) -> (element=w1830:i32)
                    n993 = Reshape Array(w1836, w1830) -> (w1828:string[])
                    n994 = Search 1D Array(1D array=w1828, element="Length (um):") -> (index of element=w1839:i32)  [unwired: 1 in]
                    n995 = Equal?(x=w1839, y=-1) -> (x = y?=w1838:bool)
                    n996 = case shown="False" w1838 {
                      tunnel: w1829 -> [w1849 w1852]
                      tunnel: w1839 -> [w1846 _]
                      tunnel: [w1845 w1852] -> w1837
                      frame False {
                        n997 = local read "New: Length"() -> (w1842:dbl)
                        n998 = Divide(x=w1846, y=3) -> (x/y=w1848:dbl)
                        n999 = Format Value(format string="%#g", value (0)=w1842) -> (output string=w1843:string)  [unwired: 1 in]
                        n1000 = To Word Integer(number=w1848) -> (16bit integer=w1847:i16)
                        n1001 = Replace Array Subset(array=w1849, new element=w1843, index (row)=w1847, index (col)=1) -> (w1845:string[][])
                      }
                      frame True {
                      }
                    }
                    n1002 = local write "Save1 Array"(w1837) -> ()
                  }
                  frame #3 {
                    n1003 = local read "Save1 Array"() -> (w1854:string[][])
                    n1004 = Array Size(array=w1854) -> (size(s)=w1859:i32[])
                    n1005 = Array Subset(array=w1854, index (row)=0, index (col)=0, length (col)=3) -> (w1855:string[][])  [unwired: 1 in]
                    n1006 = Index Array(array=w1859, index=0) -> (element=w1861:i32)
                    n1007 = Reshape Array(w1855, w1861) -> (w1853:string[])
                    n1008 = Search 1D Array(1D array=w1853, element="Width (um):") -> (index of element=w1864:i32)  [unwired: 1 in]
                    n1009 = Equal?(x=w1864, y=-1) -> (x = y?=w1863:bool)
                    n1010 = case shown="False" w1863 {
                      tunnel: w1864 -> [w1872 _]
                      tunnel: w1854 -> [w1871 w1877]
                      tunnel: [w1870 w1877] -> w1862
                      frame False {
                        n1011 = local read "New: Width"() -> (w1867:dbl)
                        n1012 = Divide(x=w1872, y=3) -> (x/y=w1874:dbl)
                        n1013 = To Word Integer(number=w1874) -> (16bit integer=w1873:i16)
                        n1014 = Format Value(format string="%#g", value (0)=w1867) -> (output string=w1868:string)  [unwired: 1 in]
                        n1015 = Replace Array Subset(array=w1871, new element=w1868, index (row)=w1873, index (col)=1) -> (w1870:string[][])
                      }
                      frame True {
                      }
                    }
                    n1016 = local write "Save1 Array"(w1862) -> ()
                  }
                  frame #4 {
                    w1887 = "Sample Temp (K):"
                    n1017 = local read "Save1 Array"() -> (w1879:string[][])
                    n1018 = Array Size(array=w1879) -> (size(s)=w1884:i32[])
                    n1019 = Array Subset(array=w1879, index (row)=0, index (col)=0, length (col)=3) -> (w1880:string[][])  [unwired: 1 in]
                    n1020 = Index Array(array=w1884, index=0) -> (element=w1886:i32)
                    n1021 = Reshape Array(w1880, w1886) -> (w1878:string[])
                    n1022 = Search 1D Array(1D array=w1878, element=w1887) -> (index of element=w1890:i32)  [unwired: 1 in]
                    n1023 = Equal?(x=w1890, y=-1) -> (x = y?=w1889:bool)
                    n1024 = case shown="True" w1889 {
                      tunnel: w1879 -> [w1899 w1913]
                      tunnel: w1890 -> [w1896 _]
                      tunnel: [w1895 w1912] -> w1888
                      tunnel: w1878 -> [_ w1915]
                      tunnel: w1887 -> [_ w1902]
                      frame False {
                        n1025 = local read "New: Temp"() -> (w1893:dbl)
                        n1026 = Divide(x=w1896, y=3) -> (x/y=w1898:dbl)
                        n1027 = Format Value(format string="%#g", value (0)=w1893) -> (output string=w1892:string)  [unwired: 1 in]
                        n1028 = To Word Integer(number=w1898) -> (16bit integer=w1897:i16)
                        n1029 = Replace Array Subset(array=w1899, new element=w1892, index (row)=w1897, index (col)=1) -> (w1895:string[][])
                      }
                      frame True {
                        n1030 = local read "New: Temp"() -> (w1904:dbl)
                        n1031 = Search 1D Array(1D array=w1915, element="Width (um):") -> (index of element=w1909:i32)  [unwired: 1 in]
                        n1032 = Divide(x=w1909, y=3) -> (x/y=w1910:dbl)
                        n1033 = To Word Integer(number=w1910) -> (16bit integer=w1908:i16)
                        n1034 = Format Value(format string="%#g", value (0)=w1904) -> (output string=w1903:string)  [unwired: 1 in]
                        n1035 = Build Array(w1902, w1903) -> (w1906:string[])
                        n1036 = Increment(x=w1908) -> (x+1=w1907:i16)
                        n1037 = Insert Into Array(array=w1913, index (row)=w1907, new element=w1906) -> (w1912:string[][])  [unwired: 1 in]
                      }
                    }
                    n1038 = local write "Save1 Array"(w1888) -> ()
                  }
                  frame #5 {
                    w1925 = "Mobility-Sat (cm^2/Vs):"
                    n1039 = local read "Save1 Array"() -> (w1917:string[][])
                    n1040 = Array Size(array=w1917) -> (size(s)=w1922:i32[])
                    n1041 = Array Subset(array=w1917, index (row)=0, index (col)=0, length (col)=3) -> (w1918:string[][])  [unwired: 1 in]
                    n1042 = Index Array(array=w1922, index=0) -> (element=w1924:i32)
                    n1043 = Reshape Array(w1918, w1924) -> (w1916:string[])
                    n1044 = Search 1D Array(1D array=w1916, element=w1925) -> (index of element=w1928:i32)  [unwired: 1 in]
                    n1045 = Equal?(x=w1928, y=-1) -> (x = y?=w1927:bool)
                    n1046 = case shown="True" w1927 {
                      tunnel: w1917 -> [w1937 w1945]
                      tunnel: w1928 -> [w1934 _]
                      tunnel: [w1933 w1944] -> w1926
                      tunnel: w1916 -> [_ w1942]
                      tunnel: w1925 -> [_ w1940]
                      frame False {
                        n1047 = local read "New: Mobility-Sat"() -> (w1930:dbl)
                        n1048 = Divide(x=w1934, y=3) -> (x/y=w1936:dbl)
                        n1049 = To Word Integer(number=w1936) -> (16bit integer=w1935:i16)
                        n1050 = Format Value(format string="%#g", value (0)=w1930) -> (output string=w1931:string)  [unwired: 1 in]
                        n1051 = Replace Array Subset(array=w1937, new element=w1931, index (row)=w1935, index (col)=1) -> (w1933:string[][])
                      }
                      frame True {
                        n1052 = local read "New: Mobility-Sat"() -> (w1946:dbl)
                        n1053 = Search 1D Array(1D array=w1942, element="Mobility (cm^2/Vs):") -> (index of element=w1949:i32)  [unwired: 1 in]
                        n1054 = Divide(x=w1949, y=3) -> (x/y=w1950:dbl)
                        n1055 = To Word Integer(number=w1950) -> (16bit integer=w1941:i16)
                        n1056 = Format Value(format string="%#g", value (0)=w1946) -> (output string=w1943:string)  [unwired: 1 in]
                        n1057 = Build Array(w1940, w1943) -> (w1948:string[])
                        n1058 = Replace Array Subset(array=w1945, new element=w1948, index (row)=w1941) -> (w1944:string[][])  [unwired: 1 in]
                      }
                    }
                    n1059 = local write "Save1 Array"(w1926) -> ()
                  }
                  frame #6 {
                    w1962 = "Mobility-Lin (cm^2/Vs):"
                    n1060 = local read "Save1 Array"() -> (w1953:string[][])
                    n1061 = Array Size(array=w1953) -> (size(s)=w1959:i32[])
                    n1062 = Array Subset(array=w1953, index (row)=0, index (col)=0, length (col)=3) -> (w1955:string[][])  [unwired: 1 in]
                    n1063 = Index Array(array=w1959, index=0) -> (element=w1961:i32)
                    n1064 = Reshape Array(w1955, w1961) -> (w1954:string[])
                    n1065 = Search 1D Array(1D array=w1954, element=w1962) -> (index of element=w1965:i32)  [unwired: 1 in]
                    n1066 = Equal?(x=w1965, y=-1) -> (x = y?=w1964:bool)
                    n1067 = case shown="True" w1964 {
                      tunnel: w1953 -> [w1974 w1980]
                      tunnel: w1965 -> [w1971 _]
                      tunnel: [w1970 w1979] -> w1963
                      tunnel: w1954 -> [_ w1978]
                      tunnel: w1962 -> [_ w1977]
                      frame False {
                        n1068 = local read "Calc: Mobility-Lin"() -> (w1967:dbl)
                        n1069 = Divide(x=w1971, y=3) -> (x/y=w1973:dbl)
                        n1070 = To Word Integer(number=w1973) -> (16bit integer=w1972:i16)
                        n1071 = Format Value(format string="%#g", value (0)=w1967) -> (output string=w1968:string)  [unwired: 1 in]
                        n1072 = Replace Array Subset(array=w1974, new element=w1968, index (row)=w1972, index (col)=1) -> (w1970:string[][])
                      }
                      frame True {
                        n1073 = local read "Calc: Mobility-Lin"() -> (w1981:dbl)
                        n1074 = Search 1D Array(1D array=w1978, element="Mobility-Sat (cm^2/Vs):") -> (index of element=w1986:i32)  [unwired: 1 in]
                        n1075 = Divide(x=w1986, y=3) -> (x/y=w1987:dbl)
                        n1076 = To Word Integer(number=w1987) -> (16bit integer=w1985:i16)
                        n1077 = Format Value(format string="%#g", value (0)=w1981) -> (output string=w1990:string)  [unwired: 1 in]
                        n1078 = Build Array(w1977, w1990) -> (w1983:string[])
                        n1079 = Increment(x=w1985) -> (x+1=w1984:i16)
                        n1080 = Insert Into Array(array=w1980, index (row)=w1984, new element=w1983) -> (w1979:string[][])  [unwired: 1 in]
                      }
                    }
                    n1081 = local write "Save1 Array"(w1963) -> ()
                  }
                  frame #7 {
                    w2000 = "On/Off I-Sat:"
                    n1082 = local read "Save1 Array"() -> (w1991:string[][])
                    n1083 = Array Size(array=w1991) -> (size(s)=w1997:i32[])
                    n1084 = Array Subset(array=w1991, index (row)=0, index (col)=0, length (col)=3) -> (w1993:string[][])  [unwired: 1 in]
                    n1085 = Index Array(array=w1997, index=0) -> (element=w1999:i32)
                    n1086 = Reshape Array(w1993, w1999) -> (w1992:string[])
                    n1087 = Search 1D Array(1D array=w1992, element=w2000) -> (index of element=w2003:i32)  [unwired: 1 in]
                    n1088 = Equal?(x=w2003, y=-1) -> (x = y?=w2002:bool)
                    n1089 = case shown="True" w2002 {
                      tunnel: w1991 -> [w2012 w2019]
                      tunnel: w2003 -> [w2009 _]
                      tunnel: [w2008 w2020] -> w2001
                      tunnel: w1992 -> [_ w2017]
                      tunnel: w2000 -> [_ w2015]
                      frame False {
                        n1090 = local read "Calc: On/Off"() -> (w2005:dbl)
                        n1091 = Divide(x=w2009, y=3) -> (x/y=w2011:dbl)
                        n1092 = To Word Integer(number=w2011) -> (16bit integer=w2010:i16)
                        n1093 = Format Value(format string="%#g", value (0)=w2005) -> (output string=w2006:string)  [unwired: 1 in]
                        n1094 = Replace Array Subset(array=w2012, new element=w2006, index (row)=w2010, index (col)=1) -> (w2008:string[][])
                      }
                      frame True {
                        n1095 = local read "Calc: On/Off"() -> (w2021:dbl)
                        n1096 = Search 1D Array(1D array=w2017, element="On/Off Current:") -> (index of element=w2024:i32)  [unwired: 1 in]
                        n1097 = Divide(x=w2024, y=3) -> (x/y=w2025:dbl)
                        n1098 = To Word Integer(number=w2025) -> (16bit integer=w2016:i16)
                        n1099 = Format Value(format string="%#g", value (0)=w2021) -> (output string=w2018:string)  [unwired: 1 in]
                        n1100 = Build Array(w2015, w2018) -> (w2023:string[])
                        n1101 = Replace Array Subset(array=w2019, new element=w2023, index (row)=w2016) -> (w2020:string[][])  [unwired: 1 in]
                      }
                    }
                    n1102 = local write "Save1 Array"(w2001) -> ()
                  }
                  frame #8 {
                    w2037 = "Off I-Sat (A):"
                    n1103 = local read "Save1 Array"() -> (w2028:string[][])
                    n1104 = Array Size(array=w2028) -> (size(s)=w2034:i32[])
                    n1105 = Array Subset(array=w2028, index (row)=0, index (col)=0, length (col)=3) -> (w2030:string[][])  [unwired: 1 in]
                    n1106 = Index Array(array=w2034, index=0) -> (element=w2036:i32)
                    n1107 = Reshape Array(w2030, w2036) -> (w2029:string[])
                    n1108 = Search 1D Array(1D array=w2029, element=w2037) -> (index of element=w2040:i32)  [unwired: 1 in]
                    n1109 = Equal?(x=w2040, y=-1) -> (x = y?=w2039:bool)
                    n1110 = case shown="True" w2039 {
                      tunnel: w2028 -> [w2049 w2055]
                      tunnel: w2040 -> [w2046 _]
                      tunnel: [w2045 w2054] -> w2038
                      tunnel: w2029 -> [_ w2053]
                      tunnel: w2037 -> [_ w2052]
                      frame False {
                        n1111 = local read "Calc: Off I-Sat"() -> (w2044:dbl)
                        n1112 = Divide(x=w2046, y=3) -> (x/y=w2048:dbl)
                        n1113 = Format Value(format string="%#g", value (0)=w2044) -> (output string=w2042:string)  [unwired: 1 in]
                        n1114 = To Word Integer(number=w2048) -> (16bit integer=w2047:i16)
                        n1115 = Replace Array Subset(array=w2049, new element=w2042, index (row)=w2047, index (col)=1) -> (w2045:string[][])
                      }
                      frame True {
                        n1116 = local read "Calc: Off I-Sat"() -> (w2056:dbl)
                        n1117 = Search 1D Array(1D array=w2053, element="On/Off I-Sat:") -> (index of element=w2061:i32)  [unwired: 1 in]
                        n1118 = Divide(x=w2061, y=3) -> (x/y=w2062:dbl)
                        n1119 = To Word Integer(number=w2062) -> (16bit integer=w2060:i16)
                        n1120 = Format Value(format string="%#g", value (0)=w2056) -> (output string=w2065:string)  [unwired: 1 in]
                        n1121 = Build Array(w2052, w2065) -> (w2058:string[])
                        n1122 = Increment(x=w2060) -> (x+1=w2059:i16)
                        n1123 = Insert Into Array(array=w2055, index (row)=w2059, new element=w2058) -> (w2054:string[][])  [unwired: 1 in]
                      }
                    }
                    n1124 = local write "Save1 Array"(w2038) -> ()
                  }
                  frame #9 {
                    w2067 = "Vt-Sat (V):"
                    n1125 = local read "Save1 Array"() -> (w2068:string[][])
                    n1126 = Array Size(array=w2068) -> (size(s)=w2073:i32[])
                    n1127 = Array Subset(array=w2068, index (row)=0, index (col)=0, length (col)=3) -> (w2069:string[][])  [unwired: 1 in]
                    n1128 = Index Array(array=w2073, index=0) -> (element=w2075:i32)
                    n1129 = Reshape Array(w2069, w2075) -> (w2066:string[])
                    n1130 = Search 1D Array(1D array=w2066, element=w2067) -> (index of element=w2078:i32)  [unwired: 1 in]
                    n1131 = Equal?(x=w2078, y=-1) -> (x = y?=w2077:bool)
                    n1132 = case shown="True" w2077 {
                      tunnel: w2068 -> [w2085 w2094]
                      tunnel: w2078 -> [w2081 _]
                      tunnel: [w2080 w2093] -> w2076
                      tunnel: w2067 -> [_ w2092]
                      tunnel: w2066 -> [_ w2091]
                      frame False {
                        n1133 = local read "New: VT-Sat"() -> (w2087:dbl)
                        n1134 = Number To Fractional String(number=w2087) -> (F-format string=w2082:string)  [unwired: 3 in]
                        n1135 = Divide(x=w2081, y=3) -> (x/y=w2084:dbl)
                        n1136 = To Word Integer(number=w2084) -> (16bit integer=w2083:i16)
                        n1137 = Replace Array Subset(array=w2085, new element=w2082, index (row)=w2083, index (col)=1) -> (w2080:string[][])
                      }
                      frame True {
                        n1138 = local read "New: VT-Sat"() -> (w2095:dbl)
                        n1139 = Search 1D Array(1D array=w2091, element="Threshold V (V):") -> (index of element=w2090:i32)  [unwired: 1 in]
                        n1140 = Divide(x=w2090, y=3) -> (x/y=w2098:dbl)
                        n1141 = To Word Integer(number=w2098) -> (16bit integer=w2089:i16)
                        n1142 = Format Value(format string="%#g", value (0)=w2095) -> (output string=w2101:string)  [unwired: 1 in]
                        n1143 = Build Array(w2092, w2101) -> (w2097:string[])
                        n1144 = Replace Array Subset(array=w2094, new element=w2097, index (row)=w2089) -> (w2093:string[][])  [unwired: 1 in]
                      }
                    }
                    n1145 = local write "Save1 Array"(w2076) -> ()
                  }
                  frame #10 {
                    n1146 = local read "Save1 Array"() -> (w2102:string[][])
                    n1147 = Array Size(array=w2102) -> (size(s)=w2108:i32[])
                    n1148 = Array Subset(array=w2102, index (row)=0, index (col)=0, length (col)=3) -> (w2104:string[][])  [unwired: 1 in]
                    n1149 = Index Array(array=w2108, index=0) -> (element=w2110:i32)
                    n1150 = Reshape Array(w2104, w2110) -> (w2103:string[])
                    n1151 = Search 1D Array(1D array=w2103, element="VT-Lin (V):") -> (index of element=w2113:i32)  [unwired: 1 in]
                    n1152 = Equal?(x=w2113, y=-1) -> (x = y?=w2112:bool)
                    n1153 = case shown="False" w2112 {
                      tunnel: w2102 -> [w2123 w2126]
                      tunnel: w2113 -> [w2120 _]
                      tunnel: [w2119 w2126] -> w2111
                      frame False {
                        n1154 = local read "New: VT-Lin"() -> (w2117:dbl)
                        n1155 = Divide(x=w2120, y=3) -> (x/y=w2122:dbl)
                        n1156 = Format Value(format string="%#g", value (0)=w2117) -> (output string=w2116:string)  [unwired: 1 in]
                        n1157 = To Word Integer(number=w2122) -> (16bit integer=w2121:i16)
                        n1158 = Replace Array Subset(array=w2123, new element=w2116, index (row)=w2121, index (col)=1) -> (w2119:string[][])
                      }
                      frame True {
                      }
                    }
                    n1159 = local write "Save1 Array"(w2111) -> ()
                  }
                  frame #11 {
                    w2127 = "STS-Sat (V/decade):"
                    n1160 = local read "Save1 Array"() -> (w2129:string[][])
                    n1161 = Array Size(array=w2129) -> (size(s)=w2134:i32[])
                    n1162 = Array Subset(array=w2129, index (row)=0, index (col)=0, length (col)=3) -> (w2130:string[][])  [unwired: 1 in]
                    n1163 = Index Array(array=w2134, index=0) -> (element=w2136:i32)
                    n1164 = Reshape Array(w2130, w2136) -> (w2128:string[])
                    n1165 = Search 1D Array(1D array=w2128, element=w2127) -> (index of element=w2139:i32)  [unwired: 1 in]
                    n1166 = Equal?(x=w2139, y=-1) -> (x = y?=w2138:bool)
                    n1167 = case shown="True" w2138 {
                      tunnel: w2129 -> [w2148 w2154]
                      tunnel: w2139 -> [w2145 _]
                      tunnel: [w2144 w2155] -> w2137
                      tunnel: w2128 -> [_ w2153]
                      tunnel: w2127 -> [_ w2152]
                      frame False {
                        n1168 = local read "New: STS"() -> (w2142:dbl)
                        n1169 = Divide(x=w2145, y=3) -> (x/y=w2147:dbl)
                        n1170 = Format Value(format string="%#g", value (0)=w2142) -> (output string=w2141:string)  [unwired: 1 in]
                        n1171 = To Word Integer(number=w2147) -> (16bit integer=w2146:i16)
                        n1172 = Replace Array Subset(array=w2148, new element=w2141, index (row)=w2146, index (col)=1) -> (w2144:string[][])
                      }
                      frame True {
                        n1173 = local read "New: STS"() -> (w2156:dbl)
                        n1174 = Search 1D Array(1D array=w2153, element="S.T.S. (V/decade):") -> (index of element=w2159:i32)  [unwired: 1 in]
                        n1175 = Divide(x=w2159, y=3) -> (x/y=w2160:dbl)
                        n1176 = To Word Integer(number=w2160) -> (16bit integer=w2151:i16)
                        n1177 = Format Value(format string="%#g", value (0)=w2156) -> (output string=w2163:string)  [unwired: 1 in]
                        n1178 = Build Array(w2152, w2163) -> (w2158:string[])
                        n1179 = Replace Array Subset(array=w2154, new element=w2158, index (row)=w2151) -> (w2155:string[][])  [unwired: 1 in]
                      }
                    }
                    n1180 = local write "Save1 Array"(w2137) -> ()
                  }
                  frame #12 {
                    w2164 = "Trap Density-VT (Traps/Vcm^2):"
                    n1181 = local read "Save1 Array"() -> (w2166:string[][])
                    n1182 = Array Size(array=w2166) -> (size(s)=w2171:i32[])
                    n1183 = Array Subset(array=w2166, index (row)=0, index (col)=0, length (col)=3) -> (w2167:string[][])  [unwired: 1 in]
                    n1184 = Index Array(array=w2171, index=0) -> (element=w2173:i32)
                    n1185 = Reshape Array(w2167, w2173) -> (w2165:string[])
                    n1186 = Search 1D Array(1D array=w2165, element=w2164) -> (index of element=w2176:i32)  [unwired: 1 in]
                    n1187 = Equal?(x=w2176, y=-1) -> (x = y?=w2175:bool)
                    n1188 = case shown="True" w2175 {
                      tunnel: w2166 -> [w2185 w2190]
                      tunnel: w2176 -> [w2181 _]
                      tunnel: [w2180 w2191] -> w2174
                      tunnel: w2165 -> [_ w2189]
                      tunnel: w2164 -> [_ w2188]
                      frame False {
                        n1189 = local read "New: Trap Density-VT"() -> (w2179:dbl)
                        n1190 = Format Value(format string="%#g", value (0)=w2179) -> (output string=w2182:string)  [unwired: 1 in]
                        n1191 = Divide(x=w2181, y=3) -> (x/y=w2184:dbl)
                        n1192 = To Word Integer(number=w2184) -> (16bit integer=w2183:i16)
                        n1193 = Replace Array Subset(array=w2185, new element=w2182, index (row)=w2183, index (col)=1) -> (w2180:string[][])
                      }
                      frame True {
                        n1194 = local read "New: Trap Density-VT"() -> (w2201:dbl)
                        n1195 = Search 1D Array(1D array=w2189, element="STS-Sat (V/decade):") -> (index of element=w2196:i32)  [unwired: 1 in]
                        n1196 = Divide(x=w2196, y=3) -> (x/y=w2195:dbl)
                        n1197 = To Word Integer(number=w2195) -> (16bit integer=w2197:i16)
                        n1198 = Format Value(format string="%#g", value (0)=w2201) -> (output string=w2192:string)  [unwired: 1 in]
                        n1199 = Build Array(w2188, w2192) -> (w2199:string[])
                        n1200 = Increment(x=w2197) -> (x+1=w2198:i16)
                        n1201 = Insert Into Array(array=w2190, index (row)=w2198, new element=w2199) -> (w2191:string[][])  [unwired: 1 in]
                      }
                    }
                    n1202 = local write "Save1 Array"(w2174) -> ()
                  }
                  frame #13 {
                    w2202 = "Trap Density-STS (Traps/Vcm^2):"
                    n1203 = local read "Save1 Array"() -> (w2204:string[][])
                    n1204 = Array Size(array=w2204) -> (size(s)=w2209:i32[])
                    n1205 = Array Subset(array=w2204, index (row)=0, index (col)=0, length (col)=3) -> (w2205:string[][])  [unwired: 1 in]
                    n1206 = Index Array(array=w2209, index=0) -> (element=w2211:i32)
                    n1207 = Reshape Array(w2205, w2211) -> (w2203:string[])
                    n1208 = Search 1D Array(1D array=w2203, element=w2202) -> (index of element=w2214:i32)  [unwired: 1 in]
                    n1209 = Equal?(x=w2214, y=-1) -> (x = y?=w2213:bool)
                    n1210 = case shown="True" w2213 {
                      tunnel: w2204 -> [w2223 w2228]
                      tunnel: w2214 -> [w2220 _]
                      tunnel: [w2219 w2229] -> w2212
                      tunnel: w2203 -> [_ w2227]
                      tunnel: w2202 -> [_ w2226]
                      frame False {
                        n1211 = local read "New: Trap Density-STS"() -> (w2217:dbl)
                        n1212 = Divide(x=w2220, y=3) -> (x/y=w2222:dbl)
                        n1213 = To Word Integer(number=w2222) -> (16bit integer=w2221:i16)
                        n1214 = Format Value(format string="%#g", value (0)=w2217) -> (output string=w2216:string)  [unwired: 1 in]
                        n1215 = Replace Array Subset(array=w2223, new element=w2216, index (row)=w2221, index (col)=1) -> (w2219:string[][])
                      }
                      frame True {
                        n1216 = local read "New: Trap Density-STS"() -> (w2230:dbl)
                        n1217 = Search 1D Array(1D array=w2227, element="Trap Density-VT (Traps/Vcm^2):") -> (index of element=w2235:i32)  [unwired: 1 in]
                        n1218 = Divide(x=w2235, y=3) -> (x/y=w2236:dbl)
                        n1219 = To Word Integer(number=w2236) -> (16bit integer=w2234:i16)
                        n1220 = Format Value(format string="%#g", value (0)=w2230) -> (output string=w2239:string)  [unwired: 1 in]
                        n1221 = Build Array(w2226, w2239) -> (w2232:string[])
                        n1222 = Increment(x=w2234) -> (x+1=w2233:i16)
                        n1223 = Insert Into Array(array=w2228, index (row)=w2233, new element=w2232) -> (w2229:string[][])  [unwired: 1 in]
                      }
                    }
                    n1224 = local write "Save1 Array"(w2212) -> ()
                  }
                }
                n1225 = Concatenate Strings(w1777, "\\", w1775) -> (w1776:string)
                n1226 = String To Path(string=w1776) -> (path=w1766:path)
                n1227 = disable-structure shown="Disabled" {
                  frame Disabled {
                  }
                  frame Enabled {
                  }
                }
              }
              frame #2 {
                n1228 = Equal?(x=w2298, y=w2295) -> (x = y?=w2297:bool)
                n1229 = case shown="False" w2297 {
                  tunnel: w2298 -> [w2301 _]
                  tunnel: w2295 -> [w2300 _]
                  frame False {
                    n1230 = Move(source path=w2301, 9:TRUE, 10:w2300) -> ()  [unwired: 2 in, 3 out]
                  }
                  frame True {
                  }
                }
              }
              frame #3 {
                n1231 = local write "Transfer File"(w2302) -> ()
                n1232 = call-poly <vilib>:"Write To Spreadsheet File.vi"("2D data"=w2303, "file path (dialog if empty)"=w2302) -> ()  [unwired: 6 in, 1 out]
              }
            }
          }
          event "Save Changes? 2": Mouse Down {
            n1233 = event-data() -> ()  [unwired: 1 in, 5 out]
            n1234 = stacked-sequence {
              seq-local: [w2361 _ _ _ _] -> [_ w2844 _ _ _]
              seq-local: [w2360 _ _ _ _] -> [_ w2845 _ _ _]
              seq-local: [w2360 _ _ _ _] -> [_ w2843 _ _ _]
              seq-local: [w2362 _ _ _ _] -> [_ w2841 _ _ _]
              seq-local: [_ w2845 _ _ _] -> [_ _ w2850 _ _]
              seq-local: [_ w2841 _ _ _] -> [_ _ w2849 _ _]
              frame #0 {
                n1235 = local read "Transfer File"() -> (w2361:path)
                n1236 = local read "New: Temp"() -> (w2364:dbl)
                n1237 = local read "New: Length"() -> (w2367:dbl)
                n1238 = local read "New: Width"() -> (w2365:dbl)
                n1239 = To Word Integer(number=w2364) -> (16bit integer=w2363:i16)
                n1240 = Number To Decimal String(number=w2363) -> (decimal integer string=w2371:string)  [unwired: 1 in]
                n1241 = To Single Precision Float(number=w2365) -> (single precision float=w2366:sgl)
                n1242 = To Single Precision Float(number=w2367) -> (single precision float=w2368:sgl)
                n1243 = local read "Index"() -> (w2375:string)
                n1244 = Strip Path(path=w2361) -> (stripped path=w2380:path)  [unwired: 1 out]
                n1245 = Number To Decimal String(number=w2368) -> (decimal integer string=w2373:string)  [unwired: 1 in]
                n1246 = Number To Decimal String(number=w2366) -> (decimal integer string=w2374:string)  [unwired: 1 in]
                n1247 = Concatenate Strings("_", w2371, "K") -> (w2369:string)
                n1248 = call "Build Text2"("Temp"=w2369, "Index"=w2375, "Length"=w2373, "Width"=w2374) -> ("Result"=w2376:string)  [unwired: 10 in, 1 out]
                n1249 = Path To String(path=w2380) -> (string=w2378:string)
                n1250 = Concatenate Strings(w2378, "\\", w2376) -> (w2377:string)
                n1251 = stacked-sequence {
                  tunnel: [_ _ _ _ _ _ _ _ _ _ _ _ _ w2803] -> _
                  tunnel: w2361 -> [w2382 _ _ _ _ _ _ _ _ _ _ _ _ _]
                  tunnel: [_ _ _ _ _ _ _ _ _ _ _ _ _ w2803] -> w2362
                  frame #0 {
                    n1252 = call-poly <vilib>:"Read From Spreadsheet File.vi"("file path (dialog if empty)"=w2382) -> ("all rows"=w2381:string[][])  [unwired: 6 in, 4 out]
                    n1253 = Array Size(array=w2381) -> (size(s)=w2386:i32[])
                    n1254 = Array Subset(array=w2381, index (row)=0, index (col)=0, length (col)=3) -> (w2390:string[][])  [unwired: 1 in]
                    n1255 = Index Array(array=w2386, index=0) -> (element=w2384:i32)
                    n1256 = Reshape Array(w2390, w2384) -> (w2383:string[])
                    n1257 = Search 1D Array(1D array=w2383, element="Dielectric (nm):") -> (index of element=w2393:i32)  [unwired: 1 in]
                    n1258 = Equal?(x=w2393, y=-1) -> (x = y?=w2392:bool)
                    n1259 = case shown="False" w2392 {
                      tunnel: w2381 -> [w2401 w2405]
                      tunnel: w2393 -> [w2397 _]
                      tunnel: [w2396 w2405] -> w2391
                      frame False {
                        n1260 = local read "New: Dielectric"() -> (w2403:dbl)
                        n1261 = Number To Fractional String(number=w2403) -> (F-format string=w2398:string)  [unwired: 3 in]
                        n1262 = Divide(x=w2397, y=3) -> (x/y=w2400:dbl)
                        n1263 = To Word Integer(number=w2400) -> (16bit integer=w2399:i16)
                        n1264 = Replace Array Subset(array=w2401, new element=w2398, index (row)=w2399, index (col)=1) -> (w2396:string[][])
                      }
                      frame True {
                      }
                    }
                    n1265 = local write "Save1 Array"(w2391) -> ()
                  }
                  frame #1 {
                    n1266 = local read "Save1 Array"() -> (w2407:string[][])
                    n1267 = Array Size(array=w2407) -> (size(s)=w2410:i32[])
                    n1268 = Array Subset(array=w2407, index (row)=0, index (col)=0, length (col)=3) -> (w2414:string[][])  [unwired: 1 in]
                    n1269 = Index Array(array=w2410, index=0) -> (element=w2408:i32)
                    n1270 = Reshape Array(w2414, w2408) -> (w2406:string[])
                    n1271 = Search 1D Array(1D array=w2406, element="Comments:") -> (index of element=w2417:i32)  [unwired: 1 in]
                    n1272 = Equal?(x=w2417, y=-1) -> (x = y?=w2416:bool)
                    n1273 = case shown="False" w2416 {
                      tunnel: w2407 -> [w2425 w2428]
                      tunnel: w2417 -> [w2422 _]
                      tunnel: [w2421 w2428] -> w2415
                      frame False {
                        n1274 = local read "Comments:"() -> (w2420:string)
                        n1275 = Divide(x=w2422, y=3) -> (x/y=w2424:dbl)
                        n1276 = To Word Integer(number=w2424) -> (16bit integer=w2423:i16)
                        n1277 = Replace Array Subset(array=w2425, new element=w2420, index (row)=w2423, index (col)=1) -> (w2421:string[][])
                      }
                      frame True {
                      }
                    }
                    n1278 = local write "Save1 Array"(w2415) -> ()
                  }
                  frame #2 {
                    n1279 = local read "Save1 Array"() -> (w2430:string[][])
                    n1280 = Array Size(array=w2430) -> (size(s)=w2433:i32[])
                    n1281 = Array Subset(array=w2430, index (row)=0, index (col)=0, length (col)=3) -> (w2437:string[][])  [unwired: 1 in]
                    n1282 = Index Array(array=w2433, index=0) -> (element=w2431:i32)
                    n1283 = Reshape Array(w2437, w2431) -> (w2429:string[])
                    n1284 = Search 1D Array(1D array=w2429, element="Length (um):") -> (index of element=w2440:i32)  [unwired: 1 in]
                    n1285 = Equal?(x=w2440, y=-1) -> (x = y?=w2439:bool)
                    n1286 = case shown="False" w2439 {
                      tunnel: w2430 -> [w2450 w2453]
                      tunnel: w2440 -> [w2447 _]
                      tunnel: [w2446 w2453] -> w2438
                      frame False {
                        n1287 = local read "New: Length"() -> (w2443:dbl)
                        n1288 = Divide(x=w2447, y=3) -> (x/y=w2449:dbl)
                        n1289 = Format Value(format string="%#g", value (0)=w2443) -> (output string=w2444:string)  [unwired: 1 in]
                        n1290 = To Word Integer(number=w2449) -> (16bit integer=w2448:i16)
                        n1291 = Replace Array Subset(array=w2450, new element=w2444, index (row)=w2448, index (col)=1) -> (w2446:string[][])
                      }
                      frame True {
                      }
                    }
                    n1292 = local write "Save1 Array"(w2438) -> ()
                  }
                  frame #3 {
                    n1293 = local read "Save1 Array"() -> (w2455:string[][])
                    n1294 = Array Size(array=w2455) -> (size(s)=w2460:i32[])
                    n1295 = Array Subset(array=w2455, index (row)=0, index (col)=0, length (col)=3) -> (w2456:string[][])  [unwired: 1 in]
                    n1296 = Index Array(array=w2460, index=0) -> (element=w2462:i32)
                    n1297 = Reshape Array(w2456, w2462) -> (w2454:string[])
                    n1298 = Search 1D Array(1D array=w2454, element="Width (um):") -> (index of element=w2465:i32)  [unwired: 1 in]
                    n1299 = Equal?(x=w2465, y=-1) -> (x = y?=w2464:bool)
                    n1300 = case shown="False" w2464 {
                      tunnel: w2465 -> [w2473 _]
                      tunnel: w2455 -> [w2472 w2478]
                      tunnel: [w2471 w2478] -> w2463
                      frame False {
                        n1301 = local read "New: Width"() -> (w2468:dbl)
                        n1302 = Divide(x=w2473, y=3) -> (x/y=w2475:dbl)
                        n1303 = To Word Integer(number=w2475) -> (16bit integer=w2474:i16)
                        n1304 = Format Value(format string="%#g", value (0)=w2468) -> (output string=w2469:string)  [unwired: 1 in]
                        n1305 = Replace Array Subset(array=w2472, new element=w2469, index (row)=w2474, index (col)=1) -> (w2471:string[][])
                      }
                      frame True {
                      }
                    }
                    n1306 = local write "Save1 Array"(w2463) -> ()
                  }
                  frame #4 {
                    w2488 = "Sample Temp (K):"
                    n1307 = local read "Save1 Array"() -> (w2480:string[][])
                    n1308 = Array Size(array=w2480) -> (size(s)=w2485:i32[])
                    n1309 = Array Subset(array=w2480, index (row)=0, index (col)=0, length (col)=3) -> (w2481:string[][])  [unwired: 1 in]
                    n1310 = Index Array(array=w2485, index=0) -> (element=w2487:i32)
                    n1311 = Reshape Array(w2481, w2487) -> (w2479:string[])
                    n1312 = Search 1D Array(1D array=w2479, element=w2488) -> (index of element=w2491:i32)  [unwired: 1 in]
                    n1313 = Equal?(x=w2491, y=-1) -> (x = y?=w2490:bool)
                    n1314 = case shown="True" w2490 {
                      tunnel: w2480 -> [w2500 w2514]
                      tunnel: w2491 -> [w2497 _]
                      tunnel: [w2496 w2513] -> w2489
                      tunnel: w2479 -> [_ w2516]
                      tunnel: w2488 -> [_ w2503]
                      frame False {
                        n1315 = local read "New: Temp"() -> (w2494:dbl)
                        n1316 = Divide(x=w2497, y=3) -> (x/y=w2499:dbl)
                        n1317 = Format Value(format string="%#g", value (0)=w2494) -> (output string=w2493:string)  [unwired: 1 in]
                        n1318 = To Word Integer(number=w2499) -> (16bit integer=w2498:i16)
                        n1319 = Replace Array Subset(array=w2500, new element=w2493, index (row)=w2498, index (col)=1) -> (w2496:string[][])
                      }
                      frame True {
                        n1320 = local read "New: Temp"() -> (w2505:dbl)
                        n1321 = Search 1D Array(1D array=w2516, element="Width (um):") -> (index of element=w2510:i32)  [unwired: 1 in]
                        n1322 = Divide(x=w2510, y=3) -> (x/y=w2511:dbl)
                        n1323 = To Word Integer(number=w2511) -> (16bit integer=w2509:i16)
                        n1324 = Format Value(format string="%#g", value (0)=w2505) -> (output string=w2504:string)  [unwired: 1 in]
                        n1325 = Build Array(w2503, w2504) -> (w2507:string[])
                        n1326 = Increment(x=w2509) -> (x+1=w2508:i16)
                        n1327 = Insert Into Array(array=w2514, index (row)=w2508, new element=w2507) -> (w2513:string[][])  [unwired: 1 in]
                      }
                    }
                    n1328 = local write "Save1 Array"(w2489) -> ()
                  }
                  frame #5 {
                    w2526 = "Mobility-Sat (cm^2/Vs):"
                    n1329 = local read "Save1 Array"() -> (w2518:string[][])
                    n1330 = Array Size(array=w2518) -> (size(s)=w2523:i32[])
                    n1331 = Array Subset(array=w2518, index (row)=0, index (col)=0, length (col)=3) -> (w2519:string[][])  [unwired: 1 in]
                    n1332 = Index Array(array=w2523, index=0) -> (element=w2525:i32)
                    n1333 = Reshape Array(w2519, w2525) -> (w2517:string[])
                    n1334 = Search 1D Array(1D array=w2517, element=w2526) -> (index of element=w2529:i32)  [unwired: 1 in]
                    n1335 = Equal?(x=w2529, y=-1) -> (x = y?=w2528:bool)
                    n1336 = case shown="True" w2528 {
                      tunnel: w2518 -> [w2538 w2546]
                      tunnel: w2529 -> [w2535 _]
                      tunnel: [w2534 w2545] -> w2527
                      tunnel: w2517 -> [_ w2543]
                      tunnel: w2526 -> [_ w2541]
                      frame False {
                        n1337 = local read "New: Mobility-Sat"() -> (w2531:dbl)
                        n1338 = Divide(x=w2535, y=3) -> (x/y=w2537:dbl)
                        n1339 = To Word Integer(number=w2537) -> (16bit integer=w2536:i16)
                        n1340 = Format Value(format string="%#g", value (0)=w2531) -> (output string=w2532:string)  [unwired: 1 in]
                        n1341 = Replace Array Subset(array=w2538, new element=w2532, index (row)=w2536, index (col)=1) -> (w2534:string[][])
                      }
                      frame True {
                        n1342 = local read "New: Mobility-Sat"() -> (w2547:dbl)
                        n1343 = Search 1D Array(1D array=w2543, element="Mobility (cm^2/Vs):") -> (index of element=w2550:i32)  [unwired: 1 in]
                        n1344 = Divide(x=w2550, y=3) -> (x/y=w2551:dbl)
                        n1345 = To Word Integer(number=w2551) -> (16bit integer=w2542:i16)
                        n1346 = Format Value(format string="%#g", value (0)=w2547) -> (output string=w2544:string)  [unwired: 1 in]
                        n1347 = Build Array(w2541, w2544) -> (w2549:string[])
                        n1348 = Replace Array Subset(array=w2546, new element=w2549, index (row)=w2542) -> (w2545:string[][])  [unwired: 1 in]
                      }
                    }
                    n1349 = local write "Save1 Array"(w2527) -> ()
                  }
                  frame #6 {
                    w2563 = "Mobility-Lin (cm^2/Vs):"
                    n1350 = local read "Save1 Array"() -> (w2554:string[][])
                    n1351 = Array Size(array=w2554) -> (size(s)=w2560:i32[])
                    n1352 = Array Subset(array=w2554, index (row)=0, index (col)=0, length (col)=3) -> (w2556:string[][])  [unwired: 1 in]
                    n1353 = Index Array(array=w2560, index=0) -> (element=w2562:i32)
                    n1354 = Reshape Array(w2556, w2562) -> (w2555:string[])
                    n1355 = Search 1D Array(1D array=w2555, element=w2563) -> (index of element=w2566:i32)  [unwired: 1 in]
                    n1356 = Equal?(x=w2566, y=-1) -> (x = y?=w2565:bool)
                    n1357 = case shown="True" w2565 {
                      tunnel: w2554 -> [w2575 w2581]
                      tunnel: w2566 -> [w2572 _]
                      tunnel: [w2571 w2580] -> w2564
                      tunnel: w2555 -> [_ w2579]
                      tunnel: w2563 -> [_ w2578]
                      frame False {
                        n1358 = local read "Calc: Mobility-Lin"() -> (w2568:dbl)
                        n1359 = Divide(x=w2572, y=3) -> (x/y=w2574:dbl)
                        n1360 = To Word Integer(number=w2574) -> (16bit integer=w2573:i16)
                        n1361 = Format Value(format string="%#g", value (0)=w2568) -> (output string=w2569:string)  [unwired: 1 in]
                        n1362 = Replace Array Subset(array=w2575, new element=w2569, index (row)=w2573, index (col)=1) -> (w2571:string[][])
                      }
                      frame True {
                        n1363 = local read "Calc: Mobility-Lin"() -> (w2582:dbl)
                        n1364 = Search 1D Array(1D array=w2579, element="Mobility-Sat (cm^2/Vs):") -> (index of element=w2587:i32)  [unwired: 1 in]
                        n1365 = Divide(x=w2587, y=3) -> (x/y=w2588:dbl)
                        n1366 = To Word Integer(number=w2588) -> (16bit integer=w2586:i16)
                        n1367 = Format Value(format string="%#g", value (0)=w2582) -> (output string=w2591:string)  [unwired: 1 in]
                        n1368 = Build Array(w2578, w2591) -> (w2584:string[])
                        n1369 = Increment(x=w2586) -> (x+1=w2585:i16)
                        n1370 = Insert Into Array(array=w2581, index (row)=w2585, new element=w2584) -> (w2580:string[][])  [unwired: 1 in]
                      }
                    }
                    n1371 = local write "Save1 Array"(w2564) -> ()
                  }
                  frame #7 {
                    w2601 = "On/Off I-Sat:"
                    n1372 = local read "Save1 Array"() -> (w2592:string[][])
                    n1373 = Array Size(array=w2592) -> (size(s)=w2598:i32[])
                    n1374 = Array Subset(array=w2592, index (row)=0, index (col)=0, length (col)=3) -> (w2594:string[][])  [unwired: 1 in]
                    n1375 = Index Array(array=w2598, index=0) -> (element=w2600:i32)
                    n1376 = Reshape Array(w2594, w2600) -> (w2593:string[])
                    n1377 = Search 1D Array(1D array=w2593, element=w2601) -> (index of element=w2604:i32)  [unwired: 1 in]
                    n1378 = Equal?(x=w2604, y=-1) -> (x = y?=w2603:bool)
                    n1379 = case shown="True" w2603 {
                      tunnel: w2592 -> [w2613 w2620]
                      tunnel: w2604 -> [w2610 _]
                      tunnel: [w2609 w2621] -> w2602
                      tunnel: w2593 -> [_ w2618]
                      tunnel: w2601 -> [_ w2616]
                      frame False {
                        n1380 = local read "Calc: On/Off"() -> (w2606:dbl)
                        n1381 = Divide(x=w2610, y=3) -> (x/y=w2612:dbl)
                        n1382 = To Word Integer(number=w2612) -> (16bit integer=w2611:i16)
                        n1383 = Format Value(format string="%#g", value (0)=w2606) -> (output string=w2607:string)  [unwired: 1 in]
                        n1384 = Replace Array Subset(array=w2613, new element=w2607, index (row)=w2611, index (col)=1) -> (w2609:string[][])
                      }
                      frame True {
                        n1385 = local read "Calc: On/Off"() -> (w2622:dbl)
                        n1386 = Search 1D Array(1D array=w2618, element="On/Off Current:") -> (index of element=w2625:i32)  [unwired: 1 in]
                        n1387 = Divide(x=w2625, y=3) -> (x/y=w2626:dbl)
                        n1388 = To Word Integer(number=w2626) -> (16bit integer=w2617:i16)
                        n1389 = Format Value(format string="%#g", value (0)=w2622) -> (output string=w2619:string)  [unwired: 1 in]
                        n1390 = Build Array(w2616, w2619) -> (w2624:string[])
                        n1391 = Replace Array Subset(array=w2620, new element=w2624, index (row)=w2617) -> (w2621:string[][])  [unwired: 1 in]
                      }
                    }
                    n1392 = local write "Save1 Array"(w2602) -> ()
                  }
                  frame #8 {
                    w2638 = "Off I-Sat (A):"
                    n1393 = local read "Save1 Array"() -> (w2629:string[][])
                    n1394 = Array Size(array=w2629) -> (size(s)=w2635:i32[])
                    n1395 = Array Subset(array=w2629, index (row)=0, index (col)=0, length (col)=3) -> (w2631:string[][])  [unwired: 1 in]
                    n1396 = Index Array(array=w2635, index=0) -> (element=w2637:i32)
                    n1397 = Reshape Array(w2631, w2637) -> (w2630:string[])
                    n1398 = Search 1D Array(1D array=w2630, element=w2638) -> (index of element=w2641:i32)  [unwired: 1 in]
                    n1399 = Equal?(x=w2641, y=-1) -> (x = y?=w2640:bool)
                    n1400 = case shown="True" w2640 {
                      tunnel: w2629 -> [w2650 w2656]
                      tunnel: w2641 -> [w2647 _]
                      tunnel: [w2646 w2655] -> w2639
                      tunnel: w2630 -> [_ w2654]
                      tunnel: w2638 -> [_ w2653]
                      frame False {
                        n1401 = local read "Calc: Off I-Sat"() -> (w2645:dbl)
                        n1402 = Divide(x=w2647, y=3) -> (x/y=w2649:dbl)
                        n1403 = Format Value(format string="%#g", value (0)=w2645) -> (output string=w2643:string)  [unwired: 1 in]
                        n1404 = To Word Integer(number=w2649) -> (16bit integer=w2648:i16)
                        n1405 = Replace Array Subset(array=w2650, new element=w2643, index (row)=w2648, index (col)=1) -> (w2646:string[][])
                      }
                      frame True {
                        n1406 = local read "Calc: Off I-Sat"() -> (w2657:dbl)
                        n1407 = Search 1D Array(1D array=w2654, element="On/Off I-Sat:") -> (index of element=w2662:i32)  [unwired: 1 in]
                        n1408 = Divide(x=w2662, y=3) -> (x/y=w2663:dbl)
                        n1409 = To Word Integer(number=w2663) -> (16bit integer=w2661:i16)
                        n1410 = Format Value(format string="%#g", value (0)=w2657) -> (output string=w2666:string)  [unwired: 1 in]
                        n1411 = Build Array(w2653, w2666) -> (w2659:string[])
                        n1412 = Increment(x=w2661) -> (x+1=w2660:i16)
                        n1413 = Insert Into Array(array=w2656, index (row)=w2660, new element=w2659) -> (w2655:string[][])  [unwired: 1 in]
                      }
                    }
                    n1414 = local write "Save1 Array"(w2639) -> ()
                  }
                  frame #9 {
                    w2668 = "Vt-Sat (V):"
                    n1415 = local read "Save1 Array"() -> (w2669:string[][])
                    n1416 = Array Size(array=w2669) -> (size(s)=w2674:i32[])
                    n1417 = Array Subset(array=w2669, index (row)=0, index (col)=0, length (col)=3) -> (w2670:string[][])  [unwired: 1 in]
                    n1418 = Index Array(array=w2674, index=0) -> (element=w2676:i32)
                    n1419 = Reshape Array(w2670, w2676) -> (w2667:string[])
                    n1420 = Search 1D Array(1D array=w2667, element=w2668) -> (index of element=w2679:i32)  [unwired: 1 in]
                    n1421 = Equal?(x=w2679, y=-1) -> (x = y?=w2678:bool)
                    n1422 = case shown="True" w2678 {
                      tunnel: w2669 -> [w2686 w2695]
                      tunnel: w2679 -> [w2682 _]
                      tunnel: [w2681 w2694] -> w2677
                      tunnel: w2668 -> [_ w2693]
                      tunnel: w2667 -> [_ w2692]
                      frame False {
                        n1423 = local read "New: VT-Sat"() -> (w2688:dbl)
                        n1424 = Number To Fractional String(number=w2688) -> (F-format string=w2683:string)  [unwired: 3 in]
                        n1425 = Divide(x=w2682, y=3) -> (x/y=w2685:dbl)
                        n1426 = To Word Integer(number=w2685) -> (16bit integer=w2684:i16)
                        n1427 = Replace Array Subset(array=w2686, new element=w2683, index (row)=w2684, index (col)=1) -> (w2681:string[][])
                      }
                      frame True {
                        n1428 = local read "New: VT-Sat"() -> (w2696:dbl)
                        n1429 = Search 1D Array(1D array=w2692, element="Threshold V (V):") -> (index of element=w2691:i32)  [unwired: 1 in]
                        n1430 = Divide(x=w2691, y=3) -> (x/y=w2699:dbl)
                        n1431 = To Word Integer(number=w2699) -> (16bit integer=w2690:i16)
                        n1432 = Format Value(format string="%#g", value (0)=w2696) -> (output string=w2702:string)  [unwired: 1 in]
                        n1433 = Build Array(w2693, w2702) -> (w2698:string[])
                        n1434 = Replace Array Subset(array=w2695, new element=w2698, index (row)=w2690) -> (w2694:string[][])  [unwired: 1 in]
                      }
                    }
                    n1435 = local write "Save1 Array"(w2677) -> ()
                  }
                  frame #10 {
                    n1436 = local read "Save1 Array"() -> (w2703:string[][])
                    n1437 = Array Size(array=w2703) -> (size(s)=w2709:i32[])
                    n1438 = Array Subset(array=w2703, index (row)=0, index (col)=0, length (col)=3) -> (w2705:string[][])  [unwired: 1 in]
                    n1439 = Index Array(array=w2709, index=0) -> (element=w2711:i32)
                    n1440 = Reshape Array(w2705, w2711) -> (w2704:string[])
                    n1441 = Search 1D Array(1D array=w2704, element="VT-Lin (V):") -> (index of element=w2714:i32)  [unwired: 1 in]
                    n1442 = Equal?(x=w2714, y=-1) -> (x = y?=w2713:bool)
                    n1443 = case shown="False" w2713 {
                      tunnel: w2703 -> [w2724 w2727]
                      tunnel: w2714 -> [w2721 _]
                      tunnel: [w2720 w2727] -> w2712
                      frame False {
                        n1444 = local read "New: VT-Lin"() -> (w2718:dbl)
                        n1445 = Divide(x=w2721, y=3) -> (x/y=w2723:dbl)
                        n1446 = Format Value(format string="%#g", value (0)=w2718) -> (output string=w2717:string)  [unwired: 1 in]
                        n1447 = To Word Integer(number=w2723) -> (16bit integer=w2722:i16)
                        n1448 = Replace Array Subset(array=w2724, new element=w2717, index (row)=w2722, index (col)=1) -> (w2720:string[][])
                      }
                      frame True {
                      }
                    }
                    n1449 = local write "Save1 Array"(w2712) -> ()
                  }
                  frame #11 {
                    w2728 = "STS-Sat (V/decade):"
                    n1450 = local read "Save1 Array"() -> (w2730:string[][])
                    n1451 = Array Size(array=w2730) -> (size(s)=w2735:i32[])
                    n1452 = Array Subset(array=w2730, index (row)=0, index (col)=0, length (col)=3) -> (w2731:string[][])  [unwired: 1 in]
                    n1453 = Index Array(array=w2735, index=0) -> (element=w2737:i32)
                    n1454 = Reshape Array(w2731, w2737) -> (w2729:string[])
                    n1455 = Search 1D Array(1D array=w2729, element=w2728) -> (index of element=w2740:i32)  [unwired: 1 in]
                    n1456 = Equal?(x=w2740, y=-1) -> (x = y?=w2739:bool)
                    n1457 = case shown="True" w2739 {
                      tunnel: w2730 -> [w2749 w2755]
                      tunnel: w2740 -> [w2746 _]
                      tunnel: [w2745 w2756] -> w2738
                      tunnel: w2729 -> [_ w2754]
                      tunnel: w2728 -> [_ w2753]
                      frame False {
                        n1458 = local read "New: STS"() -> (w2743:dbl)
                        n1459 = Divide(x=w2746, y=3) -> (x/y=w2748:dbl)
                        n1460 = Format Value(format string="%#g", value (0)=w2743) -> (output string=w2742:string)  [unwired: 1 in]
                        n1461 = To Word Integer(number=w2748) -> (16bit integer=w2747:i16)
                        n1462 = Replace Array Subset(array=w2749, new element=w2742, index (row)=w2747, index (col)=1) -> (w2745:string[][])
                      }
                      frame True {
                        n1463 = local read "New: STS"() -> (w2757:dbl)
                        n1464 = Search 1D Array(1D array=w2754, element="S.T.S. (V/decade):") -> (index of element=w2760:i32)  [unwired: 1 in]
                        n1465 = Divide(x=w2760, y=3) -> (x/y=w2761:dbl)
                        n1466 = To Word Integer(number=w2761) -> (16bit integer=w2752:i16)
                        n1467 = Format Value(format string="%#g", value (0)=w2757) -> (output string=w2764:string)  [unwired: 1 in]
                        n1468 = Build Array(w2753, w2764) -> (w2759:string[])
                        n1469 = Replace Array Subset(array=w2755, new element=w2759, index (row)=w2752) -> (w2756:string[][])  [unwired: 1 in]
                      }
                    }
                    n1470 = local write "Save1 Array"(w2738) -> ()
                  }
                  frame #12 {
                    w2765 = "Trap Density-VT (Traps/Vcm^2):"
                    n1471 = local read "Save1 Array"() -> (w2767:string[][])
                    n1472 = Array Size(array=w2767) -> (size(s)=w2772:i32[])
                    n1473 = Array Subset(array=w2767, index (row)=0, index (col)=0, length (col)=3) -> (w2768:string[][])  [unwired: 1 in]
                    n1474 = Index Array(array=w2772, index=0) -> (element=w2774:i32)
                    n1475 = Reshape Array(w2768, w2774) -> (w2766:string[])
                    n1476 = Search 1D Array(1D array=w2766, element=w2765) -> (index of element=w2777:i32)  [unwired: 1 in]
                    n1477 = Equal?(x=w2777, y=-1) -> (x = y?=w2776:bool)
                    n1478 = case shown="True" w2776 {
                      tunnel: w2767 -> [w2786 w2791]
                      tunnel: w2777 -> [w2782 _]
                      tunnel: [w2781 w2792] -> w2775
                      tunnel: w2766 -> [_ w2790]
                      tunnel: w2765 -> [_ w2789]
                      frame False {
                        n1479 = local read "New: Trap Density-VT"() -> (w2780:dbl)
                        n1480 = Format Value(format string="%#g", value (0)=w2780) -> (output string=w2783:string)  [unwired: 1 in]
                        n1481 = Divide(x=w2782, y=3) -> (x/y=w2785:dbl)
                        n1482 = To Word Integer(number=w2785) -> (16bit integer=w2784:i16)
                        n1483 = Replace Array Subset(array=w2786, new element=w2783, index (row)=w2784, index (col)=1) -> (w2781:string[][])
                      }
                      frame True {
                        n1484 = local read "New: Trap Density-VT"() -> (w2802:dbl)
                        n1485 = Search 1D Array(1D array=w2790, element="STS-Sat (V/decade):") -> (index of element=w2797:i32)  [unwired: 1 in]
                        n1486 = Divide(x=w2797, y=3) -> (x/y=w2796:dbl)
                        n1487 = To Word Integer(number=w2796) -> (16bit integer=w2798:i16)
                        n1488 = Format Value(format string="%#g", value (0)=w2802) -> (output string=w2793:string)  [unwired: 1 in]
                        n1489 = Build Array(w2789, w2793) -> (w2800:string[])
                        n1490 = Increment(x=w2798) -> (x+1=w2799:i16)
                        n1491 = Insert Into Array(array=w2791, index (row)=w2799, new element=w2800) -> (w2792:string[][])  [unwired: 1 in]
                      }
                    }
                    n1492 = local write "Save1 Array"(w2775) -> ()
                  }
                  frame #13 {
                    w2804 = "Trap Density-STS (Traps/Vcm^2):"
                    n1493 = local read "Save1 Array"() -> (w2806:string[][])
                    n1494 = Array Size(array=w2806) -> (size(s)=w2811:i32[])
                    n1495 = Array Subset(array=w2806, index (row)=0, index (col)=0, length (col)=3) -> (w2807:string[][])  [unwired: 1 in]
                    n1496 = Index Array(array=w2811, index=0) -> (element=w2813:i32)
                    n1497 = Reshape Array(w2807, w2813) -> (w2805:string[])
                    n1498 = Search 1D Array(1D array=w2805, element=w2804) -> (index of element=w2815:i32)  [unwired: 1 in]
                    n1499 = Equal?(x=w2815, y=-1) -> (x = y?=w2814:bool)
                    n1500 = case shown="True" w2814 {
                      tunnel: w2806 -> [w2824 w2829]
                      tunnel: w2815 -> [w2821 _]
                      tunnel: [w2820 w2830] -> w2803
                      tunnel: w2805 -> [_ w2828]
                      tunnel: w2804 -> [_ w2827]
                      frame False {
                        n1501 = local read "New: Trap Density-STS"() -> (w2818:dbl)
                        n1502 = Divide(x=w2821, y=3) -> (x/y=w2823:dbl)
                        n1503 = To Word Integer(number=w2823) -> (16bit integer=w2822:i16)
                        n1504 = Format Value(format string="%#g", value (0)=w2818) -> (output string=w2817:string)  [unwired: 1 in]
                        n1505 = Replace Array Subset(array=w2824, new element=w2817, index (row)=w2822, index (col)=1) -> (w2820:string[][])
                      }
                      frame True {
                        n1506 = local read "New: Trap Density-STS"() -> (w2831:dbl)
                        n1507 = Search 1D Array(1D array=w2828, element="Trap Density-VT (Traps/Vcm^2):") -> (index of element=w2836:i32)  [unwired: 1 in]
                        n1508 = Divide(x=w2836, y=3) -> (x/y=w2837:dbl)
                        n1509 = To Word Integer(number=w2837) -> (16bit integer=w2835:i16)
                        n1510 = Format Value(format string="%#g", value (0)=w2831) -> (output string=w2840:string)  [unwired: 1 in]
                        n1511 = Build Array(w2827, w2840) -> (w2833:string[])
                        n1512 = Increment(x=w2835) -> (x+1=w2834:i16)
                        n1513 = Insert Into Array(array=w2829, index (row)=w2834, new element=w2833) -> (w2830:string[][])  [unwired: 1 in]
                      }
                    }
                    n1514 = local write "Save1 Array"(w2803) -> ()
                  }
                }
                n1515 = String To Path(string=w2377) -> (path=w2360:path)
                "No Image 2" <- w2360
              }
              frame #1 {
                n1516 = Equal?(x=w2844, y=w2843) -> (x = y?=w2842:bool)
                n1517 = case shown="False" w2842 {
                  tunnel: w2844 -> [w2848 _]
                  tunnel: w2843 -> [w2847 _]
                  frame False {
                    n1518 = Move(source path=w2848, 9:TRUE, 10:w2847) -> ()  [unwired: 2 in, 3 out]
                  }
                  frame True {
                  }
                }
              }
              frame #2 {
                n1519 = local write "Transfer File"(w2850) -> ()
                n1520 = call-poly <vilib>:"Write To Spreadsheet File.vi"("2D data"=w2849, "file path (dialog if empty)"=w2850) -> ()  [unwired: 6 in, 1 out]
              }
              frame #3 {
                w2951 = 0
                # "Moves to next file and displays new image/data"
                n1521 = property on="Image Out" class="ImageControl"() -> (error out=w2913:errorcluster, "Image Center Position"=w2917:cluster{"X":u32, "Y":u32})  [unwired: 2 in, 1 out]
                n1522 = local read "Transfer File"() -> (w2956:path)
                n1523 = Strip Path(path=w2956) -> (stripped path=w2947:path, name=w2965:string)
                n1524 = Unbundle(w2917) -> ("X"=w2915:u32)  [unwired: 1 out]
                n1525 = local write "Transfer Folder"(w2947) -> ()
                n1526 = Bundle("X"=w2915, 0) -> (w2916:cluster{"X":u32, i32})  [unwired: 1 in]
                n1527 = property on="Image Out" class="ImageControl"(error in=w2913, "Image Center Position"=w2916) -> ()  [unwired: 1 in, 2 out]
                n1528 = List Folder(path=w2947) -> (filenames=w2961:string[])  [unwired: 3 in, 3 out]
                n1529 = Search 1D Array(1D array=w2961, element=w2965) -> (index of element=w2958:i32)  [unwired: 1 in]
                n1530 = Array Size(array=w2961) -> (size(s)=w2957:i32)
                n1531 = Decrement(x=w2957) -> (x-1=w2959:i32)
                n1532 = Equal?(x=w2958, y=w2959) -> (x = y?=w2960:bool)
                n1533 = local read "Folder Index"() -> (w2909:dbl)
                n1534 = case shown="False" w2960 {
                  tunnel: w2909 -> [w3090 _]
                  tunnel: [w3089 0] -> w2908
                  frame False {
                    n1535 = Increment(x=w3090) -> (x+1=w3089:dbl)
                  }
                  frame True {
                  }
                }
                n1536 = invoke on="Image Out" class="ImageControl" method="Clear ROI"() -> ()  [unwired: 3 in, 3 out]
                n1537 = local write "Folder Index"(w2908) -> ()
                n1538 = Path To String(path=w2947) -> (string=w2966:string)
                n1539 = Index Array(array=w2961, index=w2908) -> (element=w2962:string)
                n1540 = local write "Data Name:"(w2962) -> ()
                n1541 = Concatenate Strings(w2966, "\\", w2962) -> (w2964:string)
                n1542 = String To Path(string=w2964) -> (path=w2862:path)
                n1543 = call "Recorded Values.vi"("Path"=w2862) -> ("Recorded Char"=w2864:T5, "Recorded Prop"=w2865:T6, "Fabrication Prop"=w2863:T7)  [unwired: 8 in]
                n1544 = Unbundle By Name(w2864) -> ("Mobility-Sat"=w2877:dbl, "Moblitity-Lin"=w2878:dbl, "On/Off"=w2879:dbl, "Off Current"=w2880:dbl, "Vt-Sat"=w2856:dbl, "STS"=w2881:dbl, "Trap Density-VT"=w2882:dbl, "Trap Density-STS"=w2883:dbl)
                n1545 = Unbundle By Name(w2865) -> ("Date Recorded"=w2873:string, "Index"=w2874:string, "Length"=w2875:dbl, "Width"=w2876:dbl, "Sample Temp"=w2859:dbl)
                n1546 = Unbundle By Name(w2863) -> ("Date Created"=w2884:string, "Material"=w2866:string, "Solvent"=w2867:string, "Concentration"=w2868:dbl, "Method"=w2869:string, "Dielectric (nm)"=w2870:dbl, "Treatment"=w2871:string, "Comments"=w2872:string)
                n1547 = local write "Rec: Off I-Sat"(w2880) -> ()
                n1548 = local write "Rec: Comments"(w2872) -> ()
                n1549 = local write "Rec: VT-Sat"(w2856) -> ()
                n1550 = local write "Date Created"(w2884) -> ()
                n1551 = local write "Rec: Material"(w2866) -> ()
                n1552 = local write "Rec: Solvent"(w2867) -> ()
                n1553 = local write "Rec: Concentration"(w2868) -> ()
                n1554 = local write "Rec: Method"(w2869) -> ()
                n1555 = local write "Rec: Dielectric (d)"(w2870) -> ()
                n1556 = local write "Surface Treatment:"(w2871) -> ()
                n1557 = local write "Index"(w2874) -> ()
                n1558 = local write "Rec: Mobility-Sat"(w2877) -> ()
                n1559 = local write "Rec: Mobility-Lin"(w2878) -> ()
                n1560 = local write "Rec: On/Off"(w2879) -> ()
                n1561 = local write "Rec: STS"(w2881) -> ()
                n1562 = local write "Rec: Trap Density-VT"(w2882) -> ()
                n1563 = local write "Rec: Trap Density-STS"(w2883) -> ()
                n1564 = local write "Date Recorded"(w2873) -> ()
                n1565 = local write "Rec: Length"(w2875) -> ()
                n1566 = local write "Rec: Width"(w2876) -> ()
                n1567 = local write "Rec: Temp"(w2859) -> ()
                n1568 = Equal To 0?(x=w2859) -> (x = 0?=w2860:bool)
                n1569 = case shown="False" w2860 {
                  tunnel: [w2967 w2968] -> w2857
                  tunnel: w2859 -> [w2967 _]
                  frame False {
                  }
                  frame True {
                    n1570 = local read "Room Temp"() -> (w2968:dbl)
                  }
                }
                n1571 = local read "NumPoints Log"() -> (w2905:dbl)
                n1572 = local write "Transfer File"(w2862) -> ()
                n1573 = local read "Num Pts"() -> (w2894:dbl)
                n1574 = local read "Num Pts"() -> (w2906:dbl)
                n1575 = call-poly <vilib>:"Read From Spreadsheet File.vi"("file path (dialog if empty)"=w2862) -> ("all rows"=w2953:string[][])  [unwired: 6 in, 4 out]
                n1576 = call "Mobility-Vt Calculator-File.vi"("NumPts"=w2906, "Path"=w2862) -> ("Graph Cluster"=w2853:T8, "Output"=w2907:T9, "Index-Sat"=w2887:dbl, "Index-Lin"=w2893:dbl)  [unwired: 5 in, 1 out]
                n1577 = Unbundle By Name(w2853) -> ("Sqrt Sat"=w2852:cluster{dbl[], dbl[]}[], "Sqrt Lin"=w2851:cluster{dbl[], dbl[]}[])  [unwired: 4 out]
                n1578 = Decimate 1D Array(w2851) -> (w2901:cluster{dbl[], dbl[]}[])  [unwired: 1 out]
                n1579 = Array To Cluster(array=w2901) -> (cluster=w2899:T10)
                n1580 = Unbundle(w2899) -> ("[0]"=w2900:cluster{dbl[], dbl[]})  [unwired: 8 out]
                n1581 = Unbundle(w2900) -> (w2898:dbl[], w2897:dbl[])
                n1582 = Array Subset(array=w2897, index=w2893, length=w2894) -> (w2895:dbl[])
                n1583 = Array Subset(array=w2898, index=w2893, length=w2894) -> (w2896:dbl[])
                n1584 = call "STS Calculator-File.vi"("NumPts"=w2905, "Path"=w2862) -> ("STS Index-Sat"=w2904:dbl, "XY Graph-Sat"=w2903:cluster{dbl[], dbl[]}[], "Ouput"=w2902:cluster{"STS-Sat":dbl, "STS-Lin":dbl})  [unwired: 5 in, 2 out]
                n1585 = local read "New: Dielectric"() -> (w2889:dbl)
                n1586 = local write "Sat-Trans Slider"(w2887) -> ()
                n1587 = local write "Lin Id-Used"(w2895) -> ()
                n1588 = local write "Lin-Vg Array-Used"(w2896) -> ()
                n1589 = local write "MobVi Index"(w2887) -> ()
                n1590 = local write "Index 2"(w2904) -> ()
                n1591 = local write "Sqrt-Sat"(w2852) -> ()
                n1592 = local write "Log-Sat"(w2903) -> ()
                n1593 = Unbundle By Name(w2907) -> ("Mobility-Sat"=w2892:dbl, "Vt-Sat"=w2854:dbl, "Mobility-Lin"=w2891:dbl, "Mobility-Lin"=w2890:dbl, "Off I-Sat"=w2885:dbl, "On/Off I-Sat"=w2855:dbl)
                n1594 = local write "Sqrt-Lin"(w2851) -> ()
                n1595 = Array Size(array=w2953) -> (size(s)=w2952:i32[])
                n1596 = local write "New: Temp"(w2857) -> ()
                n1597 = Unbundle By Name(w2902) -> ("STS-Sat"=w2888:dbl)
                n1598 = call "Trap Density_STS.vi"("Temp (T) [K]"=w2857, "S.T.S. (S)"=w2888, "Dielectric"=w2889) -> ("Trap Density (N)"=w2861:dbl)  [unwired: 8 in]
                n1599 = local write "Calc: Mobility-Lin"(w2891) -> ()
                n1600 = local write "Calc: Mobility-Sat"(w2892) -> ()
                n1601 = local write "Calc: Off I-Sat"(w2885) -> ()
                n1602 = local write "Calc: VT-Sat"(w2854) -> ()
                n1603 = local write "New: VT-Lin"(w2890) -> ()
                n1604 = local write "New: Trap Density-STS"(w2861) -> ()
                n1605 = local write "Calc: Trap Density-STS"(w2861) -> ()
                n1606 = local read "Image Folder"() -> (w2941:path)
                n1607 = local read "New: Dielectric"() -> (w2886:dbl)
                n1608 = Decimate 1D Array(w2852) -> (w2936:cluster{dbl[], dbl[]}[])  [unwired: 1 out]
                n1609 = Decimate 1D Array(w2903) -> (w2926:cluster{dbl[], dbl[]}[])  [unwired: 1 out]
                n1610 = Index Array(array=w2952, index=w2951) -> (element=w2932:i32)
                n1611 = Array Subset(array=w2953, index (row)=w2951, index (col)=w2951, length (col)=3) -> (w2954:string[][])  [unwired: 1 in]
                n1612 = local write "Calc: STS"(w2888) -> ()
                n1613 = local write "New: VT-Sat"(w2854) -> ()
                n1614 = local write "New: Mobility-Sat"(w2892) -> ()
                n1615 = local write "Calc: On/Off"(w2855) -> ()
                n1616 = local write "New: Mobility-Lin"(w2891) -> ()
                n1617 = List Folder(path=w2941) -> (filenames=w2946:string[])  [unwired: 3 in, 3 out]
                n1618 = local write "New: VT-Lin"(w2890) -> ()
                n1619 = Array To Cluster(array=w2936) -> (cluster=w2938:T10)
                n1620 = Array To Cluster(array=w2926) -> (cluster=w2924:T10)
                n1621 = Reshape Array(w2954, w2932) -> (w2939:string[])
                n1622 = Subtract(x=w2932, y=20) -> (x-y=w2931:i32)
                n1623 = local write "New: STS"(w2888) -> ()
                n1624 = property on="Sat-Trans Slider" class="Slide (strict)"("Scale.Maximum"=w2931) -> ()  [unwired: 2 in, 2 out]
                n1625 = call "Trap Density_VT.vi"("VT"=w2854, "Dielectric"=w2886) -> ("Trap Density-VT"=w2858:dbl)
                n1626 = Unbundle(w2938) -> ("[0]"=w2937:cluster{dbl[], dbl[]})  [unwired: 8 out]
                n1627 = Unbundle(w2924) -> ("[0]"=w2925:cluster{dbl[], dbl[]})  [unwired: 8 out]
                n1628 = Search 1D Array(1D array=w2939, element="Index:") -> (index of element=w2948:i32)  [unwired: 1 in]
                n1629 = local write "New: Trap Density-VT"(w2858) -> ()
                n1630 = local write "Calc: Trap Density-VT"(w2858) -> ()
                n1631 = Unbundle(w2937) -> (w2928:dbl[], w2927:dbl[])
                n1632 = Unbundle(w2925) -> (w2923:dbl[], w2922:dbl[])
                n1633 = Increment(x=w2948) -> (x+1=w2949:i32)
                n1634 = Array Subset(array=w2928, index=w2887, length=w2906) -> (w2935:dbl[])
                n1635 = Array Subset(array=w2927, index=w2887, length=w2906) -> (w2934:dbl[])
                n1636 = Array Subset(array=w2923, index=w2904, length=w2905) -> (w2930:dbl[])
                n1637 = Array Subset(array=w2922, index=w2904, length=w2905) -> (w2929:dbl[])
                n1638 = Index Array(array=w2939, index=w2949) -> (element=w2944:string)
                n1639 = local write "Vg Array-Log-Used"(w2929) -> ()
                n1640 = local write "Sat Id-Log-Used"(w2930) -> ()
                n1641 = local write "Sat Id-Used"(w2934) -> ()
                n1642 = local write "Index"(w2944) -> ()
                n1643 = local write "Sat Vg Array-Used"(w2935) -> ()
                n1644 = while {
                  tunnel: w2946 -> [w2976]
                  tunnel: w2944 -> [w2974]
                  tunnel: [w2973] -> _
                  tunnel: [w2973] -> w2945
                  tunnel: w2932 -> [w2972]
                  i -> [w2973]
                  stop <- w2969 stop-if-true
                  n1645 = Index Array(array=w2976, index=w2973) -> (element=w2977:string)
                  n1646 = xnode "Match Regular Expression"("input string"=w2977, "regular expression"=w2974) -> ("whole match"=w2975:string)  [unwired: 4 in, 4 out]
                  n1647 = Equal?(x=w2975, y=w2974) -> (x = y?=w2971:bool)
                  n1648 = Equal?(x=w2972, y=w2973) -> (x = y?=w2970:bool)
                  n1649 = Or(x=w2971, y=w2970) -> (x .or. y?=w2969:bool)
                }
                n1650 = Path To String(path=w2941) -> (string=w2943:string)
                n1651 = Index Array(array=w2946, index=w2945) -> (element=w2920:string)
                n1652 = local write "Image Name"(w2920) -> ()
                n1653 = Empty String/Path?(string/path=w2920) -> (empty?=w2921:bool)
                n1654 = Concatenate Strings(w2943, "\\", w2920) -> (w2942:string)
                n1655 = String To Path(string=w2942) -> (path=w2919:path)
                n1656 = local read "No Image File"() -> (w2918:path)
                n1657 = Select(t=w2918, s=w2921, f=w2919) -> (s? t:f=w2912:path)
                n1658 = local write "Image File"(w2912) -> ()
                n1659 = local read "Image Out"() -> (w2910:T2)
                n1660 = call "IMAQ ReadFile"("File Path"=w2912, "Image"=w2910) -> ("Image Out"=w2911:T2)  [unwired: 5 in, 4 out]
                n1661 = local write "Image Out"(w2911) -> ()
                n1662 = local write "Image Out 2"(w2911) -> ()
              }
              frame #4 {
                # "Output ROI data"
                n1663 = local read "Image Folder"() -> (w3092:path)
                n1664 = Build Path(base path=w3092, name or relative path="ROI") -> (appended path=w3094:path)
                n1665 = local read "Index"() -> (w3093:string)
                n1666 = Build Path(base path=w3094, name or relative path=w3093) -> (appended path=w3099:path)
                n1667 = invoke on="Image Out" class="ImageControl" method="Clear ROI"() -> (error out=w3098:errorcluster)  [unwired: 3 in, 2 out]
                n1668 = call <vilib>:"Check if File or Folder Exists.vi"("error in (no error)"=w3098, "path"=w3099) -> ("file or folder exists?"=w3096:bool, "dup path"=w3097:path)  [unwired: 7 in, 1 out]
                n1669 = case shown="True" w3096 {
                  tunnel: w3097 -> [_ w3100]
                  frame False {
                  }
                  frame True {
                    n1670 = Read from Text File(file (use dialog)=w3100) -> (text=w3104:string)  [unwired: 3 in, 3 out]
                    n1671 = property on="Image Out" class="ImageControl"() -> ("ROI"=w3101:T11)  [unwired: 2 in, 2 out]
                    n1672 = Unflatten From String(type=w3101, binary string=w3104) -> (value=w3102:T11, error out=w3103:errorcluster)  [unwired: 3 in, 1 out]
                    n1673 = property on="Image Out" class="ImageControl"(error in=w3103, "ROI"=w3102) -> ()  [unwired: 1 in, 2 out]
                  }
                }
              }
            }
            n1674 = flat-sequence {
              tunnel: [w2317] -> w2304
              tunnel: w2304 -> [w2331]
              frame #0 {
                # "Makes Empty File for Transformer Data"
                n1675 = local read "Transfer Folder"() -> (w2306:path)
                n1676 = Build Path(base path=w2306, name or relative path="Stats") -> (appended path=w2308:path)
                n1677 = call <vilib>:"Check if File or Folder Exists.vi"("path"=w2308) -> ("file or folder exists?"=w2309:bool, "dup path"=w2310:path)  [unwired: 8 in, 1 out]
                n1678 = case shown="False" w2309 {
                  tunnel: [w2314 w2316] -> w2311
                  tunnel: w2310 -> [w2315 w2316]
                  frame False {
                    n1679 = Create Folder(path (use dialog)=w2315) -> (created path=w2314:path)  [unwired: 2 in, 2 out]
                  }
                  frame True {
                  }
                }
                n1680 = Build Path(base path=w2311, name or relative path="Tranformer Data.txt") -> (appended path=w2313:path)
                n1681 = call-poly <vilib>:"Write To Spreadsheet File.vi"("append to file? (new file:F)"=TRUE, "file path (dialog if empty)"=w2313) -> ()  [unwired: 6 in, 1 out]
              }
              frame #1 {
                # "Adds Headers if they don't exist"
                n1682 = local read "Transfer Folder"() -> (w2323:path)
                n1683 = Concatenate Strings("Stats\\", "Tranformer Data.txt") -> (w2324:string)
                n1684 = Build Path(base path=w2323, name or relative path=w2324) -> (appended path=w2317:path)
                n1685 = call-poly <vilib>:"Read From Spreadsheet File.vi"("file path (dialog if empty)"=w2317) -> ("first row"=w2322:string[])  [unwired: 6 in, 4 out]
                n1686 = Search 1D Array(1D array=w2322, element="DeviceID") -> (index of element=w2320:i32)  [unwired: 1 in]
                n1687 = Equal?(x=w2320, y=0) -> (x = y?=w2318:bool)
                n1688 = case shown="False" w2318 {
                  tunnel: w2317 -> [w2328 _]
                  frame False {
                    n1689 = local read "Transformer \nHeaders"() -> (w2327:string[])
                    n1690 = call-poly <vilib>:"Write To Spreadsheet File.vi"("1D data"=w2327, "file path (dialog if empty)"=w2328) -> ()  [unwired: 6 in, 1 out]
                  }
                  frame True {
                  }
                }
              }
              frame #2 {
                # "Adds current device if it doesn't exist"
                n1691 = local read "Current \nRecord"() -> (w2334:string[])
                n1692 = Index Array(array=w2334, index=0) -> (element=w2333:string)
                n1693 = local read "Transfer Folder"() -> (w2336:path)
                n1694 = Concatenate Strings("Stats\\", "Tranformer Data.txt") -> (w2337:string)
                n1695 = local write "Current Device ID"(w2333) -> ()
                n1696 = local read "Current Device ID"() -> (w2343:string)
                n1697 = Build Path(base path=w2336, name or relative path=w2337) -> (appended path=w2335:path)
                n1698 = call-poly <vilib>:"Read From Spreadsheet File.vi"("file path (dialog if empty)"=w2335) -> ("all rows"=w2330:string[][])  [unwired: 6 in, 4 out]
                n1699 = Index Array(array=w2330, index (col)=0) -> (element=w2341:string[])  [unwired: 1 in]
                n1700 = Search 1D Array(1D array=w2341, element=w2343) -> (index of element=w2329:i32)  [unwired: 1 in]
                n1701 = Equal?(x=w2329, y=-1) -> (x = y?=w2332:bool)
                n1702 = case shown="False" w2332 {
                  tunnel: w2331 -> [w2345 w2358]
                  tunnel: w2329 -> [w2350 _]
                  tunnel: w2330 -> [w2351 _]
                  frame False {
                    n1703 = local read "Current \nRecord"() -> (w2349:string[])
                    n1704 = Replace Array Subset(array=w2351, new element=w2349, index (row)=w2350) -> (w2346:string[][])  [unwired: 1 in]
                    n1705 = flat-sequence {
                      tunnel: [w2352] -> _
                      tunnel: [w2353] -> _
                      tunnel: [w2353] -> w2348
                      tunnel: [w2352] -> w2347
                      tunnel: w2346 -> [w2353]
                      tunnel: w2345 -> [w2352]
                      tunnel: w2348 -> [w2355]
                      tunnel: w2347 -> [w2354]
                      frame #0 {
                        n1706 = Delete(path (use dialog)=w2352) -> ()  [unwired: 4 in, 3 out]
                      }
                      frame #1 {
                        n1707 = call-poly <vilib>:"Write To Spreadsheet File.vi"("append to file? (new file:F)"=TRUE, "2D data"=w2355, "file path (dialog if empty)"=w2354) -> ()  [unwired: 5 in, 1 out]
                      }
                    }
                  }
                  frame True {
                    n1708 = local read "Current \nRecord"() -> (w2357:string[])
                    n1709 = call-poly <vilib>:"Write To Spreadsheet File.vi"("append to file? (new file:F)"=TRUE, "1D data"=w2357, "file path (dialog if empty)"=w2358) -> ()  [unwired: 5 in, 1 out]
                  }
                }
              }
            }
          }
          event "Export": Mouse Down {
            n1710 = event-data() -> ()  [unwired: 1 in, 7 out]
            n1711 = flat-sequence {
              frame #0 {
                n1712 = stacked-sequence {
                  frame #0 {
                    n1713 = local read "Independant Variable"() -> (w3106:string)
                    n1714 = Equal?(x=w3106, y="Length (um):") -> (x = y?=w3107:bool)
                    n1715 = case shown="True" w3107 {
                      frame False {
                      }
                      frame True {
                        n1716 = local write "X Axis Display Type"("1") -> ()
                        n1717 = local write "Opj X Axis"("2") -> ()
                      }
                    }
                  }
                  frame #1 {
                    n1718 = local read "Independant Variable"() -> (w3111:string)
                    n1719 = Equal?(x=w3111, y="Sample Temp (K):") -> (x = y?=w3112:bool)
                    n1720 = case shown="True" w3112 {
                      frame False {
                      }
                      frame True {
                        n1721 = local write "X Axis Display Type"("1") -> ()
                        n1722 = local write "Opj X Axis"("1") -> ()
                      }
                    }
                  }
                  frame #2 {
                    n1723 = local read "Independant Variable"() -> (w3116:string)
                    n1724 = Equal?(x=w3116, y="Mobility-Sat (cm^2/Vs):") -> (x = y?=w3117:bool)
                    n1725 = case shown="True" w3117 {
                      frame False {
                      }
                      frame True {
                        n1726 = local write "X Axis Display Type"("2") -> ()
                        n1727 = local write "Opj X Axis"("2") -> ()
                      }
                    }
                  }
                  frame #3 {
                    n1728 = local read "Independant Variable"() -> (w3121:string)
                    n1729 = Equal?(x=w3121, y="Mobility-Lin (cm^2/Vs):") -> (x = y?=w3122:bool)
                    n1730 = case shown="True" w3122 {
                      frame False {
                      }
                      frame True {
                        n1731 = local write "X Axis Display Type"("2") -> ()
                        n1732 = local write "Opj X Axis"("2") -> ()
                      }
                    }
                  }
                  frame #4 {
                    n1733 = local read "Independant Variable"() -> (w3126:string)
                    n1734 = Equal?(x=w3126, y="On/Off I-Sat:") -> (x = y?=w3127:bool)
                    n1735 = case shown="True" w3127 {
                      frame False {
                      }
                      frame True {
                        n1736 = local write "X Axis Display Type"("2") -> ()
                        n1737 = local write "Opj X Axis"("2") -> ()
                      }
                    }
                  }
                  frame #5 {
                    n1738 = local read "Independant Variable"() -> (w3131:string)
                    n1739 = Equal?(x=w3131, y="Off I-Sat (A):") -> (x = y?=w3132:bool)
                    n1740 = case shown="True" w3132 {
                      frame False {
                      }
                      frame True {
                        n1741 = local write "X Axis Display Type"("2") -> ()
                        n1742 = local write "Opj X Axis"("2") -> ()
                      }
                    }
                  }
                  frame #6 {
                    n1743 = local read "Independant Variable"() -> (w3136:string)
                    n1744 = Equal?(x=w3136, y="Vt-Sat (V):") -> (x = y?=w3137:bool)
                    n1745 = case shown="True" w3137 {
                      frame False {
                      }
                      frame True {
                        n1746 = local write "X Axis Display Type"("1") -> ()
                        n1747 = local write "Opj X Axis"("1") -> ()
                      }
                    }
                  }
                  frame #7 {
                    n1748 = local read "Independant Variable"() -> (w3141:string)
                    n1749 = Equal?(x=w3141, y="STS-Sat (V/decade):") -> (x = y?=w3142:bool)
                    n1750 = case shown="True" w3142 {
                      frame False {
                      }
                      frame True {
                        n1751 = local write "X Axis Display Type"("1") -> ()
                        n1752 = local write "Opj X Axis"("1") -> ()
                      }
                    }
                  }
                  frame #8 {
                    n1753 = local read "Independant Variable"() -> (w3146:string)
                    n1754 = Equal?(x=w3146, y="Trap Density-VT (Traps/Vcm^2):") -> (x = y?=w3147:bool)
                    n1755 = case shown="True" w3147 {
                      frame False {
                      }
                      frame True {
                        n1756 = local write "X Axis Display Type"("2") -> ()
                        n1757 = local write "Opj X Axis"("2") -> ()
                      }
                    }
                  }
                  frame #9 {
                    n1758 = local read "Independant Variable"() -> (w3151:string)
                    n1759 = Equal?(x=w3151, y="Trap Density-STS (Traps/Vcm^2):") -> (x = y?=w3152:bool)
                    n1760 = case shown="True" w3152 {
                      frame False {
                      }
                      frame True {
                        n1761 = local write "X Axis Display Type"("2") -> ()
                        n1762 = local write "Opj X Axis"("2") -> ()
                      }
                    }
                  }
                }
              }
              frame #1 {
                n1763 = local read "Transfer Folder"() -> (w3160:path)
                n1764 = Build Path(base path=w3160, name or relative path="Stats") -> (appended path=w3161:path)
                n1765 = local read "Origin Project File"() -> (w3172:path)
                n1766 = call <vilib>:"Check if File or Folder Exists.vi"("path"=w3161) -> ("file or folder exists?"=w3176:bool, "dup path"=w3175:path)  [unwired: 8 in, 1 out]
                n1767 = call <userlib>:"OA_ConnectToOrigin.vi"() -> ("error out"=w3173:errorcluster, "Origin.IOApplication"=w3174:refnum<k7>)  [unwired: 8 in]
                n1768 = case shown="False" w3176 {
                  tunnel: w3175 -> [w3349 w3350]
                  tunnel: [w3348 w3350] -> w3159
                  frame False {
                    n1769 = Create Folder(path (use dialog)=w3349) -> (created path=w3348:path)  [unwired: 2 in, 2 out]
                  }
                  frame True {
                  }
                }
                n1770 = call <userlib>:"OA_Load.vi"("error in (no error)"=w3173, "Path"=w3172, "Origin.IOApplication"=w3174) -> ("error out"=w3170:errorcluster, "Origin.IOApplication"=w3171:refnum<k7>)  [unwired: 1 out]
                n1771 = call <userlib>:"OAExecute.vi"("script"="document -m 3;", "Error IO"=w3170, "Origin.IOApplication"=w3171) -> ("Error IO Out"=w3168:errorcluster, "Origin.IOApplication"=w3169:refnum<k7>)  [unwired: 1 in, 1 out]
                n1772 = call "File Dialog"("start path"=w3161) -> ("selected path"=w3163:path)  [unwired: 11 in, 3 out]
                n1773 = local read "Independant Variable"() -> (w3156:string)
                n1774 = stacked-sequence {
                  tunnel: w3160 -> [w3187 w3217 w3229 w3251 w3271 w3292 w3313 w3336]
                  tunnel: w3159 -> [w3188 w3216 w3230 w3250 w3272 w3293 w3314 w3337]
                  tunnel: w3169 -> [w3190 w3214 w3232 w3253 w3274 w3295 w3316 w3339]
                  tunnel: w3168 -> [w3189 w3215 w3231 w3252 w3273 w3294 w3315 w3338]
                  tunnel: [_ _ _ _ _ _ _ w3334] -> w3158
                  tunnel: [_ _ _ _ _ _ _ w3335] -> w3157
                  tunnel: w3156 -> [w3186 w3207 w3228 w3249 w3270 w3291 w3312 w3333]
                  frame #0 {
                    n1775 = local read "X Axis Display Type"() -> (w3178:string)
                    n1776 = local read "Opj X Axis"() -> (w3183:string)
                    n1777 = Concatenate Strings("window -a MOBLGraph;\nlayer.x.type=", w3183, "; layer.x.label.numFormat = ", w3178, "; Y3 = 1; X3 = 1;", "window -a MOBLTable;\nwindow -s TV;") -> (w3181:string)
                    n1778 = call "Param_Analysis_7_24b_JW.vi"("Independant Variable"=w3186, "error in (no error)"=w3189, "Data Folder"=w3187, "Parameter String"="Mobility-Lin (cm^2/Vs):", "Parameter Name"="Mobility-Lin", "Stats Folder"=w3188) -> ("error out"=w3192:errorcluster, "Output Array"=w3194:string[][], "Variables"=w3185:T17)  [unwired: 2 in, 1 out]
                    n1779 = call "Origin_Export_7_27a_JW.vi"("Input Conditions"=w3185, "Analysis Array"=w3194, "error in (no error)"=w3192, "Parameter Worksheet Name"="[MOBLTable]Mobilities", "Parameter Folder Script"="pe_cd \"Mobility-Lin\";", "Origin.IOApplication"=w3190) -> ("error out"=w3191:errorcluster, "reference out"=w3193:refnum<k7>)  [unwired: 3 in, 1 out]
                    n1780 = call <userlib>:"OAExecute.vi"("script"=w3181, "Error IO"=w3191, "Origin.IOApplication"=w3193) -> ()  [unwired: 1 in, 3 out]
                  }
                  frame #1 {
                    n1781 = local read "X Axis Display Type"() -> (w3199:string)
                    n1782 = local read "Opj X Axis"() -> (w3204:string)
                    n1783 = Concatenate Strings("window -a MOBSGraph;\nlayer.x.type=", w3204, "; layer.x.label.numFormat = ", w3199, "; Y3 = 1; X3 = 1;", "window -a MOBSTable;\nwindow -s TV;") -> (w3202:string)
                    n1784 = call "Param_Analysis_7_24b_JW.vi"("Independant Variable"=w3207, "error in (no error)"=w3215, "Data Folder"=w3217, "Parameter String"="Mobility-Sat (cm^2/Vs):", "Parameter Name"="Mobility-Sat", "Stats Folder"=w3216) -> ("error out"=w3210:errorcluster, "Output Array"=w3208:string[][], "Variables"=w3206:T17)  [unwired: 2 in, 1 out]
                    n1785 = call "Origin_Export_7_27a_JW.vi"("Input Conditions"=w3206, "Analysis Array"=w3208, "error in (no error)"=w3210, "Parameter Worksheet Name"="[MOBSTable]Mobilities", "Parameter Folder Script"="pe_cd \"Mobility-Sat\";", "Origin.IOApplication"=w3214) -> ("error out"=w3209:errorcluster, "reference out"=w3211:refnum<k7>)  [unwired: 3 in, 1 out]
                    n1786 = call <userlib>:"OAExecute.vi"("script"=w3202, "Error IO"=w3209, "Origin.IOApplication"=w3211) -> ()  [unwired: 1 in, 3 out]
                  }
                  frame #2 {
                    n1787 = local read "X Axis Display Type"() -> (w3220:string)
                    n1788 = local read "Opj X Axis"() -> (w3225:string)
                    n1789 = Concatenate Strings("window -a NSTSGraph;\nlayer.x.type=", w3225, "; layer.x.label.numFormat = ", w3220, "; Y3 = 1; X3 = 1;", "window -a NSTSTable;\nwindow -s TV;") -> (w3223:string)
                    n1790 = call "Param_Analysis_7_24b_JW.vi"("Independant Variable"=w3228, "error in (no error)"=w3231, "Data Folder"=w3229, "Parameter String"="Trap Density-STS (Traps/Vcm^2):", "Parameter Name"="Trap Density-STS", "Stats Folder"=w3230) -> ("error out"=w3235:errorcluster, "Output Array"=w3233:string[][], "Variables"=w3227:T17)  [unwired: 2 in, 1 out]
                    n1791 = call "Origin_Export_7_27a_JW.vi"("Input Conditions"=w3227, "Analysis Array"=w3233, "error in (no error)"=w3235, "Parameter Worksheet Name"="[NSTSTable]Trap Densities", "Parameter Folder Script"="pe_cd \"N-STS\";", "Origin.IOApplication"=w3232) -> ("error out"=w3234:errorcluster, "reference out"=w3236:refnum<k7>)  [unwired: 3 in, 1 out]
                    n1792 = call <userlib>:"OAExecute.vi"("script"=w3223, "Error IO"=w3234, "Origin.IOApplication"=w3236) -> ()  [unwired: 1 in, 3 out]
                  }
                  frame #3 {
                    n1793 = local read "X Axis Display Type"() -> (w3241:string)
                    n1794 = local read "Opj X Axis"() -> (w3246:string)
                    n1795 = call "Param_Analysis_7_24b_JW.vi"("Independant Variable"=w3249, "error in (no error)"=w3252, "Data Folder"=w3251, "Parameter String"="Trap Density-VT (Traps/Vcm^2):", "Parameter Name"="Trap Density-Vt", "Stats Folder"=w3250) -> ("error out"=w3256:errorcluster, "Output Array"=w3254:string[][], "Variables"=w3248:T17)  [unwired: 2 in, 1 out]
                    n1796 = Concatenate Strings("window -a NVtGraph;\nlayer.x.type=", w3246, "; layer.x.label.numFormat = ", w3241, "; Y3 = 1; X3 = 1;", "window -a NVtTable;\nwindow -s TV;") -> (w3244:string)
                    n1797 = call "Origin_Export_7_27a_JW.vi"("Input Conditions"=w3248, "Analysis Array"=w3254, "error in (no error)"=w3256, "Parameter Worksheet Name"="[NVTTable]Trap Densities", "Parameter Folder Script"="pe_cd \"N-Vt\";", "Origin.IOApplication"=w3253) -> ("error out"=w3255:errorcluster, "reference out"=w3257:refnum<k7>)  [unwired: 3 in, 1 out]
                    n1798 = call <userlib>:"OAExecute.vi"("script"=w3244, "Error IO"=w3255, "Origin.IOApplication"=w3257) -> ()  [unwired: 1 in, 3 out]
                  }
                  frame #4 {
                    n1799 = local read "X Axis Display Type"() -> (w3262:string)
                    n1800 = local read "Opj X Axis"() -> (w3267:string)
                    n1801 = Concatenate Strings("window -a OffIGraph;\nlayer.x.type=", w3267, "; layer.x.label.numFormat = ", w3262, "; Y3 = 1; X3 = 1;", "window -a OffITable;\nwindow -s TV;") -> (w3265:string)
                    n1802 = call "Param_Analysis_7_24b_JW.vi"("Independant Variable"=w3270, "error in (no error)"=w3273, "Data Folder"=w3271, "Parameter String"="Off I-Sat (A):", "Parameter Name"="Off I-Sat", "Stats Folder"=w3272) -> ("error out"=w3277:errorcluster, "Output Array"=w3275:string[][], "Variables"=w3269:T17)  [unwired: 2 in, 1 out]
                    n1803 = call "Origin_Export_7_27a_JW.vi"("Input Conditions"=w3269, "Analysis Array"=w3275, "error in (no error)"=w3277, "Parameter Worksheet Name"="[OffItable]OffCurrents", "Parameter Folder Script"="pe_cd \"OffI-Sat\";", "Origin.IOApplication"=w3274) -> ("error out"=w3276:errorcluster, "reference out"=w3278:refnum<k7>)  [unwired: 3 in, 1 out]
                    n1804 = call <userlib>:"OAExecute.vi"("script"=w3265, "Error IO"=w3276, "Origin.IOApplication"=w3278) -> ()  [unwired: 1 in, 3 out]
                  }
                  frame #5 {
                    n1805 = local read "X Axis Display Type"() -> (w3283:string)
                    n1806 = local read "Opj X Axis"() -> (w3288:string)
                    n1807 = Concatenate Strings("window -a OnOffGraph;\nlayer.x.type=", w3288, "; layer.x.label.numFormat = ", w3283, "; Y3 = 1; X3 = 1;", "window -a OnOffTable;\nwindow -s TV;") -> (w3286:string)
                    n1808 = call "Param_Analysis_7_24b_JW.vi"("Independant Variable"=w3291, "error in (no error)"=w3294, "Data Folder"=w3292, "Parameter String"="On/Off I-Sat:", "Parameter Name"="OnOff Ratio", "Stats Folder"=w3293) -> ("error out"=w3298:errorcluster, "Output Array"=w3296:string[][], "Variables"=w3290:T17)  [unwired: 2 in, 1 out]
                    n1809 = call "Origin_Export_7_27a_JW.vi"("Input Conditions"=w3290, "Analysis Array"=w3296, "error in (no error)"=w3298, "Parameter Worksheet Name"="[OnOffTable]On/Off Ratios", "Parameter Folder Script"="pe_cd \"OnOff-Ratio\";", "Origin.IOApplication"=w3295) -> ("error out"=w3297:errorcluster, "reference out"=w3299:refnum<k7>)  [unwired: 3 in, 1 out]
                    n1810 = call <userlib>:"OAExecute.vi"("script"=w3286, "Error IO"=w3297, "Origin.IOApplication"=w3299) -> ()  [unwired: 1 in, 3 out]
                  }
                  frame #6 {
                    n1811 = local read "X Axis Display Type"() -> (w3304:string)
                    n1812 = local read "Opj X Axis"() -> (w3309:string)
                    n1813 = call "Param_Analysis_7_24b_JW.vi"("Independant Variable"=w3312, "error in (no error)"=w3315, "Data Folder"=w3313, "Parameter String"="STS-Sat (V/decade):", "Parameter Name"="STS-Sat", "Stats Folder"=w3314) -> ("error out"=w3319:errorcluster, "Output Array"=w3317:string[][], "Variables"=w3311:T17)  [unwired: 2 in, 1 out]
                    n1814 = Concatenate Strings("window -a SGraph;\nlayer.x.type=", w3309, "; layer.x.label.numFormat = ", w3304, "; Y3 = 1; X3 = 1;", "window -a STable;\nwindow -s TV;") -> (w3307:string)
                    n1815 = call "Origin_Export_7_27a_JW.vi"("Input Conditions"=w3311, "Analysis Array"=w3317, "error in (no error)"=w3319, "Parameter Worksheet Name"="[STable]Threshold Swing", "Parameter Folder Script"="pe_cd \"STS-Sat\";", "Origin.IOApplication"=w3316) -> ("error out"=w3318:errorcluster, "reference out"=w3320:refnum<k7>)  [unwired: 3 in, 1 out]
                    n1816 = call <userlib>:"OAExecute.vi"("script"=w3307, "Error IO"=w3318, "Origin.IOApplication"=w3320) -> ()  [unwired: 1 in, 3 out]
                  }
                  frame #7 {
                    n1817 = local read "X Axis Display Type"() -> (w3325:string)
                    n1818 = local read "Opj X Axis"() -> (w3330:string)
                    n1819 = Concatenate Strings("window -a VtGraph;\nlayer.x.type=", w3330, "; layer.x.label.numFormat = ", w3325, "; Y3 = 1; X3 = 1;", "window -a VtTable;\nwindow -s TV;") -> (w3328:string)
                    n1820 = call "Param_Analysis_7_24b_JW.vi"("Independant Variable"=w3333, "error in (no error)"=w3338, "Data Folder"=w3336, "Parameter String"="Vt-Sat (V):", "Parameter Name"="Vt-Sat", "Stats Folder"=w3337) -> ("error out"=w3342:errorcluster, "Output Array"=w3340:string[][], "Variables"=w3332:T17)  [unwired: 2 in, 1 out]
                    n1821 = call "Origin_Export_7_27a_JW.vi"("Input Conditions"=w3332, "Analysis Array"=w3340, "error in (no error)"=w3342, "Parameter Worksheet Name"="[VtTable]Threshold Voltages", "Parameter Folder Script"="pe_cd \"Vt-Sat\";", "Origin.IOApplication"=w3339) -> ("error out"=w3341:errorcluster, "reference out"=w3343:refnum<k7>)  [unwired: 3 in, 1 out]
                    n1822 = call <userlib>:"OAExecute.vi"("script"=w3328, "Error IO"=w3341, "Origin.IOApplication"=w3343) -> ("Error IO Out"=w3334:errorcluster, "Origin.IOApplication"=w3335:refnum<k7>)  [unwired: 1 in, 1 out]
                  }
                }
                n1823 = Path To String(path=w3163) -> (string=w3162:string)
                n1824 = call <userlib>:"OAExecute.vi"("script"="pe_cd /; ", "Error IO"=w3158, "Origin.IOApplication"=w3157) -> ("Error IO Out"=w3164:errorcluster, "Origin.IOApplication"=w3165:refnum<k7>)  [unwired: 1 in, 1 out]
                n1825 = call <userlib>:"OASaveProject.vi"("path"=w3162, "Error IO"=w3164, "Origin.IOApplication"=w3165) -> ()  [unwired: 3 out]
              }
            }
          }
          event "Blank Button": Mouse Down {
            n1826 = event-data() -> ()  [unwired: 1 in, 7 out]
            n1827 = local read "Transfer File"() -> (w3358:path)
            n1828 = disable-structure shown="Disabled" {
              frame Disabled {
                n1829 = local read "Folder Index"() -> (w3359:dbl)
                n1830 = Decrement(x=w3359) -> (x-1=w3360:dbl)
                n1831 = local write "Folder Index"(w3360) -> ()
              }
              frame Enabled {
              }
            }
            n1832 = Strip Path(path=w3358) -> (stripped path=w3354:path, name=w3356:string)
            n1833 = Path To String(path=w3354) -> (string=w3353:string)
            n1834 = Concatenate Strings(w3353, "\\", "X_", w3356) -> (w3352:string)
            n1835 = String To Path(string=w3352) -> (path=w3351:path)
            n1836 = Move(source path=w3358, 10:w3351) -> ()  [unwired: 3 in, 3 out]
            n1837 = local write "Transfer File"(w3351) -> ()
          }
          event "Cancel Button": Mouse Down {
            (unwired) 6
            n1838 = event-data() -> ()  [unwired: 1 in, 7 out]
            n1839 = call "Simulate_Keyboard.vi"("Action"=2, "Virtual Key"=162) -> ()  [unwired: 7 in, 1 out]
          }
        }
        n1840 = Multiply(x=w526, y=10) -> (x*y=w528:sgl)
        n1841 = case shown="\"0\"" w567 {
          tunnel: w541 -> [w638 w644 w648 w650 w654 w656 w658 w660 w662 w664 w666 w668 w670 w672 w674 w676 w678 w680 w682 w684 w686 w688 w690 w692 w694 w696 w698 w700 w702 w704 w706 w708 w710 w712 w714 w716 w718 w720 w722 w724 w726 w728 w730 w732 w734 w736 w738 w740 w742 w744 w746 w748 w750 w752 w754 w756 w758 w760 w762 w764 w766 w768 w770 w772 w774 w776 w778 w780 w782 w784 w786 w788 w790 w792 w794 w796 w798 w800 w802 w804 w806 w808 w810 w812 w814 w816 w818 w820 w822 w824 w826 w828 w830 w832 w834 w836 w838 w840 w842 w844 w846 w848 w850 w852 w854]
          tunnel: [w638 w643 w647 w650 w654 w656 w658 w660 w662 w664 w666 w668 w670 w672 w674 w676 w678 w680 w682 w684 w686 w688 w690 w692 w694 w696 w698 w700 w702 w704 w706 w708 w710 w712 w714 w716 w718 w720 w722 w724 w726 w728 w730 w732 w734 w736 w738 w740 w742 w744 w746 w748 w750 w752 w754 w756 w758 w760 w762 w764 w766 w768 w770 w772 w774 w776 w778 w780 w782 w784 w786 w788 w790 w792 w794 w796 w798 w800 w802 w804 w806 w808 w810 w812 w814 w816 w818 w820 w822 w824 w826 w828 w830 w832 w834 w836 w838 w840 w842 w844 w846 w848 w850 w852 w854] -> w566
          tunnel: w542 -> [w640 w642 w646 w652 w653 w655 w657 w659 w661 w663 w665 w667 w669 w671 w673 w675 w677 w679 w681 w683 w685 w687 w689 w691 w693 w695 w697 w699 w701 w703 w705 w707 w709 w711 w713 w715 w717 w719 w721 w723 w725 w727 w729 w731 w733 w735 w737 w739 w741 w743 w745 w747 w749 w751 w753 w755 w757 w759 w761 w763 w765 w767 w769 w771 w773 w775 w777 w779 w781 w783 w785 w787 w789 w791 w793 w795 w797 w799 w801 w803 w805 w807 w809 w811 w813 w815 w817 w819 w821 w823 w825 w827 w829 w831 w833 w835 w837 w839 w841 w843 w845 w847 w849 w851 w853]
          tunnel: [w639 w642 w646 w651 w653 w655 w657 w659 w661 w663 w665 w667 w669 w671 w673 w675 w677 w679 w681 w683 w685 w687 w689 w691 w693 w695 w697 w699 w701 w703 w705 w707 w709 w711 w713 w715 w717 w719 w721 w723 w725 w727 w729 w731 w733 w735 w737 w739 w741 w743 w745 w747 w749 w751 w753 w755 w757 w759 w761 w763 w765 w767 w769 w771 w773 w775 w777 w779 w781 w783 w785 w787 w789 w791 w793 w795 w797 w799 w801 w803 w805 w807 w809 w811 w813 w815 w817 w819 w821 w823 w825 w827 w829 w831 w833 w835 w837 w839 w841 w843 w845 w847 w849 w851 w853] -> w565
          tunnel: w528 -> [w637 w641 w645 w649 _ _ _ _ _ _ _ _ _ _ _ _ _ _ _ _ _ _ _ _ _ _ _ _ _ _ _ _ _ _ _ _ _ _ _ _ _ _ _ _ _ _ _ _ _ _ _ _ _ _ _ _ _ _ _ _ _ _ _ _ _ _ _ _ _ _ _ _ _ _ _ _ _ _ _ _ _ _ _ _ _ _ _ _ _ _ _ _ _ _ _ _ _ _ _ _ _ _ _ _ _]
          frame "DOWN" {
            n1842 = Add(x=w640, y=w637) -> (x+y=w639:sgl)
          }
          frame "LEFT" {
            n1843 = Subtract(x=w644, y=w641) -> (x-y=w643:sgl)
          }
          frame "RIGHT" {
            n1844 = Add(x=w648, y=w645) -> (x+y=w647:sgl)
          }
          frame "UP" {
            n1845 = Subtract(x=w652, y=w649) -> (x-y=w651:sgl)
          }
          frame "ENTER (num pad)" {
          }
          frame "' (quote)" {
          }
          frame "END" {
          }
          frame "EQUALS" {
          }
          frame "ESCAPE" {
          }
          frame "GRAVE (`)" {
          }
          frame "HOME" {
          }
          frame "INSERT" {
          }
          frame "LBRACKET" {
          }
          frame "LCONTROL" {
          }
          frame "L ALT" {
          }
          frame "LSHIFT" {
          }
          frame "LWIN" {
          }
          frame "MINUS" {
          }
          frame "MULTIPLY" {
          }
          frame "NEXT" {
          }
          frame "NUMLOCK" {
          }
          frame "NUMPAD_0" {
          }
          frame "NUMPAD_1" {
          }
          frame "NUMPAD_2" {
          }
          frame "NUMPAD_3" {
          }
          frame "NUMPAD_4" {
          }
          frame "NUMPAD_5" {
          }
          frame "NUMPAD_6" {
          }
          frame "NUMPAD_7" {
          }
          frame "NUMPAD_8" {
          }
          frame "NUMPAD_9" {
          }
          frame "PAUSE" {
          }
          frame "PERIOD" {
          }
          frame "PRIOR (PG UP)" {
          }
          frame "RBRACKET" {
          }
          frame "RCONTROL" {
          }
          frame "RETURN" {
          }
          frame "R ALT" {
          }
          frame "RSHIFT" {
          }
          frame "RWIN" {
          }
          frame "SCROLL" {
          }
          frame "SEMICOLON" {
          }
          frame "SLASH" {
          }
          frame "SPACE" {
          }
          frame "SUBTRACT" {
          }
          frame "TAB" {
          }
          frame "DIVIDE" {
          }
          frame "DELETE" {
          }
          frame "DECIMAL" {
          }
          frame "COMMA" {
          }
          frame "CAPITAL" {
          }
          frame "BACKSLASH" {
          }
          frame "BACK" {
          }
          frame "ADD" {
          }
          frame "F15" {
          }
          frame "F14" {
          }
          frame "F13" {
          }
          frame "F12" {
          }
          frame "F11" {
          }
          frame "F10" {
          }
          frame "F9" {
          }
          frame "F8" {
          }
          frame "F7" {
          }
          frame "F6" {
          }
          frame "F5" {
          }
          frame "F4" {
          }
          frame "F3" {
          }
          frame "F2" {
          }
          frame "F1" {
          }
          frame "Z" {
          }
          frame "Y" {
          }
          frame "X" {
          }
          frame "W" {
          }
          frame "V" {
          }
          frame "U" {
          }
          frame "T" {
          }
          frame "S" {
          }
          frame "R" {
          }
          frame "Q" {
          }
          frame "P" {
          }
          frame "O" {
          }
          frame "N" {
          }
          frame "M" {
          }
          frame "L" {
          }
          frame "K" {
          }
          frame "J" {
          }
          frame "I" {
          }
          frame "H" {
          }
          frame "G" {
          }
          frame "F" {
          }
          frame "E" {
          }
          frame "D" {
          }
          frame "C" {
          }
          frame "B" {
          }
          frame "A" {
          }
          frame "9" {
          }
          frame "8" {
          }
          frame "7" {
          }
          frame "6" {
          }
          frame "5" {
          }
          frame "4" {
          }
          frame "3" {
          }
          frame "2" {
          }
          frame "1" {
          }
          frame "0" {
          }
        }
        n1846 = Bundle(w544, w543, w558, w557, 0.0) -> (w556:cluster{dbl, dbl, dbl, dbl, dbl})  [unwired: 1 in]
        n1847 = Bundle("X"=w566, "Y"=w565) -> (w560:cluster{"X":sgl, "Y":sgl})  [unwired: 1 in]
        n1848 = Divide(x=20, y=w527) -> (x/y=w530:sgl)
        n1849 = property on="Image Out" class="ImageControl"("Image Center Position"=w560) -> ()  [unwired: 2 in, 2 out]
        n1850 = call "IMAQ Convert Rectangle to ROI (Polygon)"("Rectangle"=w556) -> ("ROI Descriptor"=w554:T3)  [unwired: 7 in, 2 out]
        n1851 = Bundle("Application Font", w530, w534, w534, w534, w534, w534, TRUE, w532) -> (w536:T18)  [unwired: 1 in]
        n1852 = property on="Image Out 2" class="ImageControl"("ROI"=w554) -> ()  [unwired: 2 in, 2 out]
        n1853 = Bundle(w532, w536, w532, w532) -> (w535:T19)  [unwired: 1 in]
        n1854 = property on="Image Out" class="ImageControl"() -> ("ROI"=w519:T11)  [unwired: 2 in, 2 out]
        n1855 = Unbundle By Name(w519) -> ("Contours"=w583:T15)
        n1856 = local read "Image Out"() -> (w538:T2)
        n1857 = call "IMAQ Clear Overlay"("Image"=w538) -> ("Image Out"=w537:T2)  [unwired: 9 in, 1 out]
        n1858 = Initialize Array(0) -> (w581:i32[])  [unwired: 1 in]
        n1859 = local read "Magnification"() -> (w572:u16)
        n1860 = Array Size(array=w583) -> (size(s)=w582:i32)
        n1861 = Build Array(0.505025, 0.252522, 0.127742, 0.050345, 0.031129) -> (w573:dbl[])
        n1862 = Array Subset(array=w573, index=w572, length=1) -> (w570:dbl[])
        n1863 = property on="Image Out" class="ImageControl"() -> ("ZoomInteger"=w562:cluster{"X":i32, "Y":i32})  [unwired: 2 in, 2 out]
        n1864 = To Double Precision Float(number=w570) -> (double precision float=w569:dbl[])
        n1865 = for {
          N: w582 -> [_]
          shift-right: [w877] -> _
          shift-left: w583 -> [w877]
          shift-right: [w875] -> w568
          shift-left: w581 -> [w874]
          tunnel: w569 -> [w873]
          shift-right: [w870] -> _
          shift-left: w537 -> [w872]
          tunnel: w535 -> [w865]
          i -> [w869]
          n1866 = Index Array(array=w877, index=w869) -> (element=w886:T20)
          n1867 = Unbundle(w886) -> ("Points"=w885:i32[])  [unwired: 2 out]
          n1868 = Array To Cluster(array=w885) -> (cluster=w884:T21)
          n1869 = Unbundle(w884) -> ("Points[0]"=w864:i32, "Points[1]"=w861:i32, "Points[2]"=w876:i32, "Points[3]"=w882:i32)  [unwired: 5 out]
          n1870 = Add(x=w864, y=10) -> (x+y=w862:i32)
          n1871 = Subtract(x=w861, y=w882) -> (x-y=w881:i32)
          n1872 = Subtract(x=w864, y=w876) -> (x-y=w883:i32)
          n1873 = Square(x=w881) -> (x^2=w879:i32)
          n1874 = Square(x=w883) -> (x^2=w880:i32)
          n1875 = Add(x=w880, y=w879) -> (x+y=w878:i32)
          n1876 = Square Root(x=w878) -> (sqrt(x)=w855:dbl)
          n1877 = Multiply(x=w855, y=0.5) -> (x*y=w858:dbl)
          n1878 = Add(x=w858, y=w861) -> (x+y=w860:dbl)
          n1879 = Bundle(w862, w860) -> (w871:cluster{i32, dbl})  [unwired: 1 in]
          n1880 = Multiply(x=w855, y=w873) -> (x*y=w868:dbl[])
          n1881 = Index Array(array=w868) -> (element=w867:dbl)  [unwired: 1 in]
          n1882 = Number To Fractional String(number=w867) -> (F-format string=w866:string)  [unwired: 3 in]
          n1883 = call "IMAQ Overlay Text"("BG Color (Transparent)"=u32 0, "Text Color (black)"=u32 16448250, "Font, Size & Style"=w865, "String"=w866, "Origin"=w871, "Image"=w872) -> ("Image Out"=w870:T2)  [unwired: 4 in, 1 out]
          n1884 = Build Array (concatenate)(w874, w868) -> (w875:dbl[])
          n1885 = local write "Numeric 3"(w855) -> ()
        }
        n1886 = local write "ROI Descriptor"(w519) -> ()
        n1887 = Unbundle(w562) -> ("X"=w561:i32)  [unwired: 1 out]
        n1888 = Add Array Elements(numeric array=w568) -> (sum=w579:dbl)
        n1889 = local write "Distances"(w568) -> ()
        n1890 = local write "Total Width"(w579) -> ()
        n1891 = local write "Zoom"(w561) -> ()
        n1892 = local read "Manual-Width"() -> (w417:bool)
        n1893 = local read "Total Width"() -> (w522:dbl)
        n1894 = local read "Rec: Width"() -> (w520:dbl)
        n1895 = case shown="False" w417 {
          frame False {
            n1896 = property on="New: Width" class="DigNum (strict)"("DisabledEnum"=1) -> ()  [unwired: 2 in, 2 out]
          }
          frame True {
            n1897 = property on="New: Width" class="DigNum (strict)"("DisabledEnum"=0) -> ()  [unwired: 2 in, 2 out]
          }
        }
        n1898 = Not(x=w417) -> (.not. x?=w517:bool)
        n1899 = Equal To 0?(x=w522) -> (x = 0?=w518:bool)
        n1900 = Or(x=w518, y=w417) -> (x .or. y?=w521:bool)
        n1901 = And(x=w518, y=w517) -> (x .and. y?=w516:bool)
        n1902 = case shown="True" w516 {
          tunnel: w520 -> [_ w613]
          frame False {
          }
          frame True {
            n1903 = local write "New: Width"(w613) -> ()
          }
        }
        n1904 = case shown="False" w521 {
          tunnel: w522 -> [w615 _]
          frame False {
            n1905 = local write "New: Width"(w615) -> ()
            n1906 = property on="New: Width" class="DigNum (strict)"("DisabledEnum"=1) -> ()  [unwired: 2 in, 2 out]
          }
          frame True {
            n1907 = property on="New: Width" class="DigNum (strict)"("DisabledEnum"=0) -> ()  [unwired: 2 in, 2 out]
          }
        }
        n1908 = local read "Manual Comments"() -> (w418:bool)
        n1909 = local read "Rec: Comments"() -> (w419:string)
        n1910 = local read "Manuel-Dielectric"() -> (w445:bool)
        n1911 = local read "Rec: Dielectric (d)"() -> (w444:dbl)
        n1912 = local read "Manuel-Length"() -> (w446:bool)
        n1913 = local read "Rec: Length"() -> (w447:dbl)
        n1914 = case shown="True" w418 {
          tunnel: w419 -> [w588 _]
          frame False {
            n1915 = local write "Comments:"(w588) -> ()
            n1916 = property on="Comments:" class="Str"("DisabledEnum"=1) -> ()  [unwired: 2 in, 2 out]
          }
          frame True {
            n1917 = property on="Comments:" class="Str"("DisabledEnum"=0) -> ()  [unwired: 2 in, 2 out]
          }
        }
        n1918 = case shown="True" w446 {
          tunnel: w447 -> [w603 _]
          frame False {
            n1919 = local write "New: Length"(w603) -> ()
            n1920 = property on="New: Length" class="DigNum (strict)"("DisabledEnum"=1) -> ()  [unwired: 2 in, 2 out]
          }
          frame True {
            n1921 = property on="New: Length" class="DigNum (strict)"("DisabledEnum"=0) -> ()  [unwired: 2 in, 2 out]
          }
        }
        n1922 = case shown="True" w445 {
          tunnel: w444 -> [w600 _]
          frame False {
            n1923 = local write "New: Dielectric"(w600) -> ()
            n1924 = property on="New: Dielectric" class="DigNum (strict)"("DisabledEnum"=1) -> ()  [unwired: 2 in, 2 out]
          }
          frame True {
            n1925 = property on="New: Dielectric" class="DigNum (strict)"("DisabledEnum"=0) -> ()  [unwired: 2 in, 2 out]
          }
        }
      }
    }
  }
  n1926 = Build Array("DeviceID", "Fabricator", "Deposition", "Date", "Sample", "Row", "Column", "L (um)", "W (um)", "Material", "Treatment", "TC (mM)", "Solvent", "C (%)", "ST (C)", "Drops", "Wait (s)", "RT (F)", "RH (%)", "Ramp (s)", "RPM", "Accel (RPM/s)", "Time (s)", "Mobility", "On/Off", "Vt", "S.T.S") -> (→"Transformer \nHeaders":string[])
